vi "Demo.vi"() -> ()   [LabVIEW 2020]
uses:
  TypeDef/Plane.ctl
panel:
  out "string":string
  in  "current lon":string="-79.541260"
  in  "current lat":string="40.286792"
  in  "Current Map":refnum<k7>(container)
  out "Airplanes":T1[](array[typedef])
  out "Raw data":string[][](array[string])
  in  "Airplane":T1
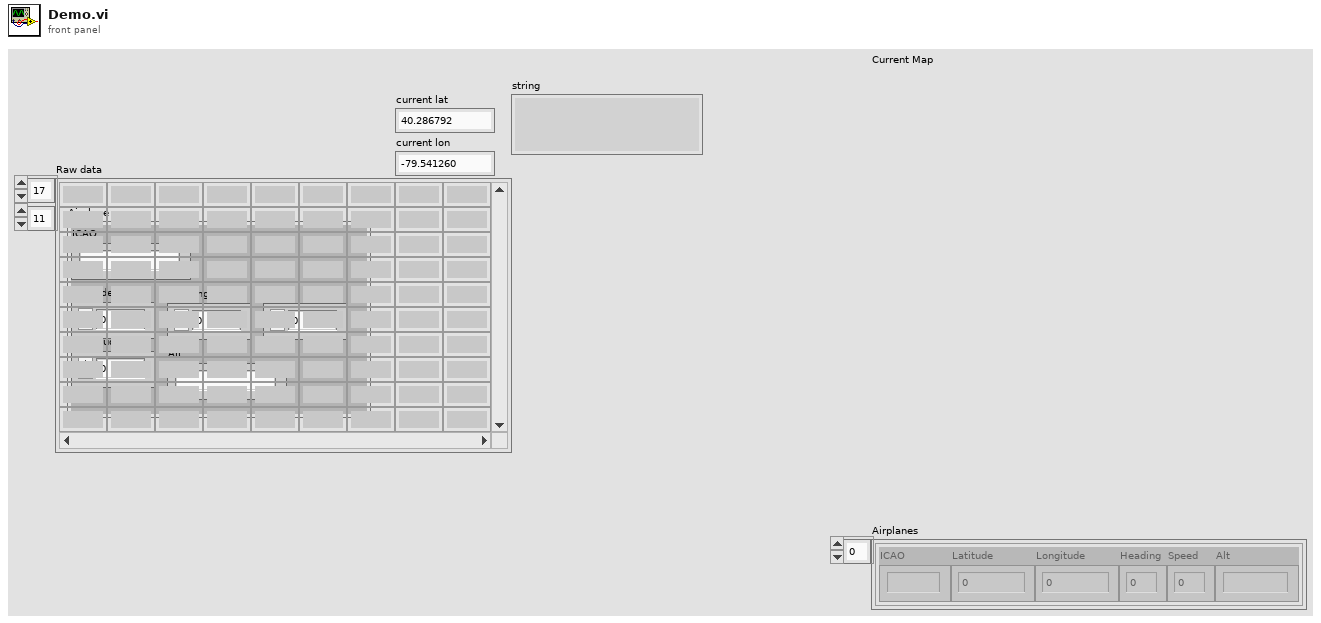
[diagram p1: front panel]
types:
  T1 = typedef "Plane.ctl" = cluster{"ICAO":string, "Latitude":dbl, "Longitude":dbl, "Heading":dbl, "Speed":dbl, "Alt":string}
  T2 = cluster{"ViewerLat":string, "ViewerLong":string, "ViewerAlt":string, "ViewerHDG":string, "Viewerpitch":string}
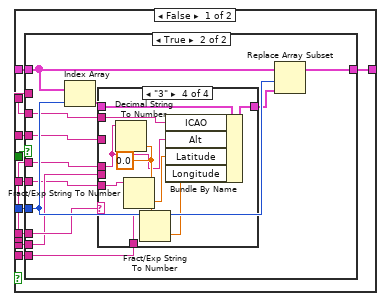
[diagram p6: hidden frame]
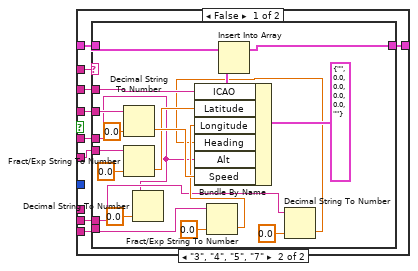
[diagram p7: hidden frame]
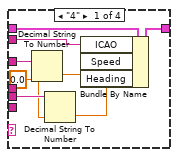
[diagram p9: hidden frame]
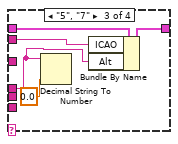
[diagram p11: hidden frame]
diagram:
  (unwired) ",{\"longitude\":0.000000,\"latitude\":0.000000,\"height\":,\"ICAO\":A05514},{\"longitude\":-79.645510,\"latitude\":39.757100,\"height\":39000,\"ICAO\":A4DD8F}" ("string")
  (unwired) "&markers=&markers=icon:https://icons.iconarchive.com/icons/unclebob/spanish-travel/24/plane-icon.png|40.366792,-80.261260" ("string")
  (unwired) "&markers=icon:https://icons.iconarchive.com/icons/unclebob/spanish-travel/24/plane-icon.png|" ("string")
  (unwired) "&markers=icon:https://icons.iconarchive.com/icons/ahmadhania/spherical/64/airplane-icon.png|" ("string")
  (unwired) "&markers=icon:https://icons.iconarchive.com/icons/graphicloads/folded/24/plane-folded-icon.png|" ("string")
  (unwired) "&markers=icon:https://icons.iconarchive.com/icons/papirus-team/papirus-status/24/airplane-mode-icon.png|" ("string")
  (unwired) "&markers=icon:\"file:///C:/Users/Kaitie/Downloads/aeroplane64.png\"%7C" ("string")
  (unwired) string[][] [["MSG", "7", "111", "11111", "ABAE62", "111111", "2021/06/30", "12:22:06.169", "2021/06/30", "12:22:06.150", "", "36000", "", "", "", "", "", "", "", "", "", "0"], ["MSG", "8", "111", "11111", "ABAE62", "111111", "2021/06/30", "12:22:06.346", "2021/06/30", "12:22:06.346", "", "", "", "", "", "", "", "", "", "", "", "0"], ["MSG", "8", "111", "11111", "ABAE62", "111111", "2021/06/30", "12:22:06.506", "2021/06/30", "12:22:06.478", "", "", "", "", "", "", "", "", "", "", "", "0"], ["MSG", "8", "111", "11111", "ABAE62", "111111", "2021/06/30", "12:22:06.515", "2021/06/30", "12:22:06.479", "", "", "", "", "", "", "", "", "", "", "", "0"], ["MSG", "7", "111", "11111", "ABAE62", "111111", "2021/06/30", "12:22:06.556", "2021/06/30", "12:22:06.543", "", "36000", "", "", "", "", "", "", "", "", "", "0"], ["MSG", "8", "111", "11111", "ABAE62", "111111", "2021/06/30", "12:22:07.101", "2021/06/30", "12:22:07.070", "", "", "", "", "", "", "", "", "", "", "", "0"], ["MSG", "7", "111", "11111", "ABAE62", "111111", "2021/06/30", "12:22:07.289", "2021/06/30", "12:22:07.264", "", "36000", "", "", "", "", "", "", "", "", "", "0"], ["MSG", "7", "111", "11111", "ABAE62", "111111", "2021/06/30", "12:22:07.451", "2021/06/30", "12:22:07.395", "", "36000", "", "", "", "", "", "", "", "", "", "0"], ["MSG", "8", "111", "11111", "ABAE62", "111111", "2021/06/30", "12:22:07.568", "2021/06/30", "12:22:07.527", "", "", "", "", "", "", "", "", "", "", "", "0"], ["MSG", "8", "111", "11111", "ABAE62", "111111", "2021/06/30", "12:22:07.578", "2021/06/30", "12:22:07.528", "", "", "", "", "", "", "", "", "", "", "", "0"], ["MSG", "8", "111", "11111", "ABAE62", "111111", "2021/06/30", "12:22:07.830", "2021/06/30", "12:22:07.789", "", "", "", "", "", "", "", "", "", "", "", "0"], ["MSG", "3", "111", "11111", "ABAE62", "111111", "2021/06/30", "12:22:07.997", "2021/06/30", "12:22:07.985", "", "36000", "", "", "40.36748", "-80.25311", "", "", "", "", "", "0"], ["MSG", "8", "111", "11111", "ABAE62", "111111", "2021/06/30", "12:22:08.045", "2021/06/30", "12:22:07.987", "", "", "", "", "", "", "", "", "", "", "", "0"], ["MSG", "8", "111", "11111", "ABAE62", "111111", "2021/06/30", "12:22:08.188", "2021/06/30", "12:22:08.181", "", "", "", "", "", "", "", "", "", "", "", "0"], ["MSG", "8", "111", "11111", "ABAE62", "111111", "2021/06/30", "12:22:08.197", "2021/06/30", "12:22:08.181", "", "", "", "", "", "", "", "", "", "", "", "0"], ["MSG", "7", "111", "11111", "ABAE62", "111111", "2021/06/30", "12:22:08.339", "2021/06/30", "12:22:08.315", "", "36000", "", "", "", "", "", "", "", "", "", "0"], ["MSG", "8", "111", "11111", "ABAE62", "111111", "2021/06/30", "12:22:09.700", "2021/06/30", "12:22:09.689", "", "", "", "", "", "", "", "", "", "", "", "0"], ["MSG", "8", "111", "11111", "ABAE62", "111111", "2021/06/30", "12:22:09.709", "2021/06/30", "12:22:09.689", "", "", "", "", "", "", "", "", "", "", "", "0"], ["MSG", "8", "111", "11111", "ABAE62", "111111", "2021/06/30", "12:22:10.016", "2021/06/30", "12:22:10.016", "", "", "", "", "", "", "", "", "", "", "", "0"], ["MSG", "3", "111", "11111", "ABAE62", "111111", "2021/06/30", "12:22:10.242", "2021/06/30", "12:22:10.214", "", "36000", "", "", "40.36833", "-80.25893", "", "", "", "", "", "0"], ["MSG", "8", "111", "11111", "ABAE62", "111111", "2021/06/30", "12:22:10.368", "2021/06/30", "12:22:10.345", "", "", "", "", "", "", "", "", "", "", "", "0"], ["MSG", "8", "111", "11111", "ABAE62", "111111", "2021/06/30", "12:22:10.602", "2021/06/30", "12:22:10.542", "", "", "", "", "", "", "", "", "", "", "", "0"], ["MSG", "4", "111", "11111", "ABAE62", "111111", "2021/06/30", "12:22:10.703", "2021/06/30", "12:22:10.672", "", "", "437", "281", "", "", "64", "", "", "", "", "0"], ["MSG", "8", "111", "11111", "ABAE62", "111111", "2021/06/30", "12:22:10.942", "2021/06/30", "12:22:10.934", "", "", "", "", "", "", "", "", "", "", "", "0"], ["MSG", "4", "111", "11111", "ABAE62", "111111", "2021/06/30", "12:22:11.735", "2021/06/30", "12:22:11.720", "", "", "437", "281", "", "", "64", "", "", "", "", "0"], ["MSG", "8", "111", "11111", "ABAE62", "111111", "2021/06/30", "12:22:11.902", "2021/06/30", "12:22:11.853", "", "", "", "", "", "", "", "", "", "", "", "0"], ["MSG", "7", "111", "11111", "ABAE62", "111111", "2021/06/30", "12:22:12.170", "2021/06/30", "12:22:12.114", "", "36000", "", "", "", "", "", "", "", "", "", "0"], ["MSG", "8", "111", "11111", "AE0144", "111111", "2021/06/30", "12:22:12.729", "2021/06/30", "12:22:12.704", "", "", "", "", "", "", "", "", "", "", "", "0"], ["MSG", "7", "111", "11111", "AE0144", "111111", "2021/06/30", "12:22:12.797", "2021/06/30", "12:22:12.769", "", "20000", "", "", "", "", "", "", "", "", "", "0"], ["MSG", "7", "111", "11111", "AE0144", "111111", "2021/06/30", "12:22:12.993", "2021/06/30", "12:22:12.966", "", "20000", "", "", "", "", "", "", "", "", "", "0"], ["MSG", "5", "111", "11111", "AE0144", "111111", "2021/06/30", "12:22:13.264", "2021/06/30", "12:22:13.229", "", "20000", "", "", "", "", "", "", "0", "", "0", "0"], ["MSG", "3", "111", "11111", "ABAE62", "111111", "2021/06/30", "12:22:14.038", "2021/06/30", "12:22:14.014", "", "36000", "", "", "40.36977", "-80.26880", "", "", "", "", "", "0"], ["MSG", "5", "111", "11111", "ABAE62", "111111", "2021/06/30", "12:22:14.427", "2021/06/30", "12:22:14.408", "", "36000", "", "", "", "", "", "", "0", "", "0", "0"], ["MSG", "7", "111", "11111", "ABAE62", "111111", "2021/06/30", "12:22:14.859", "2021/06/30", "12:22:14.801", "", "36000", "", "", "", "", "", "", "", "", "", "0"], ["MSG", "8", "111", "11111", "ABAE62", "111111", "2021/06/30", "12:22:14.994", "2021/06/30", "12:22:14.933", "", "", "", "", "", "", "", "", "", "", "", "0"], ["MSG", "8", "111", "11111", "ABAE62", "111111", "2021/06/30", "12:22:15.009", "2021/06/30", "12:22:15.000", "", "", "", "", "", "", "", "", "", "", "", "0"], ["MSG", "8", "111", "11111", "AE0144", "111111", "2021/06/30", "12:22:15.116", "2021/06/30", "12:22:15.064", "", "", "", "", "", "", "", "", "", "", "", "0"], ["MSG", "7", "111", "11111", "ABAE62", "111111", "2021/06/30", "12:22:15.147", "2021/06/30", "12:22:15.128", "", "36000", "", "", "", "", "", "", "", "", "", "0"], ["MSG", "7", "111", "11111", "ABAE62", "111111", "2021/06/30", "12:22:15.405", "2021/06/30", "12:22:15.391", "", "36000", "", "", "", "", "", "", "", "", "", "0"], ["MSG", "8", "111", "11111", "ABAE62", "111111", "2021/06/30", "12:22:15.533", "2021/06/30", "12:22:15.522", "", "", "", "", "", "", "", "", "", "", "", "0"], ["MSG", "8", "111", "11111", "ABAE62", "111111", "2021/06/30", "12:22:15.553", "2021/06/30", "12:22:15.523", "", "", "", "", "", "", "", "", "", "", "", "0"], ["MSG", "7", "111", "11111", "ABAE62", "111111", "2021/06/30", "12:22:15.718", "2021/06/30", "12:22:15.717", "", "36000", "", "", "", "", "", "", "", "", "", "0"]] ("Raw data 2")
  (unwired) "&markers=size:tiny" ("string")
  (unwired) "&markers=color:blue%7Clabel:S%7C" ("string")
  (unwired) "&markers=icon:https://goo.gl/5y3S82|" ("string")
  (unwired) string[][] [["MSG", "4", "111", "11111", "A99703", "111111", "2021/06/30", "01:33:22.831", "2021/06/30", "01:33:22.770", "", "", "213", "266", "", "", "-896", "", "", "", "", "0"], ["MSG", "8", "111", "11111", "A99703", "111111", "2021/06/30", "01:33:23.619", "2021/06/30", "01:33:23.558", "", "", "", "", "", "", "", "", "", "", "", "0"], ["MSG", "3", "111", "11111", "A99703", "111111", "2021/06/30", "01:33:23.658", "2021/06/30", "01:33:23.621", "", "3475", "", "", "40.35814", "-79.71923", "", "", "", "", "", "0"], ["MSG", "4", "111", "11111", "A99703", "111111", "2021/06/30", "01:33:23.760", "2021/06/30", "01:33:23.752", "", "", "213", "266", "", "", "-832", "", "", "", "", "0"], ["MSG", "3", "111", "11111", "A99703", "111111", "2021/06/30", "01:33:24.622", "2021/06/30", "01:33:24.605", "", "3475", "", "", "40.35805", "-79.72052", "", "", "", "", "", "0"], ["MSG", "4", "111", "11111", "A99703", "111111", "2021/06/30", "01:33:24.693", "2021/06/30", "01:33:24.672", "", "", "213", "266", "", "", "-832", "", "", "", "", "0"], ["MSG", "4", "111", "11111", "A99703", "111111", "2021/06/30", "01:33:25.696", "2021/06/30", "01:33:25.654", "", "", "213", "266", "", "", "-768", "", "", "", "", "0"], ["MSG", "1", "111", "11111", "A99703", "111111", "2021/06/30", "01:33:25.766", "2021/06/30", "01:33:25.720", "N717KV  ", "", "", "", "", "", "", "", "", "", "", "0"], ["MSG", "8", "111", "11111", "A99703", "111111", "2021/06/30", "01:33:25.849", "2021/06/30", "01:33:25.850", "", "", "", "", "", "", "", "", "", "", "", "0"], ["MSG", "5", "111", "11111", "A99703", "111111", "2021/06/30", "01:33:26.437", "2021/06/30", "01:33:26.375", "", "345", "", "", "", "", "", "", "", "", "", ""]] ("array")
  w27 = "," ("string")
  (unwired) "https://maps.googleapis.com/maps/api/staticmap?center=Brooklyn+Bridge,New+York,NY&zoom=13&size=600x300&maptype=roadmap\n&markers=color:blue%7Clabel:S%7C40.702147,-74.015794&markers=color:green%7Clabel:G%7C40.711614,-74.012318\n&markers=color:red%7Clabel:C%7C40.718217,-73.998284\n&key=AIzaSyBLVIRyOFRoOpmuxChHO5QT5_7M34SwGWA" ("URL")
  (unwired) string[][] [["MSG", "4", "111", "11111", "A05514", "111111", "2021/06/30", "01:06:18.351", "2021/06/30", "01:06:18.304", "", "", "272", "127", "", "", "0", "", "", "", "", "0"], ["MSG", "8", "111", "11111", "A4DD8F", "111111", "2021/06/30", "01:06:18.874", "2021/06/30", "01:06:18.827", "", "", "", "", "", "", "", "", "", "", "", "0"], ["MSG", "5", "111", "11111", "A4DD8F", "111111", "2021/06/30", "01:06:18.962", "2021/06/30", "01:06:18.957", "", "5000", "", "", "", "", "", "", "0", "", "0", "0"], ["MSG", "5", "111", "11111", "A4DD8F", "111111", "2021/06/30", "01:06:19.109", "2021/06/30", "01:06:19.088", "", "5000", "", "", "", "", "", "", "0", "", "0", "0"], ["MSG", "3", "111", "11111", "A4DD8F", "111111", "2021/06/30", "01:06:19.169", "2021/06/30", "01:06:19.153", "", "5000", "", "", "39.75710", "-79.64551", "", "", "", "", "", "0"], ["MSG", "4", "111", "11111", "A4DD8F", "111111", "2021/06/30", "01:06:19.218", "2021/06/30", "01:06:19.155", "", "", "450", "104", "", "", "0", "", "", "", "", "0"], ["MSG", "8", "111", "11111", "A4DD8F", "111111", "2021/06/30", "01:06:19.628", "2021/06/30", "01:06:19.612", "", "", "", "", "", "", "", "", "", "", "", "0"], ["MSG", "8", "111", "11111", "A4DD8F", "111111", "2021/06/30", "01:06:19.638", "2021/06/30", "01:06:19.613", "", "", "", "", "", "", "", "", "", "", "", "0"], ["MSG", "8", "111", "11111", "A4DD8F", "111111", "2021/06/30", "01:06:19.656", "2021/06/30", "01:06:19.614", "", "", "", "", "", "", "", "", "", "", "", "0"], ["MSG", "8", "111", "11111", "A4DD8F", "111111", "2021/06/30", "01:06:19.669", "2021/06/30", "01:06:19.614", "", "", "", "", "", "", "", "", "", "", "", "0"], ["MSG", "5", "111", "11111", "A4DD8F", "111111", "", "", "", "", "", "", "", "", "", "", "", "", "", "", "", ""]] ("array")
  # "Microsoft Windows [Version 10.0.19042.1052]\n(c) Microsoft Corporation. All rights reserved.\n\nC:\\Data\\dump1090-win.1.10.3010.14>dump1090.exe --interactive --net --net-beast --net-http-port 8081\n-----------------------------------------------------------------------------\n|                        dump1090 ModeS Receiver         Ver : 1.10.3010.14 |\n-----------------------------------------------------------------------------\n\n Copyright (C) 2012 by Salvatore Sanfilippo <antirez@gmail.com>\n Copyright (C) 2014 by Malcolm Robb <support@attavionics.com>\n\n All rights reserved.\n\n THIS SOFTWARE IS PROVIDED BY THE COPYRIGHT HOLDERS AND CONTRIBUTORS\n AS IS AND ANY EXPRESS OR IMPLIED WARRANTIES, INCLUDING, BUT NOT\n LIMITED TO, THE IMPLIED WARRANTIES OF MERCHANTABILITY AND FITNESS FOR\n A PARTICULAR PURPOSE ARE DISCLAIMED. IN NO EVENT SHALL THE COPYRIGHT\n HOLDER OR CONTRIBUTORS BE LIABLE FOR ANY DIRECT, INDIRECT, INCIDENTAL,\n SPECIAL, EXEMPLARY, OR CONSEQUENTIAL DAMAGES (INCLUDING, BUT NOT\n LIMITED TO, PROCUREMENT OF SUBSTITUTE GOODS OR SERVICES; LOSS OF USE,\n DATA, OR PROFITS; OR BUSINESS INTERRUPTION) HOWEVER CAUSED AND ON ANY\n THEORY OF LIABILITY, WHETHER IN CONTRACT, STRICT LIABILITY, OR TORT\n (INCLUDING NEGLIGENCE OR OTHERWISE) ARISING IN ANY WAY OUT OF THE USE\n OF THIS SOFTWARE, EVEN IF ADVISED OF THE POSSIBILITY OF SUCH DAMAGE.\n\n For further details refer to <https://github.com/MalcolmRobb/dump1090>\n\nHex     Mode  Sqwk  Flight   Alt    Spd  Hdg    Lat      Long   Sig  Msgs   Ti/\n-------------------------------------------------------------------------------\nHex     Mode  Sqwk  Flight   Alt    Spd  Hdg    Lat      Long   Sig  Msgs   Ti-\n-------------------------------------------------------------------------------\nHex     Mode  Sqwk  Flight   Alt    Spd  Hdg    Lat      Long   Sig  Msgs   Ti-\n-------------------------------------------------------------------------------\nHex     Mode  Sqwk  Flight   Alt    Spd  Hdg    Lat      Long   Sig  Msgs   Ti-\n-------------------------------------------------------------------------------\nHex     Mode  Sqwk  Flight   Alt    Spd  Hdg    Lat      Long   Sig  Msgs   Ti-\n-------------------------------------------------------------------------------\nHex     Mode  Sqwk  Flight   Alt    Spd  Hdg    Lat      Long   Sig  Msgs   Ti\\\n-------------------------------------------------------------------------------\nHex     Mode  Sqwk  Flight   Alt    Spd  Hdg    Lat      Long   Sig  Msgs   Ti\\\n-------------------------------------------------------------------------------\nHex     Mode  Sqwk  Flight   Alt    Spd  Hdg    Lat      Long   Sig  Msgs   Ti\\\n-------------------------------------------------------------------------------\nHex     Mode  Sqwk  Flight   Alt    Spd  Hdg    Lat      Long   Sig  Msgs   Ti\\\n-------------------------------------------------------------------------------\nHex     Mode  Sqwk  Flight   Alt    Spd  Hdg    Lat      Long   Sig  Msgs   Ti|\n-------------------------------------------------------------------------------\nHex     Mode  Sqwk  Flight   Alt    Spd  Hdg    Lat      Long   Sig  Msgs   Ti|\n-------------------------------------------------------------------------------\nHex     Mode  Sqwk  Flight   Alt    Spd  Hdg    Lat      Long   Sig  Msgs   Ti|\n-------------------------------------------------------------------------------\nHex     Mode  Sqwk  Flight   Alt    Spd  Hdg    Lat      Long   Sig  Msgs   Ti|\n-------------------------------------------------------------------------------\nHex     Mode  Sqwk  Flight   Alt    Spd  Hdg    Lat      Long   Sig  Msgs   Ti/\n-------------------------------------------------------------------------------\nHex     Mode  Sqwk  Flight   Alt    Spd  Hdg    Lat      Long   Sig  Msgs   Ti/\n-------------------------------------------------------------------------------\nHex     Mode  Sqwk  Flight   Alt    Spd  Hdg    Lat      Long   Sig  Msgs   Ti/\n-------------------------------------------------------------------------------\nHex     Mode  Sqwk  Flight   Alt    Spd  Hdg    Lat      Long   Sig  Msgs   Ti/\n-------------------------------------------------------------------------------\nHex     Mode  Sqwk  Flight   Alt    Spd  Hdg    Lat      Long   Sig  Msgs   Ti-\n-------------------------------------------------------------------------------\nHex     Mode  Sqwk  Flight   Alt    Spd  Hdg    Lat      Long   Sig  Msgs   Ti-\n-------------------------------------------------------------------------------\nHex     Mode  Sqwk  Flight   Alt    Spd  Hdg    Lat      Long   Sig  Msgs   Ti-\n-------------------------------------------------------------------------------\nHex     Mode  Sqwk  Flight   Alt    Spd  Hdg    Lat      Long   Sig  Msgs   Ti\\\n-------------------------------------------------------------------------------\nHex     Mode  Sqwk  Flight   Alt    Spd  Hdg    Lat      Long   Sig  Msgs   Ti\\\n-------------------------------------------------------------------------------\nHex     Mode  Sqwk  Flight   Alt    Spd  Hdg    Lat      Long   Sig  Msgs   Ti\\\n-------------------------------------------------------------------------------\nHex     Mode  Sqwk  Flight   Alt    Spd  Hdg    Lat      Long   Sig  Msgs   Ti\\\n-------------------------------------------------------------------------------\nHex     Mode  Sqwk  Flight   Alt    Spd  Hdg    Lat      Long   Sig  Msgs   Ti|\n-------------------------------------------------------------------------------\nHex     Mode  Sqwk  Flight   Alt    Spd  Hdg    Lat      Long   Sig  Msgs   Ti|\n-------------------------------------------------------------------------------\nHex     Mode  Sqwk  Flight   Alt    Spd  Hdg    Lat      Long   Sig  Msgs   Ti|\n-------------------------------------------------------------------------------\nHex     Mode  Sqwk  Flight   Alt    Spd  Hdg    Lat      Long   Sig  Msgs   Ti|\n-------------------------------------------------------------------------------\nHex     Mode  Sqwk  Flight   Alt    Spd  Hdg    Lat      Long   Sig  Msgs   Ti/\n-------------------------------------------------------------------------------\nHex     Mode  Sqwk  Flight   Alt    Spd  Hdg    Lat      Long   Sig  Msgs   Ti/\n-------------------------------------------------------------------------------\nHex     Mode  Sqwk  Flight   Alt    Spd  Hdg    Lat      Long   Sig  Msgs   Ti/\n-------------------------------------------------------------------------------\nHex     Mode  Sqwk  Flight   Alt    Spd  Hdg    Lat      Long   Sig  Msgs   Ti/\n-------------------------------------------------------------------------------\nHex     Mode  Sqwk  Flight   Alt    Spd  Hdg    Lat      Long   Sig  Msgs   Ti-\n-------------------------------------------------------------------------------\nHex     Mode  Sqwk  Flight   Alt    Spd  Hdg    Lat      Long   Sig  Msgs   Ti-\n-------------------------------------------------------------------------------\nHex     Mode  Sqwk  Flight   Alt    Spd  Hdg    Lat      Long   Sig  Msgs   Ti-\n-------------------------------------------------------------------------------\nHex     Mode  Sqwk  Flight   Alt    Spd  Hdg    Lat      Long   Sig  Msgs   Ti-\n-------------------------------------------------------------------------------\nHex     Mode  Sqwk  Flight   Alt    Spd  Hdg    Lat      Long   Sig  Msgs   Ti\\\n-------------------------------------------------------------------------------\nHex     Mode  Sqwk  Flight   Alt    Spd  Hdg    Lat      Long   Sig  Msgs   Ti\\\n-------------------------------------------------------------------------------\nHex     Mode  Sqwk  Flight   Alt    Spd  Hdg    Lat      Long   Sig  Msgs   Ti\\\n-------------------------------------------------------------------------------\nHex     Mode  Sqwk  Flight   Alt    Spd  Hdg    Lat      Long   Sig  Msgs   Ti\\\n-------------------------------------------------------------------------------\nHex     Mode  Sqwk  Flight   Alt    Spd  Hdg    Lat      Long   Sig  Msgs   Ti|\n-------------------------------------------------------------------------------\nHex     Mode  Sqwk  Flight   Alt    Spd  Hdg    Lat      Long   Sig  Msgs   Ti|\n-------------------------------------------------------------------------------\nHex     Mode  Sqwk  Flight   Alt    Spd  Hdg    Lat      Long   Sig  Msgs   Ti|\n-------------------------------------------------------------------------------\nHex     Mode  Sqwk  Flight   Alt    Spd  Hdg    Lat      Long   Sig  Msgs   Ti/\n-------------------------------------------------------------------------------\nHex     Mode  Sqwk  Flight   Alt    Spd  Hdg    Lat      Long   Sig  Msgs   Ti/\n-------------------------------------------------------------------------------\nHex     Mode  Sqwk  Flight   Alt    Spd  Hdg    Lat      Long   Sig  Msgs   Ti/\n-------------------------------------------------------------------------------\nHex     Mode  Sqwk  Flight   Alt    Spd  Hdg    Lat      Long   Sig  Msgs   Ti/\n-------------------------------------------------------------------------------\nHex     Mode  Sqwk  Flight   Alt    Spd  Hdg    Lat      Long   Sig  Msgs   Ti-\n-------------------------------------------------------------------------------\nHex     Mode  Sqwk  Flight   Alt    Spd  Hdg    Lat      Long   Sig  Msgs   Ti-\n-------------------------------------------------------------------------------\nHex     Mode  Sqwk  Flight   Alt    Spd  Hdg    Lat      Long   Sig  Msgs   Ti-\n-------------------------------------------------------------------------------\nHex     Mode  Sqwk  Flight   Alt    Spd  Hdg    Lat      Long   Sig  Msgs   Ti-\n-------------------------------------------------------------------------------\nHex     Mode  Sqwk  Flight   Alt    Spd  Hdg    Lat      Long   Sig  Msgs   Ti\\\n-------------------------------------------------------------------------------\nHex     Mode  Sqwk  Flight   Alt    Spd  Hdg    Lat      Long   Sig  Msgs   Ti\\\n-------------------------------------------------------------------------------\nHex     Mode  Sqwk  Flight   Alt    Spd  Hdg    Lat      Long   Sig  Msgs   Ti\\\n-------------------------------------------------------------------------------\nHex     Mode  Sqwk  Flight   Alt    Spd  Hdg    Lat      Long   Sig  Msgs   Ti\\\n-------------------------------------------------------------------------------\nHex     Mode  Sqwk  Flight   Alt    Spd  Hdg    Lat      Long   Sig  Msgs   Ti|\n-------------------------------------------------------------------------------\nHex     Mode  Sqwk  Flight   Alt    Spd  Hdg    Lat      Long   Sig  Msgs   Ti|\n-------------------------------------------------------------------------------\nHex     Mode  Sqwk  Flight   Alt    Spd  Hdg    Lat      Long   Sig  Msgs   Ti|\n-------------------------------------------------------------------------------\nHex     Mode  Sqwk  Flight   Alt    Spd  Hdg    Lat      Long   Sig  Msgs   Ti|\n-------------------------------------------------------------------------------\nHex     Mode  Sqwk  Flight   Alt    Spd  Hdg    Lat      Long   Sig  Msgs   Ti/\n-------------------------------------------------------------------------------\nHex     Mode  Sqwk  Flight   Alt    Spd  Hdg    Lat      Long   Sig  Msgs   Ti/\n-------------------------------------------------------------------------------\nHex     Mode  Sqwk  Flight   Alt    Spd  Hdg    Lat      Long   Sig  Msgs   Ti/\n-------------------------------------------------------------------------------\nHex     Mode  Sqwk  Flight   Alt    Spd  Hdg    Lat      Long   Sig  Msgs   Ti-\n-------------------------------------------------------------------------------\nHex     Mode  Sqwk  Flight   Alt    Spd  Hdg    Lat      Long   Sig  Msgs   Ti-\n-------------------------------------------------------------------------------\nHex     Mode  Sqwk  Flight   Alt    Spd  Hdg    Lat      Long   Sig  Msgs   Ti-\n-------------------------------------------------------------------------------\nHex     Mode  Sqwk  Flight   Alt    Spd  Hdg    Lat      Long   Sig  Msgs   Ti-\n-------------------------------------------------------------------------------\nHex     Mode  Sqwk  Flight   Alt    Spd  Hdg    Lat      Long   Sig  Msgs   Ti\\\n-------------------------------------------------------------------------------\nHex     Mode  Sqwk  Flight   Alt    Spd  Hdg    Lat      Long   Sig  Msgs   Ti\\\n-------------------------------------------------------------------------------\nHex     Mode  Sqwk  Flight   Alt    Spd  Hdg    Lat      Long   Sig  Msgs   Ti\\\n-------------------------------------------------------------------------------\nHex     Mode  Sqwk  Flight   Alt    Spd  Hdg    Lat      Long   Sig  Msgs   Ti\\\n-------------------------------------------------------------------------------\nHex     Mode  Sqwk  Flight   Alt    Spd  Hdg    Lat      Long   Sig  Msgs   Ti|\n-------------------------------------------------------------------------------\nHex     Mode  Sqwk  Flight   Alt    Spd  Hdg    Lat      Long   Sig  Msgs   Ti|\n-------------------------------------------------------------------------------\nHex     Mode  Sqwk  Flight   Alt    Spd  Hdg    Lat      Long   Sig  Msgs   Ti|\n-------------------------------------------------------------------------------\nHex     Mode  Sqwk  Flight   Alt    Spd  Hdg    Lat      Long   Sig  Msgs   Ti|\n-------------------------------------------------------------------------------\nHex     Mode  Sqwk  Flight   Alt    Spd  Hdg    Lat      Long   Sig  Msgs   Ti/\n-------------------------------------------------------------------------------\nHex     Mode  Sqwk  Flight   Alt    Spd  Hdg    Lat      Long   Sig  Msgs   Ti/\n-------------------------------------------------------------------------------\nHex     Mode  Sqwk  Flight   Alt    Spd  Hdg    Lat      Long   Sig  Msgs   Ti/\n-------------------------------------------------------------------------------\nHex     Mode  Sqwk  Flight   Alt    Spd  Hdg    Lat      Long   Sig  Msgs   Ti/\n-------------------------------------------------------------------------------\nHex     Mode  Sqwk  Flight   Alt    Spd  Hdg    Lat      Long   Sig  Msgs   Ti-\n-------------------------------------------------------------------------------\nHex     Mode  Sqwk  Flight   Alt    Spd  Hdg    Lat      Long   Sig  Msgs   Ti-\n-------------------------------------------------------------------------------\nHex     Mode  Sqwk  Flight   Alt    Spd  Hdg    Lat      Long   Sig  Msgs   Ti-\n-------------------------------------------------------------------------------\nHex     Mode  Sqwk  Flight   Alt    Spd  Hdg    Lat      Long   Sig  Msgs   Ti-\n-------------------------------------------------------------------------------\nHex     Mode  Sqwk  Flight   Alt    Spd  Hdg    Lat      Long   Sig  Msgs   Ti\\\n-------------------------------------------------------------------------------\nHex     Mode  Sqwk  Flight   Alt    Spd  Hdg    Lat      Long   Sig  Msgs   Ti\\\n-------------------------------------------------------------------------------\nHex     Mode  Sqwk  Flight   Alt    Spd  Hdg    Lat      Long   Sig  Msgs   Ti\\\n-------------------------------------------------------------------------------\nHex     Mode  Sqwk  Flight   Alt    Spd  Hdg    Lat      Long   Sig  Msgs   Ti|\n-------------------------------------------------------------------------------\nHex     Mode  Sqwk  Flight   Alt    Spd  Hdg    Lat      Long   Sig  Msgs   Ti|\n-------------------------------------------------------------------------------\nHex     Mode  Sqwk  Flight   Alt    Spd  Hdg    Lat      Long   Sig  Msgs   Ti|\n-------------------------------------------------------------------------------\nHex     Mode  Sqwk  Flight   Alt    Spd  Hdg    Lat      Long   Sig  Msgs   Ti|\n-------------------------------------------------------------------------------\nHex     Mode  Sqwk  Flight   Alt    Spd  Hdg    Lat      Long   Sig  Msgs   Ti/\n-------------------------------------------------------------------------------\nHex     Mode  Sqwk  Flight   Alt    Spd  Hdg    Lat      Long   Sig  Msgs   Ti/\n-------------------------------------------------------------------------------\nHex     Mode  Sqwk  Flight   Alt    Spd  Hdg    Lat      Long   Sig  Msgs   Ti/\n-------------------------------------------------------------------------------\nHex     Mode  Sqwk  Flight   Alt    Spd  Hdg    Lat      Long   Sig  Msgs   Ti/\n-------------------------------------------------------------------------------\nHex     Mode  Sqwk  Flight   Alt    Spd  Hdg    Lat      Long   Sig  Msgs   Ti-\n-------------------------------------------------------------------------------\nHex     Mode  Sqwk  Flight   Alt    Spd  Hdg    Lat      Long   Sig  Msgs   Ti-\n-------------------------------------------------------------------------------\nHex     Mode  Sqwk  Flight   Alt    Spd  Hdg    Lat      Long   Sig  Msgs   Ti-\n-------------------------------------------------------------------------------\nHex     Mode  Sqwk  Flight   Alt    Spd  Hdg    Lat      Long   Sig  Msgs   Ti-\n-------------------------------------------------------------------------------\nHex     Mode  Sqwk  Flight   Alt    Spd  Hdg    Lat      Long   Sig  Msgs   Ti\\\n-------------------------------------------------------------------------------\nHex     Mode  Sqwk  Flight   Alt    Spd  Hdg    Lat      Long   Sig  Msgs   Ti\\\n-------------------------------------------------------------------------------\nHex     Mode  Sqwk  Flight   Alt    Spd  Hdg    Lat      Long   Sig  Msgs   Ti\\\n-------------------------------------------------------------------------------\nHex     Mode  Sqwk  Flight   Alt    Spd  Hdg    Lat      Long   Sig  Msgs   Ti\\\n-------------------------------------------------------------------------------\nHex     Mode  Sqwk  Flight   Alt    Spd  Hdg    Lat      Long   Sig  Msgs   Ti|\n-------------------------------------------------------------------------------\nHex     Mode  Sqwk  Flight   Alt    Spd  Hdg    Lat      Long   Sig  Msgs   Ti|\n-------------------------------------------------------------------------------\nHex     Mode  Sqwk  Flight   Alt    Spd  Hdg    Lat      Long   Sig  Msgs   Ti|\n-------------------------------------------------------------------------------\nHex     Mode  Sqwk  Flight   Alt    Spd  Hdg    Lat      Long   Sig  Msgs   Ti/\n-------------------------------------------------------------------------------\nHex     Mode  Sqwk  Flight   Alt    Spd  Hdg    Lat      Long   Sig  Msgs   Ti/\n-------------------------------------------------------------------------------\nHex     Mode  Sqwk  Flight   Alt    Spd  Hdg    Lat      Long   Sig  Msgs   Ti/\n-------------------------------------------------------------------------------\nHex     Mode  Sqwk  Flight   Alt    Spd  Hdg    Lat      Long   Sig  Msgs   Ti/\n-------------------------------------------------------------------------------\nHex     Mode  Sqwk  Flight   Alt    Spd  Hdg    Lat      Long   Sig  Msgs   Ti-\n-------------------------------------------------------------------------------\nHex     Mode  Sqwk  Flight   Alt    Spd  Hdg    Lat      Long   Sig  Msgs   Ti-\n-------------------------------------------------------------------------------\nHex     Mode  Sqwk  Flight   Alt    Spd  Hdg    Lat      Long   Sig  Msgs   Ti-\n-------------------------------------------------------------------------------\nHex     Mode  Sqwk  Flight   Alt    Spd  Hdg    Lat      Long   Sig  Msgs   Ti-\n-------------------------------------------------------------------------------\nHex     Mode  Sqwk  Flight   Alt    Spd  Hdg    Lat      Long   Sig  Msgs   Ti\\\n-------------------------------------------------------------------------------\nHex     Mode  Sqwk  Flight   Alt    Spd  Hdg    Lat      Long   Sig  Msgs   Ti\\\n-------------------------------------------------------------------------------\nHex     Mode  Sqwk  Flight   Alt    Spd  Hdg    Lat      Long   Sig  Msgs   Ti\\\n-------------------------------------------------------------------------------\nHex     Mode  Sqwk  Flight   Alt    Spd  Hdg    Lat      Long   Sig  Msgs   Ti\\\n-------------------------------------------------------------------------------\nHex     Mode  Sqwk  Flight   Alt    Spd  Hdg    Lat      Long   Sig  Msgs   Ti|\n-------------------------------------------------------------------------------\nHex     Mode  Sqwk  Flight   Alt    Spd  Hdg    Lat      Long   Sig  Msgs   Ti|\n-------------------------------------------------------------------------------\nHex     Mode  Sqwk  Flight   Alt    Spd  Hdg    Lat      Long   Sig  Msgs   Ti|\n-------------------------------------------------------------------------------\nHex     Mode  Sqwk  Flight   Alt    Spd  Hdg    Lat      Long   Sig  Msgs   Ti|\n-------------------------------------------------------------------------------\nHex     Mode  Sqwk  Flight   Alt    Spd  Hdg    Lat      Long   Sig  Msgs   Ti/\n-------------------------------------------------------------------------------\nHex     Mode  Sqwk  Flight   Alt    Spd  Hdg    Lat      Long   Sig  Msgs   Ti/\n-------------------------------------------------------------------------------\nHex     Mode  Sqwk  Flight   Alt    Spd  Hdg    Lat      Long   Sig  Msgs   Ti/\n-------------------------------------------------------------------------------\nHex     Mode  Sqwk  Flight   Alt    Spd  Hdg    Lat      Long   Sig  Msgs   Ti-\n-------------------------------------------------------------------------------\nHex     Mode  Sqwk  Flight   Alt    Spd  Hdg    Lat      Long   Sig  Msgs   Ti-\n-------------------------------------------------------------------------------\nHex     Mode  Sqwk  Flight   Alt    Spd  Hdg    Lat      Long   Sig  Msgs   Ti-\n-------------------------------------------------------------------------------\nHex     Mode  Sqwk  Flight   Alt    Spd  Hdg    Lat      Long   Sig  Msgs   Ti-\n-------------------------------------------------------------------------------\nHex     Mode  Sqwk  Flight   Alt    Spd  Hdg    Lat      Long   Sig  Msgs   Ti\\\n-------------------------------------------------------------------------------\nHex     Mode  Sqwk  Flight   Alt    Spd  Hdg    Lat      Long   Sig  Msgs   Ti\\\n-------------------------------------------------------------------------------\nHex     Mode  Sqwk  Flight   Alt    Spd  Hdg    Lat      Long   Sig  Msgs   Ti\\\n-------------------------------------------------------------------------------\nHex     Mode  Sqwk  Flight   Alt    Spd  Hdg    Lat      Long   Sig  Msgs   Ti\\\n-------------------------------------------------------------------------------\nHex     Mode  Sqwk  Flight   Alt    Spd  Hdg    Lat      Long   Sig  Msgs   Ti|\n-------------------------------------------------------------------------------\nHex     Mode  Sqwk  Flight   Alt    Spd  Hdg    Lat      Long   Sig  Msgs   Ti|\n-------------------------------------------------------------------------------\nHex     Mode  Sqwk  Flight   Alt    Spd  Hdg    Lat      Long   Sig  Msgs   Ti|\n-------------------------------------------------------------------------------\nHex     Mode  Sqwk  Flight   Alt    Spd  Hdg    Lat      Long   Sig  Msgs   Ti|\n-------------------------------------------------------------------------------\nHex     Mode  Sqwk  Flight   Alt    Spd  Hdg    Lat      Long   Sig  Msgs   Ti/\n-------------------------------------------------------------------------------\nHex     Mode  Sqwk  Flight   Alt    Spd  Hdg    Lat      Long   Sig  Msgs   Ti/\n-------------------------------------------------------------------------------\nHex     Mode  Sqwk  Flight   Alt    Spd  Hdg    Lat      Long   Sig  Msgs   Ti/\n-------------------------------------------------------------------------------\nHex     Mode  Sqwk  Flight   Alt    Spd  Hdg    Lat      Long   Sig  Msgs   Ti/\n-------------------------------------------------------------------------------\nHex     Mode  Sqwk  Flight   Alt    Spd  Hdg    Lat      Long   Sig  Msgs   Ti-\n-------------------------------------------------------------------------------\nHex     Mode  Sqwk  Flight   Alt    Spd  Hdg    Lat      Long   Sig  Msgs   Ti-\n-------------------------------------------------------------------------------\nHex     Mode  Sqwk  Flight   Alt    Spd  Hdg    Lat      Long   Sig  Msgs   Ti-\n-------------------------------------------------------------------------------\nHex     Mode  Sqwk  Flight   Alt    Spd  Hdg    Lat      Long   Sig  Msgs   Ti-\n-------------------------------------------------------------------------------\nHex     Mode  Sqwk  Flight   Alt    Spd  Hdg    Lat      Long   Sig  Msgs   Ti\\\n-------------------------------------------------------------------------------\nHex     Mode  Sqwk  Flight   Alt    Spd  Hdg    Lat      Long   Sig  Msgs   Ti\\\n-------------------------------------------------------------------------------\nHex     Mode  Sqwk  Flight   Alt    Spd  Hdg    Lat      Long   Sig  Msgs   Ti\\\n-------------------------------------------------------------------------------\nHex     Mode  Sqwk  Flight   Alt    Spd  Hdg    Lat      Long   Sig  Msgs   Ti|\n-------------------------------------------------------------------------------\nHex     Mode  Sqwk  Flight   Alt    Spd  Hdg    Lat      Long   Sig  Msgs   Ti|\n-------------------------------------------------------------------------------\nHex     Mode  Sqwk  Flight   Alt    Spd  Hdg    Lat      Long   Sig  Msgs   Ti|\n-------------------------------------------------------------------------------\nHex     Mode  Sqwk  Flight   Alt    Spd  Hdg    Lat      Long   Sig  Msgs   Ti|\n-------------------------------------------------------------------------------\nHex     Mode  Sqwk  Flight   Alt    Spd  Hdg    Lat      Long   Sig  Msgs   Ti/\n-------------------------------------------------------------------------------\nHex     Mode  Sqwk  Flight   Alt    Spd  Hdg    Lat      Long   Sig  Msgs   Ti/\n-------------------------------------------------------------------------------\nHex     Mode  Sqwk  Flight   Alt    Spd  Hdg    Lat      Long   Sig  Msgs   Ti/\n-------------------------------------------------------------------------------\nHex     Mode  Sqwk  Flight   Alt    Spd  Hdg    Lat      Long   Sig  Msgs   Ti/\n-------------------------------------------------------------------------------\nHex     Mode  Sqwk  Flight   Alt    Spd  Hdg    Lat      Long   Sig  Msgs   Ti-\n-------------------------------------------------------------------------------\nHex     Mode  Sqwk  Flight   Alt    Spd  Hdg    Lat      Long   Sig  Msgs   Ti-\n-------------------------------------------------------------------------------\nHex     Mode  Sqwk  Flight   Alt    Spd  Hdg    Lat      Long   Sig  Msgs   Ti-\n-------------------------------------------------------------------------------\nHex     Mode  Sqwk  Flight   Alt    Spd  Hdg    Lat      Long   Sig  Msgs   Ti-\n-------------------------------------------------------------------------------\nHex     Mode  Sqwk  Flight   Alt    Spd  Hdg    Lat      Long   Sig  Msgs   Ti\\\n-------------------------------------------------------------------------------\nHex     Mode  Sqwk  Flight   Alt    Spd  Hdg    Lat      Long   Sig  Msgs   Ti\\\n-------------------------------------------------------------------------------\nHex     Mode  Sqwk  Flight   Alt    Spd  Hdg    Lat      Long   Sig  Msgs   Ti\\\n-------------------------------------------------------------------------------\nHex     Mode  Sqwk  Flight   Alt    Spd  Hdg    Lat      Long   Sig  Msgs   Ti\\\n-------------------------------------------------------------------------------\nHex     Mode  Sqwk  Flight   Alt    Spd  Hdg    Lat      Long   Sig  Msgs   Ti|\n-------------------------------------------------------------------------------\nHex     Mode  Sqwk  Flight   Alt    Spd  Hdg    Lat      Long   Sig  Msgs   Ti|\n-------------------------------------------------------------------------------\nHex     Mode  Sqwk  Flight   Alt    Spd  Hdg    Lat      Long   Sig  Msgs   Ti|\n-------------------------------------------------------------------------------\nHex     Mode  Sqwk  Flight   Alt    Spd  Hdg    Lat      Long   Sig  Msgs   Ti/\n-------------------------------------------------------------------------------\nHex     Mode  Sqwk  Flight   Alt    Spd  Hdg    Lat      Long   Sig  Msgs   Ti/\n-------------------------------------------------------------------------------\nHex     Mode  Sqwk  Flight   Alt    Spd  Hdg    Lat      Long   Sig  Msgs   Ti/\n-------------------------------------------------------------------------------\nHex     Mode  Sqwk  Flight   Alt    Spd  Hdg    Lat      Long   Sig  Msgs   Ti/\n-------------------------------------------------------------------------------\nHex     Mode  Sqwk  Flight   Alt    Spd  Hdg    Lat      Long   Sig  Msgs   Ti-\n-------------------------------------------------------------------------------\nHex     Mode  Sqwk  Flight   Alt    Spd  Hdg    Lat      Long   Sig  Msgs   Ti-\n-------------------------------------------------------------------------------\nHex     Mode  Sqwk  Flight   Alt    Spd  Hdg    Lat      Long   Sig  Msgs   Ti-\n-------------------------------------------------------------------------------\nHex     Mode  Sqwk  Flight   Alt    Spd  Hdg    Lat      Long   Sig  Msgs   Ti-\n-------------------------------------------------------------------------------\nHex     Mode  Sqwk  Flight   Alt    Spd  Hdg    Lat      Long   Sig  Msgs   Ti\\\n-------------------------------------------------------------------------------\nHex     Mode  Sqwk  Flight   Alt    Spd  Hdg    Lat      Long   Sig  Msgs   Ti\\\n-------------------------------------------------------------------------------\nHex     Mode  Sqwk  Flight   Alt    Spd  Hdg    Lat      Long   Sig  Msgs   Ti\\\n-------------------------------------------------------------------------------\nHex     Mode  Sqwk  Flight   Alt    Spd  Hdg    Lat      Long   Sig  Msgs   Ti\\\n-------------------------------------------------------------------------------\nHex     Mode  Sqwk  Flight   Alt    Spd  Hdg    Lat      Long   Sig  Msgs   Ti|\n-------------------------------------------------------------------------------\nHex     Mode  Sqwk  Flight   Alt    Spd  Hdg    Lat      Long   Sig  Msgs   Ti|\n-------------------------------------------------------------------------------\nHex     Mode  Sqwk  Flight   Alt    Spd  Hdg    Lat      Long   Sig  Msgs   Ti|\n-------------------------------------------------------------------------------\nHex     Mode  Sqwk  Flight   Alt    Spd  Hdg    Lat      Long   Sig  Msgs   Ti|\n-------------------------------------------------------------------------------\nHex     Mode  Sqwk  Flight   Alt    Spd  Hdg    Lat      Long   Sig  Msgs   Ti/\n-------------------------------------------------------------------------------\nHex     Mode  Sqwk  Flight   Alt    Spd  Hdg    Lat      Long   Sig  Msgs   Ti/\n-------------------------------------------------------------------------------\nHex     Mode  Sqwk  Flight   Alt    Spd  Hdg    Lat      Long   Sig  Msgs   Ti/\n-------------------------------------------------------------------------------\nHex     Mode  Sqwk  Flight   Alt    Spd  Hdg    Lat      Long   Sig  Msgs   Ti/\n-------------------------------------------------------------------------------\nHex     Mode  Sqwk  Flight   Alt    Spd  Hdg    Lat      Long   Sig  Msgs   Ti-\n-------------------------------------------------------------------------------\nHex     Mode  Sqwk  Flight   Alt    Spd  Hdg    Lat      Long   Sig  Msgs   Ti-\n-------------------------------------------------------------------------------\nHex     Mode  Sqwk  Flight   Alt    Spd  Hdg    Lat      Long   Sig  Msgs   Ti-\n-------------------------------------------------------------------------------\nHex     Mode  Sqwk  Flight   Alt    Spd  Hdg    Lat      Long   Sig  Msgs   Ti\\\n-------------------------------------------------------------------------------\nHex     Mode  Sqwk  Flight   Alt    Spd  Hdg    Lat      Long   Sig  Msgs   Ti\\\n-------------------------------------------------------------------------------\nHex     Mode  Sqwk  Flight   Alt    Spd  Hdg    Lat      Long   Sig  Msgs   Ti\\\n-------------------------------------------------------------------------------\nHex     Mode  Sqwk  Flight   Alt    Spd  Hdg    Lat      Long   Sig  Msgs   Ti\\\n-------------------------------------------------------------------------------\nHex     Mode  Sqwk  Flight   Alt    Spd  Hdg    Lat      Long   Sig  Msgs   Ti|\n-------------------------------------------------------------------------------\nHex     Mode  Sqwk  Flight   Alt    Spd  Hdg    Lat      Long   Sig  Msgs   Ti|\n-------------------------------------------------------------------------------\nHex     Mode  Sqwk  Flight   Alt    Spd  Hdg    Lat      Long   Sig  Msgs   Ti|\n-------------------------------------------------------------------------------\nHex     Mode  Sqwk  Flight   Alt    Spd  Hdg    Lat      Long   Sig  Msgs   Ti|\n-------------------------------------------------------------------------------\nHex     Mode  Sqwk  Flight   Alt    Spd  Hdg    Lat      Long   Sig  Msgs   Ti/\n-------------------------------------------------------------------------------\nHex     Mode  Sqwk  Flight   Alt    Spd  Hdg    Lat      Long   Sig  Msgs   Ti/\n-------------------------------------------------------------------------------\nHex     Mode  Sqwk  Flight   Alt    Spd  Hdg    Lat      Long   Sig  Msgs   Ti/\n-------------------------------------------------------------------------------\nHex     Mode  Sqwk  Flight   Alt    Spd  Hdg    Lat      Long   Sig  Msgs   Ti/\n-------------------------------------------------------------------------------\nHex     Mode  Sqwk  Flight   Alt    Spd  Hdg    Lat      Long   Sig  Msgs   Ti-\n-------------------------------------------------------------------------------\nHex     Mode  Sqwk  Flight   Alt    Spd  Hdg    Lat      Long   Sig  Msgs   Ti-\n-------------------------------------------------------------------------------\nHex     Mode  Sqwk  Flight   Alt    Spd  Hdg    Lat      Long   Sig  Msgs   Ti-\n-------------------------------------------------------------------------------\nHex     Mode  Sqwk  Flight   Alt    Spd  Hdg    Lat      Long   Sig  Msgs   Ti\\\n-------------------------------------------------------------------------------\nHex     Mode  Sqwk  Flight   Alt    Spd  Hdg    Lat      Long   Sig  Msgs   Ti\\\n-------------------------------------------------------------------------------\nHex     Mode  Sqwk  Flight   Alt    Spd  Hdg    Lat      Long   Sig  Msgs   Ti\\\n-------------------------------------------------------------------------------\nHex     Mode  Sqwk  Flight   Alt    Spd  Hdg    Lat      Long   Sig  Msgs   Ti\\\n-------------------------------------------------------------------------------\nHex     Mode  Sqwk  Flight   Alt    Spd  Hdg    Lat      Long   Sig  Msgs   Ti|\n-------------------------------------------------------------------------------\nHex     Mode  Sqwk  Flight   Alt    Spd  Hdg    Lat      Long   Sig  Msgs   Ti|\n-------------------------------------------------------------------------------\nHex     Mode  Sqwk  Flight   Alt    Spd  Hdg    Lat      Long   Sig  Msgs   Ti|\n-------------------------------------------------------------------------------\nHex     Mode  Sqwk  Flight   Alt    Spd  Hdg    Lat      Long   Sig  Msgs   Ti|\n-------------------------------------------------------------------------------\nHex     Mode  Sqwk  Flight   Alt    Spd  Hdg    Lat      Long   Sig  Msgs   Ti/\n-------------------------------------------------------------------------------\nHex     Mode  Sqwk  Flight   Alt    Spd  Hdg    Lat      Long   Sig  Msgs   Ti/\n-------------------------------------------------------------------------------\nHex     Mode  Sqwk  Flight   Alt    Spd  Hdg    Lat      Long   Sig  Msgs   Ti/\n-------------------------------------------------------------------------------\nHex     Mode  Sqwk  Flight   Alt    Spd  Hdg    Lat      Long   Sig  Msgs   Ti/\n-------------------------------------------------------------------------------\nHex     Mode  Sqwk  Flight   Alt    Spd  Hdg    Lat      Long   Sig  Msgs   Ti-\n-------------------------------------------------------------------------------\nHex     Mode  Sqwk  Flight   Alt    Spd  Hdg    Lat      Long   Sig  Msgs   Ti-\n-------------------------------------------------------------------------------\nHex     Mode  Sqwk  Flight   Alt    Spd  Hdg    Lat      Long   Sig  Msgs   Ti-\n-------------------------------------------------------------------------------\nHex     Mode  Sqwk  Flight   Alt    Spd  Hdg    Lat      Long   Sig  Msgs   Ti-\n-------------------------------------------------------------------------------\nHex     Mode  Sqwk  Flight   Alt    Spd  Hdg    Lat      Long   Sig  Msgs   Ti\\\n-------------------------------------------------------------------------------\nHex     Mode  Sqwk  Flight   Alt    Spd  Hdg    Lat      Long   Sig  Msgs   Ti\\\n-------------------------------------------------------------------------------\nHex     Mode  Sqwk  Flight   Alt    Spd  Hdg    Lat      Long   Sig  Msgs   Ti\\\n-------------------------------------------------------------------------------\nHex     Mode  Sqwk  Flight   Alt    Spd  Hdg    Lat      Long   Sig  Msgs   Ti|\n-------------------------------------------------------------------------------\nHex     Mode  Sqwk  Flight   Alt    Spd  Hdg    Lat      Long   Sig  Msgs   Ti|\n-------------------------------------------------------------------------------\nHex     Mode  Sqwk  Flight   Alt    Spd  Hdg    Lat      Long   Sig  Msgs   Ti|\n-------------------------------------------------------------------------------\nHex     Mode  Sqwk  Flight   Alt    Spd  Hdg    Lat      Long   Sig  Msgs   Ti|\n-------------------------------------------------------------------------------\nHex     Mode  Sqwk  Flight   Alt    Spd  Hdg    Lat      Long   Sig  Msgs   Ti/\n-------------------------------------------------------------------------------\nHex     Mode  Sqwk  Flight   Alt    Spd  Hdg    Lat      Long   Sig  Msgs   Ti/\n-------------------------------------------------------------------------------\nHex     Mode  Sqwk  Flight   Alt    Spd  Hdg    Lat      Long   Sig  Msgs   Ti/\n-------------------------------------------------------------------------------\nHex     Mode  Sqwk  Flight   Alt    Spd  Hdg    Lat      Long   Sig  Msgs   Ti/\n-------------------------------------------------------------------------------\nHex     Mode  Sqwk  Flight   Alt    Spd  Hdg    Lat      Long   Sig  Msgs   Ti-\n-------------------------------------------------------------------------------\nHex     Mode  Sqwk  Flight   Alt    Spd  Hdg    Lat      Long   Sig  Msgs   Ti-\n-------------------------------------------------------------------------------\nHex     Mode  Sqwk  Flight   Alt    Spd  Hdg    Lat      Long   Sig  Msgs   Ti-\n-------------------------------------------------------------------------------\nHex     Mode  Sqwk  Flight   Alt    Spd  Hdg    Lat      Long   Sig  Msgs   Ti-\n-------------------------------------------------------------------------------\nHex     Mode  Sqwk  Flight   Alt    Spd  Hdg    Lat      Long   Sig  Msgs   Ti\\\n-------------------------------------------------------------------------------\nHex     Mode  Sqwk  Flight   Alt    Spd  Hdg    Lat      Long   Sig  Msgs   Ti\\\n-------------------------------------------------------------------------------\nHex     Mode  Sqwk  Flight   Alt    Spd  Hdg    Lat      Long   Sig  Msgs   Ti\\\n-------------------------------------------------------------------------------\nHex     Mode  Sqwk  Flight   Alt    Spd  Hdg    Lat      Long   Sig  Msgs   Ti\\\n-------------------------------------------------------------------------------\nHex     Mode  Sqwk  Flight   Alt    Spd  Hdg    Lat      Long   Sig  Msgs   Ti|\n-------------------------------------------------------------------------------\nHex     Mode  Sqwk  Flight   Alt    Spd  Hdg    Lat      Long   Sig  Msgs   Ti|\n-------------------------------------------------------------------------------\nHex     Mode  Sqwk  Flight   Alt    Spd  Hdg    Lat      Long   Sig  Msgs   Ti|\n-------------------------------------------------------------------------------\nHex     Mode  Sqwk  Flight   Alt    Spd  Hdg    Lat      Long   Sig  Msgs   Ti/\n-------------------------------------------------------------------------------\nHex     Mode  Sqwk  Flight   Alt    Spd  Hdg    Lat      Long   Sig  Msgs   Ti/\n-------------------------------------------------------------------------------\nHex     Mode  Sqwk  Flight   Alt    Spd  Hdg    Lat      Long   Sig  Msgs   Ti/\n-------------------------------------------------------------------------------\nHex     Mode  Sqwk  Flight   Alt    Spd  Hdg    Lat      Long   Sig  Msgs   Ti/\n-------------------------------------------------------------------------------\nHex     Mode  Sqwk  Flight   Alt    Spd  Hdg    Lat      Long   Sig  Msgs   Ti-\n-------------------------------------------------------------------------------\nHex     Mode  Sqwk  Flight   Alt    Spd  Hdg    Lat      Long   Sig  Msgs   Ti-\n-------------------------------------------------------------------------------\nHex     Mode  Sqwk  Flight   Alt    Spd  Hdg    Lat      Long   Sig  Msgs   Ti-\n-------------------------------------------------------------------------------\nHex     Mode  Sqwk  Flight   Alt    Spd  Hdg    Lat      Long   Sig  Msgs   Ti-\n-------------------------------------------------------------------------------\nHex     Mode  Sqwk  Flight   Alt    Spd  Hdg    Lat      Long   Sig  Msgs   Ti\\\n-------------------------------------------------------------------------------\nHex     Mode  Sqwk  Flight   Alt    Spd  Hdg    Lat      Long   Sig  Msgs   Ti\\\n-------------------------------------------------------------------------------\nHex     Mode  Sqwk  Flight   Alt    Spd  Hdg    Lat      Long   Sig  Msgs   Ti\\\n-------------------------------------------------------------------------------\nHex     Mode  Sqwk  Flight   Alt    Spd  Hdg    Lat      Long   Sig  Msgs   Ti\\\n-------------------------------------------------------------------------------\nHex     Mode  Sqwk  Flight   Alt    Spd  Hdg    Lat      Long   Sig  Msgs   Ti|\n-------------------------------------------------------------------------------\nHex     Mode  Sqwk  Flight   Alt    Spd  Hdg    Lat      Long   Sig  Msgs   Ti|\n-------------------------------------------------------------------------------\nHex     Mode  Sqwk  Flight   Alt    Spd  Hdg    Lat      Long   Sig  Msgs   Ti|\n-------------------------------------------------------------------------------\nHex     Mode  Sqwk  Flight   Alt    Spd  Hdg    Lat      Long   Sig  Msgs   Ti|\n-------------------------------------------------------------------------------\nHex     Mode  Sqwk  Flight   Alt    Spd  Hdg    Lat      Long   Sig  Msgs   Ti/\n-------------------------------------------------------------------------------\nHex     Mode  Sqwk  Flight   Alt    Spd  Hdg    Lat      Long   Sig  Msgs   Ti/\n-------------------------------------------------------------------------------\nHex     Mode  Sqwk  Flight   Alt    Spd  Hdg    Lat      Long   Sig  Msgs   Ti/\n-------------------------------------------------------------------------------\nHex     Mode  Sqwk  Flight   Alt    Spd  Hdg    Lat      Long   Sig  Msgs   Ti/\n-------------------------------------------------------------------------------\nHex     Mode  Sqwk  Flight   Alt    Spd  Hdg    Lat      Long   Sig  Msgs   Ti-\n-------------------------------------------------------------------------------\nHex     Mode  Sqwk  Flight   Alt    Spd  Hdg    Lat      Long   Sig  Msgs   Ti-\n-------------------------------------------------------------------------------\nHex     Mode  Sqwk  Flight   Alt    Spd  Hdg    Lat      Long   Sig  Msgs   Ti-\n-------------------------------------------------------------------------------\nHex     Mode  Sqwk  Flight   Alt    Spd  Hdg    Lat      Long   Sig  Msgs   Ti\\\n-------------------------------------------------------------------------------\nHex     Mode  Sqwk  Flight   Alt    Spd  Hdg    Lat      Long   Sig  Msgs   Ti\\\n-------------------------------------------------------------------------------\nHex     Mode  Sqwk  Flight   Alt    Spd  Hdg    Lat      Long   Sig  Msgs   Ti\\\n-------------------------------------------------------------------------------\nHex     Mode  Sqwk  Flight   Alt    Spd  Hdg    Lat      Long   Sig  Msgs   Ti\\\n-------------------------------------------------------------------------------\nHex     Mode  Sqwk  Flight   Alt    Spd  Hdg    Lat      Long   Sig  Msgs   Ti|\n-------------------------------------------------------------------------------\nHex     Mode  Sqwk  Flight   Alt    Spd  Hdg    Lat      Long   Sig  Msgs   Ti|\n-------------------------------------------------------------------------------\nHex     Mode  Sqwk  Flight   Alt    Spd  Hdg    Lat      Long   Sig  Msgs   Ti|\n-------------------------------------------------------------------------------\nHex     Mode  Sqwk  Flight   Alt    Spd  Hdg    Lat      Long   Sig  Msgs   Ti|\n-------------------------------------------------------------------------------\nHex     Mode  Sqwk  Flight   Alt    Spd  Hdg    Lat      Long   Sig  Msgs   Ti/\n-------------------------------------------------------------------------------\nHex     Mode  Sqwk  Flight   Alt    Spd  Hdg    Lat      Long   Sig  Msgs   Ti/\n-------------------------------------------------------------------------------\nHex     Mode  Sqwk  Flight   Alt    Spd  Hdg    Lat      Long   Sig  Msgs   Ti/\n-------------------------------------------------------------------------------\nHex     Mode  Sqwk  Flight   Alt    Spd  Hdg    Lat      Long   Sig  Msgs   Ti/\n-------------------------------------------------------------------------------\nHex     Mode  Sqwk  Flight   Alt    Spd  Hdg    Lat      Long   Sig  Msgs   Ti-\n-------------------------------------------------------------------------------\nHex     Mode  Sqwk  Flight   Alt    Spd  Hdg    Lat      Long   Sig  Msgs   Ti-\n-------------------------------------------------------------------------------\nHex     Mode  Sqwk  Flight   Alt    Spd  Hdg    Lat      Long   Sig  Msgs   Ti-\n-------------------------------------------------------------------------------\nHex     Mode  Sqwk  Flight   Alt    Spd  Hdg    Lat      Long   Sig  Msgs   Ti-\n-------------------------------------------------------------------------------\nHex     Mode  Sqwk  Flight   Alt    Spd  Hdg    Lat      Long   Sig  Msgs   Ti\\\n-------------------------------------------------------------------------------\nHex     Mode  Sqwk  Flight   Alt    Spd  Hdg    Lat      Long   Sig  Msgs   Ti\\\n-------------------------------------------------------------------------------\nHex     Mode  Sqwk  Flight   Alt    Spd  Hdg    Lat      Long   Sig  Msgs   Ti\\\n-------------------------------------------------------------------------------\nHex     Mode  Sqwk  Flight   Alt    Spd  Hdg    Lat      Long   Sig  Msgs   Ti|\n-------------------------------------------------------------------------------\nHex     Mode  Sqwk  Flight   Alt    Spd  Hdg    Lat      Long   Sig  Msgs   Ti|\n-------------------------------------------------------------------------------\nHex     Mode  Sqwk  Flight   Alt    Spd  Hdg    Lat      Long   Sig  Msgs   Ti|\n-------------------------------------------------------------------------------\nHex     Mode  Sqwk  Flight   Alt    Spd  Hdg    Lat      Long   Sig  Msgs   Ti|\n-------------------------------------------------------------------------------\nHex     Mode  Sqwk  Flight   Alt    Spd  Hdg    Lat      Long   Sig  Msgs   Ti/\n-------------------------------------------------------------------------------\nHex     Mode  Sqwk  Flight   Alt    Spd  Hdg    Lat      Long   Sig  Msgs   Ti/\n-------------------------------------------------------------------------------\nHex     Mode  Sqwk  Flight   Alt    Spd  Hdg    Lat      Long   Sig  Msgs   Ti/\n-------------------------------------------------------------------------------\nHex     Mode  Sqwk  Flight   Alt    Spd  Hdg    Lat      Long   Sig  Msgs   Ti/\n-------------------------------------------------------------------------------\nHex     Mode  Sqwk  Flight   Alt    Spd  Hdg    Lat      Long   Sig  Msgs   Ti-\n-------------------------------------------------------------------------------\nHex     Mode  Sqwk  Flight   Alt    Spd  Hdg    Lat      Long   Sig  Msgs   Ti-\n-------------------------------------------------------------------------------\nHex     Mode  Sqwk  Flight   Alt    Spd  Hdg    Lat      Long   Sig  Msgs   Ti-\n-------------------------------------------------------------------------------\nHex     Mode  Sqwk  Flight   Alt    Spd  Hdg    Lat      Long   Sig  Msgs   Ti-\n-------------------------------------------------------------------------------\nHex     Mode  Sqwk  Flight   Alt    Spd  Hdg    Lat      Long   Sig  Msgs   Ti\\\n-------------------------------------------------------------------------------\nHex     Mode  Sqwk  Flight   Alt    Spd  Hdg    Lat      Long   Sig  Msgs   Ti\\\n-------------------------------------------------------------------------------\nHex     Mode  Sqwk  Flight   Alt    Spd  Hdg    Lat      Long   Sig  Msgs   Ti\\\n-------------------------------------------------------------------------------\nHex     Mode  Sqwk  Flight   Alt    Spd  Hdg    Lat      Long   Sig  Msgs   Ti\\\n-------------------------------------------------------------------------------\nHex     Mode  Sqwk  Flight   Alt    Spd  Hdg    Lat      Long   Sig  Msgs   Ti|\n-------------------------------------------------------------------------------\nHex     Mode  Sqwk  Flight   Alt    Spd  Hdg    Lat      Long   Sig  Msgs   Ti|\n-------------------------------------------------------------------------------\nHex     Mode  Sqwk  Flight   Alt    Spd  Hdg    Lat      Long   Sig  Msgs   Ti|\n-------------------------------------------------------------------------------\nHex     Mode  Sqwk  Flight   Alt    Spd  Hdg    Lat      Long   Sig  Msgs   Ti|\n-------------------------------------------------------------------------------\nHex     Mode  Sqwk  Flight   Alt    Spd  Hdg    Lat      Long   Sig  Msgs   Ti/\n-------------------------------------------------------------------------------\nHex     Mode  Sqwk  Flight   Alt    Spd  Hdg    Lat      Long   Sig  Msgs   Ti/\n-------------------------------------------------------------------------------\nHex     Mode  Sqwk  Flight   Alt    Spd  Hdg    Lat      Long   Sig  Msgs   Ti/\n-------------------------------------------------------------------------------\nHex     Mode  Sqwk  Flight   Alt    Spd  Hdg    Lat      Long   Sig  Msgs   Ti-\n-------------------------------------------------------------------------------\nHex     Mode  Sqwk  Flight   Alt    Spd  Hdg    Lat      Long   Sig  Msgs   Ti-\n-------------------------------------------------------------------------------\nHex     Mode  Sqwk  Flight   Alt    Spd  Hdg    Lat      Long   Sig  Msgs   Ti-\n-------------------------------------------------------------------------------\nHex     Mode  Sqwk  Flight   Alt    Spd  Hdg    Lat      Long   Sig  Msgs   Ti-\n-------------------------------------------------------------------------------\nHex     Mode  Sqwk  Flight   Alt    Spd  Hdg    Lat      Long   Sig  Msgs   Ti\\\n-------------------------------------------------------------------------------\nHex     Mode  Sqwk  Flight   Alt    Spd  Hdg    Lat      Long   Sig  Msgs   Ti\\\n-------------------------------------------------------------------------------\nHex     Mode  Sqwk  Flight   Alt    Spd  Hdg    Lat      Long   Sig  Msgs   Ti\\\n-------------------------------------------------------------------------------\nHex     Mode  Sqwk  Flight   Alt    Spd  Hdg    Lat      Long   Sig  Msgs   Ti\\\n-------------------------------------------------------------------------------\nHex     Mode  Sqwk  Flight   Alt    Spd  Hdg    Lat      Long   Sig  Msgs   Ti|\n-------------------------------------------------------------------------------\nHex     Mode  Sqwk  Flight   Alt    Spd  Hdg    Lat      Long   Sig  Msgs   Ti|\n-------------------------------------------------------------------------------\nHex     Mode  Sqwk  Flight   Alt    Spd  Hdg    Lat      Long   Sig  Msgs   Ti|\n-------------------------------------------------------------------------------\nHex     Mode  Sqwk  Flight   Alt    Spd  Hdg    Lat      Long   Sig  Msgs   Ti|\n-------------------------------------------------------------------------------\nHex     Mode  Sqwk  Flight   Alt    Spd  Hdg    Lat      Long   Sig  Msgs   Ti/\n-------------------------------------------------------------------------------\nHex     Mode  Sqwk  Flight   Alt    Spd  Hdg    Lat      Long   Sig  Msgs   Ti/\n-------------------------------------------------------------------------------\nHex     Mode  Sqwk  Flight   Alt    Spd  Hdg    Lat      Long   Sig  Msgs   Ti/\n-------------------------------------------------------------------------------\nHex     Mode  Sqwk  Flight   Alt    Spd  Hdg    Lat      Long   Sig  Msgs   Ti/\n-------------------------------------------------------------------------------\nHex     Mode  Sqwk  Flight   Alt    Spd  Hdg    Lat      Long   Sig  Msgs   Ti-\n-------------------------------------------------------------------------------\nHex     Mode  Sqwk  Flight   Alt    Spd  Hdg    Lat      Long   Sig  Msgs   Ti-\n-------------------------------------------------------------------------------\nHex     Mode  Sqwk  Flight   Alt    Spd  Hdg    Lat      Long   Sig  Msgs   Ti-\n-------------------------------------------------------------------------------\nHex     Mode  Sqwk  Flight   Alt    Spd  Hdg    Lat      Long   Sig  Msgs   Ti\\\n-------------------------------------------------------------------------------\nHex     Mode  Sqwk  Flight   Alt    Spd  Hdg    Lat      Long   Sig  Msgs   Ti\\\n-------------------------------------------------------------------------------\nHex     Mode  Sqwk  Flight   Alt    Spd  Hdg    Lat      Long   Sig  Msgs   Ti\\\n-------------------------------------------------------------------------------\nHex     Mode  Sqwk  Flight   Alt    Spd  Hdg    Lat      Long   Sig  Msgs   Ti\\\n-------------------------------------------------------------------------------\nHex     Mode  Sqwk  Flight   Alt    Spd  Hdg    Lat      Long   Sig  Msgs   Ti|\n-------------------------------------------------------------------------------\nHex     Mode  Sqwk  Flight   Alt    Spd  Hdg    Lat      Long   Sig  Msgs   Ti|\n-------------------------------------------------------------------------------\nHex     Mode  Sqwk  Flight   Alt    Spd  Hdg    Lat      Long   Sig  Msgs   Ti|\n-------------------------------------------------------------------------------\nHex     Mode  Sqwk  Flight   Alt    Spd  Hdg    Lat      Long   Sig  Msgs   Ti|\n-------------------------------------------------------------------------------\nHex     Mode  Sqwk  Flight   Alt    Spd  Hdg    Lat      Long   Sig  Msgs   Ti/\n-------------------------------------------------------------------------------\nHex     Mode  Sqwk  Flight   Alt    Spd  Hdg    Lat      Long   Sig  Msgs   Ti/\n-------------------------------------------------------------------------------\nHex     Mode  Sqwk  Flight   Alt    Spd  Hdg    Lat      Long   Sig  Msgs   Ti/\n-------------------------------------------------------------------------------\nHex     Mode  Sqwk  Flight   Alt    Spd  Hdg    Lat      Long   Sig  Msgs   Ti/\n-------------------------------------------------------------------------------\nHex     Mode  Sqwk  Flight   Alt    Spd  Hdg    Lat      Long   Sig  Msgs   Ti-\n-------------------------------------------------------------------------------\nHex     Mode  Sqwk  Flight   Alt    Spd  Hdg    Lat      Long   Sig  Msgs   Ti-\n-------------------------------------------------------------------------------\nHex     Mode  Sqwk  Flight   Alt    Spd  Hdg    Lat      Long   Sig  Msgs   Ti-\n-------------------------------------------------------------------------------\nHex     Mode  Sqwk  Flight   Alt    Spd  Hdg    Lat      Long   Sig  Msgs   Ti-\n-------------------------------------------------------------------------------\nHex     Mode  Sqwk  Flight   Alt    Spd  Hdg    Lat      Long   Sig  Msgs   Ti\\\n-------------------------------------------------------------------------------\nHex     Mode  Sqwk  Flight   Alt    Spd  Hdg    Lat      Long   Sig  Msgs   Ti\\\n-------------------------------------------------------------------------------\nHex     Mode  Sqwk  Flight   Alt    Spd  Hdg    Lat      Long   Sig  Msgs   Ti\\\n-------------------------------------------------------------------------------\nHex     Mode  Sqwk  Flight   Alt    Spd  Hdg    Lat      Long   Sig  Msgs   Ti|\n-------------------------------------------------------------------------------\nHex     Mode  Sqwk  Flight   Alt    Spd  Hdg    Lat      Long   Sig  Msgs   Ti|\n-------------------------------------------------------------------------------\nHex     Mode  Sqwk  Flight   Alt    Spd  Hdg    Lat      Long   Sig  Msgs   Ti|\n-------------------------------------------------------------------------------\nHex     Mode  Sqwk  Flight   Alt    Spd  Hdg    Lat      Long   Sig  Msgs   Ti|\n-------------------------------------------------------------------------------\nHex     Mode  Sqwk  Flight   Alt    Spd  Hdg    Lat      Long   Sig  Msgs   Ti/\n-------------------------------------------------------------------------------\nHex     Mode  Sqwk  Flight   Alt    Spd  Hdg    Lat      Long   Sig  Msgs   Ti/\n-------------------------------------------------------------------------------\nHex     Mode  Sqwk  Flight   Alt    Spd  Hdg    Lat      Long   Sig  Msgs   Ti/\n-------------------------------------------------------------------------------\nHex     Mode  Sqwk  Flight   Alt    Spd  Hdg    Lat      Long   Sig  Msgs   Ti/\n-------------------------------------------------------------------------------\nHex     Mode  Sqwk  Flight   Alt    Spd  Hdg    Lat      Long   Sig  Msgs   Ti-\n-------------------------------------------------------------------------------\nHex     Mode  Sqwk  Flight   Alt    Spd  Hdg    Lat      Long   Sig  Msgs   Ti-\n-------------------------------------------------------------------------------\nHex     Mode  Sqwk  Flight   Alt    Spd  Hdg    Lat      Long   Sig  Msgs   Ti-\n-------------------------------------------------------------------------------\nHex     Mode  Sqwk  Flight   Alt    Spd  Hdg    Lat      Long   Sig  Msgs   Ti-\n-------------------------------------------------------------------------------\nHex     Mode  Sqwk  Flight   Alt    Spd  Hdg    Lat      Long   Sig  Msgs   Ti\\\n-------------------------------------------------------------------------------\nHex     Mode  Sqwk  Flight   Alt    Spd  Hdg    Lat      Long   Sig  Msgs   Ti\\\n-------------------------------------------------------------------------------\nHex     Mode  Sqwk  Flight   Alt    Spd  Hdg    Lat      Long   Sig  Msgs   Ti\\\n-------------------------------------------------------------------------------\nHex     Mode  Sqwk  Flight   Alt    Spd  Hdg    Lat      Long   Sig  Msgs   Ti\\\n-------------------------------------------------------------------------------\nHex     Mode  Sqwk  Flight   Alt    Spd  Hdg    Lat      Long   Sig  Msgs   Ti|\n-------------------------------------------------------------------------------\nHex     Mode  Sqwk  Flight   Alt    Spd  Hdg    Lat      Long   Sig  Msgs   Ti|\n-------------------------------------------------------------------------------\nHex     Mode  Sqwk  Flight   Alt    Spd  Hdg    Lat      Long   Sig  Msgs   Ti|\n-------------------------------------------------------------------------------\nHex     Mode  Sqwk  Flight   Alt    Spd  Hdg    Lat      Long   Sig  Msgs   Ti|\n-------------------------------------------------------------------------------\nHex     Mode  Sqwk  Flight   Alt    Spd  Hdg    Lat      Long   Sig  Msgs   Ti/\n-------------------------------------------------------------------------------\nHex     Mode  Sqwk  Flight   Alt    Spd  Hdg    Lat      Long   Sig  Msgs   Ti/\n-------------------------------------------------------------------------------\nHex     Mode  Sqwk  Flight   Alt    Spd  Hdg    Lat      Long   Sig  Msgs   Ti/\n-------------------------------------------------------------------------------\nHex     Mode  Sqwk  Flight   Alt    Spd  Hdg    Lat      Long   Sig  Msgs   Ti-\n-------------------------------------------------------------------------------\nHex     Mode  Sqwk  Flight   Alt    Spd  Hdg    Lat      Long   Sig  Msgs   Ti-\n-------------------------------------------------------------------------------\nHex     Mode  Sqwk  Flight   Alt    Spd  Hdg    Lat      Long   Sig  Msgs   Ti-\n-------------------------------------------------------------------------------\nHex     Mode  Sqwk  Flight   Alt    Spd  Hdg    Lat      Long   Sig  Msgs   Ti-\n-------------------------------------------------------------------------------\nHex     Mode  Sqwk  Flight   Alt    Spd  Hdg    Lat      Long   Sig  Msgs   Ti\\\n-------------------------------------------------------------------------------\nHex     Mode  Sqwk  Flight   Alt    Spd  Hdg    Lat      Long   Sig  Msgs   Ti\\\n-------------------------------------------------------------------------------\nHex     Mode  Sqwk  Flight   Alt    Spd  Hdg    Lat      Long   Sig  Msgs   Ti\\\n-------------------------------------------------------------------------------\nHex     Mode  Sqwk  Flight   Alt    Spd  Hdg    Lat      Long   Sig  Msgs   Ti\\\n-------------------------------------------------------------------------------\nHex     Mode  Sqwk  Flight   Alt    Spd  Hdg    Lat      Long   Sig  Msgs   Ti|\n-------------------------------------------------------------------------------\nHex     Mode  Sqwk  Flight   Alt    Spd  Hdg    Lat      Long   Sig  Msgs   Ti|\n-------------------------------------------------------------------------------\nHex     Mode  Sqwk  Flight   Alt    Spd  Hdg    Lat      Long   Sig  Msgs   Ti|\n-------------------------------------------------------------------------------\nHex     Mode  Sqwk  Flight   Alt    Spd  Hdg    Lat      Long   Sig  Msgs   Ti|\n-------------------------------------------------------------------------------\nHex     Mode  Sqwk  Flight   Alt    Spd  Hdg    Lat      Long   Sig  Msgs   Ti/\n-------------------------------------------------------------------------------\nHex     Mode  Sqwk  Flight   Alt    Spd  Hdg    Lat      Long   Sig  Msgs   Ti/\n-------------------------------------------------------------------------------\nHex     Mode  Sqwk  Flight   Alt    Spd  Hdg    Lat      Long   Sig  Msgs   Ti/\n-------------------------------------------------------------------------------\nHex     Mode  Sqwk  Flight   Alt    Spd  Hdg    Lat      Long   Sig  Msgs   Ti/\n-------------------------------------------------------------------------------\nHex     Mode  Sqwk  Flight   Alt    Spd  Hdg    Lat      Long   Sig  Msgs   Ti-\n-------------------------------------------------------------------------------\nHex     Mode  Sqwk  Flight   Alt    Spd  Hdg    Lat      Long   Sig  Msgs   Ti-\n-------------------------------------------------------------------------------\nHex     Mode  Sqwk  Flight   Alt    Spd  Hdg    Lat      Long   Sig  Msgs   Ti-\n-------------------------------------------------------------------------------\nHex     Mode  Sqwk  Flight   Alt    Spd  Hdg    Lat      Long   Sig  Msgs   Ti\\\n-------------------------------------------------------------------------------\nHex     Mode  Sqwk  Flight   Alt    Spd  Hdg    Lat      Long   Sig  Msgs   Ti\\\n-------------------------------------------------------------------------------\nHex     Mode  Sqwk  Flight   Alt    Spd  Hdg    Lat      Long   Sig  Msgs   Ti\\\n-------------------------------------------------------------------------------\nHex     Mode  Sqwk  Flight   Alt    Spd  Hdg    Lat      Long   Sig  Msgs   Ti\\\n-------------------------------------------------------------------------------\nHex     Mode  Sqwk  Flight   Alt    Spd  Hdg    Lat      Long   Sig  Msgs   Ti|\n-------------------------------------------------------------------------------\nHex     Mode  Sqwk  Flight   Alt    Spd  Hdg    Lat      Long   Sig  Msgs   Ti|\n-------------------------------------------------------------------------------\nHex     Mode  Sqwk  Flight   Alt    Spd  Hdg    Lat      Long   Sig  Msgs   Ti|\n-------------------------------------------------------------------------------\nHex     Mode  Sqwk  Flight   Alt    Spd  Hdg    Lat      Long   Sig  Msgs   Ti|\n-------------------------------------------------------------------------------\nHex     Mode  Sqwk  Flight   Alt    Spd  Hdg    Lat      Long   Sig  Msgs   Ti/\n-------------------------------------------------------------------------------\nHex     Mode  Sqwk  Flight   Alt    Spd  Hdg    Lat      Long   Sig  Msgs   Ti/\n-------------------------------------------------------------------------------\nHex     Mode  Sqwk  Flight   Alt    Spd  Hdg    Lat      Long   Sig  Msgs   Ti/\n-------------------------------------------------------------------------------\nHex     Mode  Sqwk  Flight   Alt    Spd  Hdg    Lat      Long   Sig  Msgs   Ti/\n-------------------------------------------------------------------------------\nHex     Mode  Sqwk  Flight   Alt    Spd  Hdg    Lat      Long   Sig  Msgs   Ti-\n-------------------------------------------------------------------------------\nHex     Mode  Sqwk  Flight   Alt    Spd  Hdg    Lat      Long   Sig  Msgs   Ti-\n-------------------------------------------------------------------------------\nHex     Mode  Sqwk  Flight   Alt    Spd  Hdg    Lat      Long   Sig  Msgs   Ti-\n-------------------------------------------------------------------------------\nHex     Mode  Sqwk  Flight   Alt    Spd  Hdg    Lat      Long   Sig  Msgs   Ti-\n-------------------------------------------------------------------------------\nHex     Mode  Sqwk  Flight   Alt    Spd  Hdg    Lat      Long   Sig  Msgs   Ti\\\n-------------------------------------------------------------------------------\nHex     Mode  Sqwk  Flight   Alt    Spd  Hdg    Lat      Long   Sig  Msgs   Ti\\\n-------------------------------------------------------------------------------\nHex     Mode  Sqwk  Flight   Alt    Spd  Hdg    Lat      Long   Sig  Msgs   Ti\\\n-------------------------------------------------------------------------------\nHex     Mode  Sqwk  Flight   Alt    Spd  Hdg    Lat      Long   Sig  Msgs   Ti\\\n-------------------------------------------------------------------------------\nHex     Mode  Sqwk  Flight   Alt    Spd  Hdg    Lat      Long   Sig  Msgs   Ti|\n-------------------------------------------------------------------------------\nHex     Mode  Sqwk  Flight   Alt    Spd  Hdg    Lat      Long   Sig  Msgs   Ti|\n-------------------------------------------------------------------------------\nHex     Mode  Sqwk  Flight   Alt    Spd  Hdg    Lat      Long   Sig  Msgs   Ti|\n-------------------------------------------------------------------------------\nHex     Mode  Sqwk  Flight   Alt    Spd  Hdg    Lat      Long   Sig  Msgs   Ti/\n-------------------------------------------------------------------------------\nHex     Mode  Sqwk  Flight   Alt    Spd  Hdg    Lat      Long   Sig  Msgs   Ti/\n-------------------------------------------------------------------------------\nHex     Mode  Sqwk  Flight   Alt    Spd  Hdg    Lat      Long   Sig  Msgs   Ti/\n-------------------------------------------------------------------------------\nHex     Mode  Sqwk  Flight   Alt    Spd  Hdg    Lat      Long   Sig  Msgs   Ti/\n-------------------------------------------------------------------------------\nHex     Mode  Sqwk  Flight   Alt    Spd  Hdg    Lat      Long   Sig  Msgs   Ti-\n-------------------------------------------------------------------------------\nHex     Mode  Sqwk  Flight   Alt    Spd  Hdg    Lat      Long   Sig  Msgs   Ti-\n-------------------------------------------------------------------------------\nHex     Mode  Sqwk  Flight   Alt    Spd  Hdg    Lat      Long   Sig  Msgs   Ti-\n-------------------------------------------------------------------------------\nHex     Mode  Sqwk  Flight   Alt    Spd  Hdg    Lat      Long   Sig  Msgs   Ti-\n-------------------------------------------------------------------------------\nHex     Mode  Sqwk  Flight   Alt    Spd  Hdg    Lat      Long   Sig  Msgs   Ti\\\n-------------------------------------------------------------------------------\nHex     Mode  Sqwk  Flight   Alt    Spd  Hdg    Lat      Long   Sig  Msgs   Ti\\\n-------------------------------------------------------------------------------\nHex     Mode  Sqwk  Flight   Alt    Spd  Hdg    Lat      Long   Sig  Msgs   Ti\\\n-------------------------------------------------------------------------------\nHex     Mode  Sqwk  Flight   Alt    Spd  Hdg    Lat      Long   Sig  Msgs   Ti\\\n-------------------------------------------------------------------------------\nHex     Mode  Sqwk  Flight   Alt    Spd  Hdg    Lat      Long   Sig  Msgs   Ti|\n-------------------------------------------------------------------------------\nHex     Mode  Sqwk  Flight   Alt    Spd  Hdg    Lat      Long   Sig  Msgs   Ti|\n-------------------------------------------------------------------------------\nHex     Mode  Sqwk  Flight   Alt    Spd  Hdg    Lat      Long   Sig  Msgs   Ti|\n-------------------------------------------------------------------------------\nHex     Mode  Sqwk  Flight   Alt    Spd  Hdg    Lat      Long   Sig  Msgs   Ti|\n-------------------------------------------------------------------------------\nHex     Mode  Sqwk  Flight   Alt    Spd  Hdg    Lat      Long   Sig  Msgs   Ti/\n-------------------------------------------------------------------------------\nHex     Mode  Sqwk  Flight   Alt    Spd  Hdg    Lat      Long   Sig  Msgs   Ti/\n-------------------------------------------------------------------------------\nHex     Mode  Sqwk  Flight   Alt    Spd  Hdg    Lat      Long   Sig  Msgs   Ti/\n-------------------------------------------------------------------------------\nHex     Mode  Sqwk  Flight   Alt    Spd  Hdg    Lat      Long   Sig  Msgs   Ti-\n-------------------------------------------------------------------------------\nHex     Mode  Sqwk  Flight   Alt    Spd  Hdg    Lat      Long   Sig  Msgs   Ti-\n-------------------------------------------------------------------------------\nHex     Mode  Sqwk  Flight   Alt    Spd  Hdg    Lat      Long   Sig  Msgs   Ti-\n-------------------------------------------------------------------------------\nHex     Mode  Sqwk  Flight   Alt    Spd  Hdg    Lat      Long   Sig  Msgs   Ti-\n-------------------------------------------------------------------------------\nHex     Mode  Sqwk  Flight   Alt    Spd  Hdg    Lat      Long   Sig  Msgs   Ti\\\n-------------------------------------------------------------------------------\nHex     Mode  Sqwk  Flight   Alt    Spd  Hdg    Lat      Long   Sig  Msgs   Ti\\\n-------------------------------------------------------------------------------\nHex     Mode  Sqwk  Flight   Alt    Spd  Hdg    Lat      Long   Sig  Msgs   Ti\\\n-------------------------------------------------------------------------------\nHex     Mode  Sqwk  Flight   Alt    Spd  Hdg    Lat      Long   Sig  Msgs   Ti\\\n-------------------------------------------------------------------------------\nHex     Mode  Sqwk  Flight   Alt    Spd  Hdg    Lat      Long   Sig  Msgs   Ti|\n-------------------------------------------------------------------------------\nHex     Mode  Sqwk  Flight   Alt    Spd  Hdg    Lat      Long   Sig  Msgs   Ti|\n-------------------------------------------------------------------------------\nHex     Mode  Sqwk  Flight   Alt    Spd  Hdg    Lat      Long   Sig  Msgs   Ti|\n-------------------------------------------------------------------------------\nHex     Mode  Sqwk  Flight   Alt    Spd  Hdg    Lat      Long   Sig  Msgs   Ti|\n-------------------------------------------------------------------------------\nHex     Mode  Sqwk  Flight   Alt    Spd  Hdg    Lat      Long   Sig  Msgs   Ti/\n-------------------------------------------------------------------------------\nHex     Mode  Sqwk  Flight   Alt    Spd  Hdg    Lat      Long   Sig  Msgs   Ti/\n-------------------------------------------------------------------------------\nHex     Mode  Sqwk  Flight   Alt    Spd  Hdg    Lat      Long   Sig  Msgs   Ti/\n-------------------------------------------------------------------------------\nHex     Mode  Sqwk  Flight   Alt    Spd  Hdg    Lat      Long   Sig  Msgs   Ti/\n-------------------------------------------------------------------------------\nHex     Mode  Sqwk  Flight   Alt    Spd  Hdg    Lat      Long   Sig  Msgs   Ti-\n-------------------------------------------------------------------------------\nHex     Mode  Sqwk  Flight   Alt    Spd  Hdg    Lat      Long   Sig  Msgs   Ti-\n-------------------------------------------------------------------------------\nHex     Mode  Sqwk  Flight   Alt    Spd  Hdg    Lat      Long   Sig  Msgs   Ti-\n-------------------------------------------------------------------------------\nHex     Mode  Sqwk  Flight   Alt    Spd  Hdg    Lat      Long   Sig  Msgs   Ti\\\n-------------------------------------------------------------------------------\nHex     Mode  Sqwk  Flight   Alt    Spd  Hdg    Lat      Long   Sig  Msgs   Ti\\\n-------------------------------------------------------------------------------\nHex     Mode  Sqwk  Flight   Alt    Spd  Hdg    Lat      Long   Sig  Msgs   Ti\\\n-------------------------------------------------------------------------------\nHex     Mode  Sqwk  Flight   Alt    Spd  Hdg    Lat      Long   Sig  Msgs   Ti\\\n-------------------------------------------------------------------------------\nHex     Mode  Sqwk  Flight   Alt    Spd  Hdg    Lat      Long   Sig  Msgs   Ti|\n-------------------------------------------------------------------------------\nHex     Mode  Sqwk  Flight   Alt    Spd  Hdg    Lat      Long   Sig  Msgs   Ti|\n-------------------------------------------------------------------------------\nHex     Mode  Sqwk  Flight   Alt    Spd  Hdg    Lat      Long   Sig  Msgs   Ti|\n-------------------------------------------------------------------------------\nHex     Mode  Sqwk  Flight   Alt    Spd  Hdg    Lat      Long   Sig  Msgs   Ti|\n-------------------------------------------------------------------------------\nHex     Mode  Sqwk  Flight   Alt    Spd  Hdg    Lat      Long   Sig  Msgs   Ti/\n-------------------------------------------------------------------------------\nHex     Mode  Sqwk  Flight   Alt    Spd  Hdg    Lat      Long   Sig  Msgs   Ti/\n-------------------------------------------------------------------------------\nHex     Mode  Sqwk  Flight   Alt    Spd  Hdg    Lat      Long   Sig  Msgs   Ti/\n-------------------------------------------------------------------------------\nHex     Mode  Sqwk  Flight   Alt    Spd  Hdg    Lat      Long   Sig  Msgs   Ti/\n-------------------------------------------------------------------------------\nHex     Mode  Sqwk  Flight   Alt    Spd  Hdg    Lat      Long   Sig  Msgs   Ti-\n-------------------------------------------------------------------------------\nHex     Mode  Sqwk  Flight   Alt    Spd  Hdg    Lat      Long   Sig  Msgs   Ti-\n-------------------------------------------------------------------------------\nHex     Mode  Sqwk  Flight   Alt    Spd  Hdg    Lat      Long   Sig  Msgs   Ti-\n-------------------------------------------------------------------------------\nHex     Mode  Sqwk  Flight   Alt    Spd  Hdg    Lat      Long   Sig  Msgs   Ti-\n-------------------------------------------------------------------------------\nHex     Mode  Sqwk  Flight   Alt    Spd  Hdg    Lat      Long   Sig  Msgs   Ti\\\n-------------------------------------------------------------------------------\nHex     Mode  Sqwk  Flight   Alt    Spd  Hdg    Lat      Long   Sig  Msgs   Ti\\\n-------------------------------------------------------------------------------\nHex     Mode  Sqwk  Flight   Alt    Spd  Hdg    Lat      Long   Sig  Msgs   Ti\\\n-------------------------------------------------------------------------------\nHex     Mode  Sqwk  Flight   Alt    Spd  Hdg    Lat      Long   Sig  Msgs   Ti\\\n-------------------------------------------------------------------------------\nHex     Mode  Sqwk  Flight   Alt    Spd  Hdg    Lat      Long   Sig  Msgs   Ti|\n-------------------------------------------------------------------------------\nHex     Mode  Sqwk  Flight   Alt    Spd  Hdg    Lat      Long   Sig  Msgs   Ti|\n-------------------------------------------------------------------------------\nHex     Mode  Sqwk  Flight   Alt    Spd  Hdg    Lat      Long   Sig  Msgs   Ti|\n-------------------------------------------------------------------------------\nHex     Mode  Sqwk  Flight   Alt    Spd  Hdg    Lat      Long   Sig  Msgs   Ti/\n-------------------------------------------------------------------------------\nHex     Mode  Sqwk  Flight   Alt    Spd  Hdg    Lat      Long   Sig  Msgs   Ti/\n-------------------------------------------------------------------------------\nHex     Mode  Sqwk  Flight   Alt    Spd  Hdg    Lat      Long   Sig  Msgs   Ti/\n-------------------------------------------------------------------------------\nHex     Mode  Sqwk  Flight   Alt    Spd  Hdg    Lat      Long   Sig  Msgs   Ti/\n-------------------------------------------------------------------------------\nHex     Mode  Sqwk  Flight   Alt    Spd  Hdg    Lat      Long   Sig  Msgs   Ti-\n-------------------------------------------------------------------------------\nHex     Mode  Sqwk  Flight   Alt    Spd  Hdg    Lat      Long   Sig  Msgs   Ti-\n-------------------------------------------------------------------------------\nHex     Mode  Sqwk  Flight   Alt    Spd  Hdg    Lat      Long   Sig  Msgs   Ti-\n-------------------------------------------------------------------------------\nHex     Mode  Sqwk  Flight   Alt    Spd  Hdg    Lat      Long   Sig  Msgs   Ti-\n-------------------------------------------------------------------------------\nHex     Mode  Sqwk  Flight   Alt    Spd  Hdg    Lat      Long   Sig  Msgs   Ti\\\n-------------------------------------------------------------------------------\nHex     Mode  Sqwk  Flight   Alt    Spd  Hdg    Lat      Long   Sig  Msgs   Ti\\\n-------------------------------------------------------------------------------\nHex     Mode  Sqwk  Flight   Alt    Spd  Hdg    Lat      Long   Sig  Msgs   Ti\\\n-------------------------------------------------------------------------------\nHex     Mode  Sqwk  Flight   Alt    Spd  Hdg    Lat      Long   Sig  Msgs   Ti\\\n-------------------------------------------------------------------------------\nHex     Mode  Sqwk  Flight   Alt    Spd  Hdg    Lat      Long   Sig  Msgs   Ti|\n-------------------------------------------------------------------------------\nHex     Mode  Sqwk  Flight   Alt    Spd  Hdg    Lat      Long   Sig  Msgs   Ti|\n-------------------------------------------------------------------------------\nHex     Mode  Sqwk  Flight   Alt    Spd  Hdg    Lat      Long   Sig  Msgs   Ti|\n-------------------------------------------------------------------------------\nHex     Mode  Sqwk  Flight   Alt    Spd  Hdg    Lat      Long   Sig  Msgs   Ti|\n-------------------------------------------------------------------------------\nHex     Mode  Sqwk  Flight   Alt    Spd  Hdg    Lat      Long   Sig  Msgs   Ti/\n-------------------------------------------------------------------------------\nHex     Mode  Sqwk  Flight   Alt    Spd  Hdg    Lat      Long   Sig  Msgs   Ti/\n-------------------------------------------------------------------------------\nHex     Mode  Sqwk  Flight   Alt    Spd  Hdg    Lat      Long   Sig  Msgs   Ti/\n-------------------------------------------------------------------------------\nHex     Mode  Sqwk  Flight   Alt    Spd  Hdg    Lat      Long   Sig  Msgs   Ti-\n-------------------------------------------------------------------------------\nHex     Mode  Sqwk  Flight   Alt    Spd  Hdg    Lat      Long   Sig  Msgs   Ti-\n-------------------------------------------------------------------------------\nHex     Mode  Sqwk  Flight   Alt    Spd  Hdg    Lat      Long   Sig  Msgs   Ti-\n-------------------------------------------------------------------------------\nHex     Mode  Sqwk  Flight   Alt    Spd  Hdg    Lat      Long   Sig  Msgs   Ti-\n-------------------------------------------------------------------------------\nHex     Mode  Sqwk  Flight   Alt    Spd  Hdg    Lat      Long   Sig  Msgs   Ti\\\n-------------------------------------------------------------------------------\nHex     Mode  Sqwk  Flight   Alt    Spd  Hdg    Lat      Long   Sig  Msgs   Ti\\\n-------------------------------------------------------------------------------\nHex     Mode  Sqwk  Flight   Alt    Spd  Hdg    Lat      Long   Sig  Msgs   Ti\\\n-------------------------------------------------------------------------------\nHex     Mode  Sqwk  Flight   Alt    Spd  Hdg    Lat      Long   Sig  Msgs   Ti\\\n-------------------------------------------------------------------------------\nHex     Mode  Sqwk  Flight   Alt    Spd  Hdg    Lat      Long   Sig  Msgs   Ti|\n-------------------------------------------------------------------------------\nHex     Mode  Sqwk  Flight   Alt    Spd  Hdg    Lat      Long   Sig  Msgs   Ti|\n-------------------------------------------------------------------------------\nHex     Mode  Sqwk  Flight   Alt    Spd  Hdg    Lat      Long   Sig  Msgs   Ti|\n-------------------------------------------------------------------------------\nHex     Mode  Sqwk  Flight   Alt    Spd  Hdg    Lat      Long   Sig  Msgs   Ti|\n-------------------------------------------------------------------------------\nHex     Mode  Sqwk  Flight   Alt    Spd  Hdg    Lat      Long   Sig  Msgs   Ti/\n-------------------------------------------------------------------------------\nHex     Mode  Sqwk  Flight   Alt    Spd  Hdg    Lat      Long   Sig  Msgs   Ti/\n-------------------------------------------------------------------------------\nHex     Mode  Sqwk  Flight   Alt    Spd  Hdg    Lat      Long   Sig  Msgs   Ti/\n-------------------------------------------------------------------------------\nHex     Mode  Sqwk  Flight   Alt    Spd  Hdg    Lat      Long   Sig  Msgs   Ti/\n-------------------------------------------------------------------------------\nHex     Mode  Sqwk  Flight   Alt    Spd  Hdg    Lat      Long   Sig  Msgs   Ti-\n-------------------------------------------------------------------------------\nHex     Mode  Sqwk  Flight   Alt    Spd  Hdg    Lat      Long   Sig  Msgs   Ti-\n-------------------------------------------------------------------------------\nHex     Mode  Sqwk  Flight   Alt    Spd  Hdg    Lat      Long   Sig  Msgs   Ti-\n-------------------------------------------------------------------------------\nHex     Mode  Sqwk  Flight   Alt    Spd  Hdg    Lat      Long   Sig  Msgs   Ti-\n-------------------------------------------------------------------------------\nHex     Mode  Sqwk  Flight   Alt    Spd  Hdg    Lat      Long   Sig  Msgs   Ti\\\n-------------------------------------------------------------------------------\nHex     Mode  Sqwk  Flight   Alt    Spd  Hdg    Lat      Long   Sig  Msgs   Ti\\\n-------------------------------------------------------------------------------\nHex     Mode  Sqwk  Flight   Alt    Spd  Hdg    Lat      Long   Sig  Msgs   Ti\\\n-------------------------------------------------------------------------------\nHex     Mode  Sqwk  Flight   Alt    Spd  Hdg    Lat      Long   Sig  Msgs   Ti|\n-------------------------------------------------------------------------------\nHex     Mode  Sqwk  Flight   Alt    Spd  Hdg    Lat      Long   Sig  Msgs   Ti|\n-------------------------------------------------------------------------------\nHex     Mode  Sqwk  Flight   Alt    Spd  Hdg    Lat      Long   Sig  Msgs   Ti|\n-------------------------------------------------------------------------------\nHex     Mode  Sqwk  Flight   Alt    Spd  Hdg    Lat      Long   Sig  Msgs   Ti|\n-------------------------------------------------------------------------------\nHex     Mode  Sqwk  Flight   Alt    Spd  Hdg    Lat      Long   Sig  Msgs   Ti/\n-------------------------------------------------------------------------------\nHex     Mode  Sqwk  Flight   Alt    Spd  Hdg    Lat      Long   Sig  Msgs   Ti/\n-------------------------------------------------------------------------------\nHex     Mode  Sqwk  Flight   Alt    Spd  Hdg    Lat      Long   Sig  Msgs   Ti/\n-------------------------------------------------------------------------------\nHex     Mode  Sqwk  Flight   Alt    Spd  Hdg    Lat      Long   Sig  Msgs   Ti/\n-------------------------------------------------------------------------------\nHex     Mode  Sqwk  Flight   Alt    Spd  Hdg    Lat      Long   Sig  Msgs   Ti-\n-------------------------------------------------------------------------------\nHex     Mode  Sqwk  Flight   Alt    Spd  Hdg    Lat      Long   Sig  Msgs   Ti-\n-------------------------------------------------------------------------------\nHex     Mode  Sqwk  Flight   Alt    Spd  Hdg    Lat      Long   Sig  Msgs   Ti-\n-------------------------------------------------------------------------------\nHex     Mode  Sqwk  Flight   Alt    Spd  Hdg    Lat      Long   Sig  Msgs   Ti-\n-------------------------------------------------------------------------------\nHex     Mode  Sqwk  Flight   Alt    Spd  Hdg    Lat      Long   Sig  Msgs   Ti\\\n-------------------------------------------------------------------------------\nHex     Mode  Sqwk  Flight   Alt    Spd  Hdg    Lat      Long   Sig  Msgs   Ti\\\n-------------------------------------------------------------------------------\nHex     Mode  Sqwk  Flight   Alt    Spd  Hdg    Lat      Long   Sig  Msgs   Ti\\\n-------------------------------------------------------------------------------\nHex     Mode  Sqwk  Flight   Alt    Spd  Hdg    Lat      Long   Sig  Msgs   Ti\\\n-------------------------------------------------------------------------------\nHex     Mode  Sqwk  Flight   Alt    Spd  Hdg    Lat      Long   Sig  Msgs   Ti|\n-------------------------------------------------------------------------------\nHex     Mode  Sqwk  Flight   Alt    Spd  Hdg    Lat      Long   Sig  Msgs   Ti|\n-------------------------------------------------------------------------------\nHex     Mode  Sqwk  Flight   Alt    Spd  Hdg    Lat      Long   Sig  Msgs   Ti|\n-------------------------------------------------------------------------------\nHex     Mode  Sqwk  Flight   Alt    Spd  Hdg    Lat      Long   Sig  Msgs   Ti/\n-------------------------------------------------------------------------------\nHex     Mode  Sqwk  Flight   Alt    Spd  Hdg    Lat      Long   Sig  Msgs   Ti/\n-------------------------------------------------------------------------------\nHex     Mode  Sqwk  Flight   Alt    Spd  Hdg    Lat      Long   Sig  Msgs   Ti/\n-------------------------------------------------------------------------------\nHex     Mode  Sqwk  Flight   Alt    Spd  Hdg    Lat      Long   Sig  Msgs   Ti/\n-------------------------------------------------------------------------------\nHex     Mode  Sqwk  Flight   Alt    Spd  Hdg    Lat      Long   Sig  Msgs   Ti-\n-------------------------------------------------------------------------------\nHex     Mode  Sqwk  Flight   Alt    Spd  Hdg    Lat      Long   Sig  Msgs   Ti-\n-------------------------------------------------------------------------------\nHex     Mode  Sqwk  Flight   Alt    Spd  Hdg    Lat      Long   Sig  Msgs   Ti-\n-------------------------------------------------------------------------------\nHex     Mode  Sqwk  Flight   Alt    Spd  Hdg    Lat      Long   Sig  Msgs   Ti-\n-------------------------------------------------------------------------------\nHex     Mode  Sqwk  Flight   Alt    Spd  Hdg    Lat      Long   Sig  Msgs   Ti\\\n-------------------------------------------------------------------------------\nHex     Mode  Sqwk  Flight   Alt    Spd  Hdg    Lat      Long   Sig  Msgs   Ti\\\n-------------------------------------------------------------------------------\nHex     Mode  Sqwk  Flight   Alt    Spd  Hdg    Lat      Long   Sig  Msgs   Ti\\\n-------------------------------------------------------------------------------\nHex     Mode  Sqwk  Flight   Alt    Spd  Hdg    Lat      Long   Sig  Msgs   Ti\\\n-------------------------------------------------------------------------------\nHex     Mode  Sqwk  Flight   Alt    Spd  Hdg    Lat      Long   Sig  Msgs   Ti|\n-------------------------------------------------------------------------------\nHex     Mode  Sqwk  Flight   Alt    Spd  Hdg    Lat      Long   Sig  Msgs   Ti|\n-------------------------------------------------------------------------------\nHex     Mode  Sqwk  Flight   Alt    Spd  Hdg    Lat      Long   Sig  Msgs   Ti|\n-------------------------------------------------------------------------------\nHex     Mode  Sqwk  Flight   Alt    Spd  Hdg    Lat      Long   Sig  Msgs   Ti|\n-------------------------------------------------------------------------------\nHex     Mode  Sqwk  Flight   Alt    Spd  Hdg    Lat      Long   Sig  Msgs   Ti/\n-------------------------------------------------------------------------------\nHex     Mode  Sqwk  Flight   Alt    Spd  Hdg    Lat      Long   Sig  Msgs   Ti/\n-------------------------------------------------------------------------------\nHex     Mode  Sqwk  Flight   Alt    Spd  Hdg    Lat      Long   Sig  Msgs   Ti/\n-------------------------------------------------------------------------------\nHex     Mode  Sqwk  Flight   Alt    Spd  Hdg    Lat      Long   Sig  Msgs   Ti-\n-------------------------------------------------------------------------------\nHex     Mode  Sqwk  Flight   Alt    Spd  Hdg    Lat      Long   Sig  Msgs   Ti-\n-------------------------------------------------------------------------------\nHex     Mode  Sqwk  Flight   Alt    Spd  Hdg    Lat      Long   Sig  Msgs   Ti-\n-------------------------------------------------------------------------------\nHex     Mode  Sqwk  Flight   Alt    Spd  Hdg    Lat      Long   Sig  Msgs   Ti-\n-------------------------------------------------------------------------------\nHex     Mode  Sqwk  Flight   Alt    Spd  Hdg    Lat      Long   Sig  Msgs   Ti\\\n-------------------------------------------------------------------------------\nHex     Mode  Sqwk  Flight   Alt    Spd  Hdg    Lat      Long   Sig  Msgs   Ti\\\n-------------------------------------------------------------------------------\nHex     Mode  Sqwk  Flight   Alt    Spd  Hdg    Lat      Long   Sig  Msgs   Ti\\\n-------------------------------------------------------------------------------\nHex     Mode  Sqwk  Flight   Alt    Spd  Hdg    Lat      Long   Sig  Msgs   Ti\\\n-------------------------------------------------------------------------------\nHex     Mode  Sqwk  Flight   Alt    Spd  Hdg    Lat      Long   Sig  Msgs   Ti|\n-------------------------------------------------------------------------------\nHex     Mode  Sqwk  Flight   Alt    Spd  Hdg    Lat      Long   Sig  Msgs   Ti|\n-------------------------------------------------------------------------------\nHex     Mode  Sqwk  Flight   Alt    Spd  Hdg    Lat      Long   Sig  Msgs   Ti|\n-------------------------------------------------------------------------------\nHex     Mode  Sqwk  Flight   Alt    Spd  Hdg    Lat      Long   Sig  Msgs   Ti|\n-------------------------------------------------------------------------------\nHex     Mode  Sqwk  Flight   Alt    Spd  Hdg    Lat      Long   Sig  Msgs   Ti/\n-------------------------------------------------------------------------------\nHex     Mode  Sqwk  Flight   Alt    Spd  Hdg    Lat      Long   Sig  Msgs   Ti/\n-------------------------------------------------------------------------------\nHex     Mode  Sqwk  Flight   Alt    Spd  Hdg    Lat      Long   Sig  Msgs   Ti/\n-------------------------------------------------------------------------------\nHex     Mode  Sqwk  Flight   Alt    Spd  Hdg    Lat      Long   Sig  Msgs   Ti/\n-------------------------------------------------------------------------------\nHex     Mode  Sqwk  Flight   Alt    Spd  Hdg    Lat      Long   Sig  Msgs   Ti-\n-------------------------------------------------------------------------------\nHex     Mode  Sqwk  Flight   Alt    Spd  Hdg    Lat      Long   Sig  Msgs   Ti-\n-------------------------------------------------------------------------------\nHex     Mode  Sqwk  Flight   Alt    Spd  Hdg    Lat      Long   Sig  Msgs   Ti-\n-------------------------------------------------------------------------------\nHex     Mode  Sqwk  Flight   Alt    Spd  Hdg    Lat      Long   Sig  Msgs   Ti-\n-------------------------------------------------------------------------------\nHex     Mode  Sqwk  Flight   Alt    Spd  Hdg    Lat      Long   Sig  Msgs   Ti\\\n-------------------------------------------------------------------------------\nHex     Mode  Sqwk  Flight   Alt    Spd  Hdg    Lat      Long   Sig  Msgs   Ti\\\n-------------------------------------------------------------------------------\nHex     Mode  Sqwk  Flight   Alt    Spd  Hdg    Lat      Long   Sig  Msgs   Ti\\\n-------------------------------------------------------------------------------\nHex     Mode  Sqwk  Flight   Alt    Spd  Hdg    Lat      Long   Sig  Msgs   Ti|\n-------------------------------------------------------------------------------\nHex     Mode  Sqwk  Flight   Alt    Spd  Hdg    Lat      Long   Sig  Msgs   Ti|\n-------------------------------------------------------------------------------\nHex     Mode  Sqwk  Flight   Alt    Spd  Hdg    Lat      Long   Sig  Msgs   Ti|\n-------------------------------------------------------------------------------\nHex     Mode  Sqwk  Flight   Alt    Spd  Hdg    Lat      Long   Sig  Msgs   Ti|\n-------------------------------------------------------------------------------\nHex     Mode  Sqwk  Flight   Alt    Spd  Hdg    Lat      Long   Sig  Msgs   Ti/\n-------------------------------------------------------------------------------\nHex     Mode  Sqwk  Flight   Alt    Spd  Hdg    Lat      Long   Sig  Msgs   Ti/\n-------------------------------------------------------------------------------\nHex     Mode  Sqwk  Flight   Alt    Spd  Hdg    Lat      Long   Sig  Msgs   Ti/\n-------------------------------------------------------------------------------\nHex     Mode  Sqwk  Flight   Alt    Spd  Hdg    Lat      Long   Sig  Msgs   Ti/\n-------------------------------------------------------------------------------\nHex     Mode  Sqwk  Flight   Alt    Spd  Hdg    Lat      Long   Sig  Msgs   Ti-\n-------------------------------------------------------------------------------\nHex     Mode  Sqwk  Flight   Alt    Spd  Hdg    Lat      Long   Sig  Msgs   Ti-\n-------------------------------------------------------------------------------\nHex     Mode  Sqwk  Flight   Alt    Spd  Hdg    Lat      Long   Sig  Msgs   Ti-\n-------------------------------------------------------------------------------\nHex     Mode  Sqwk  Flight   Alt    Spd  Hdg    Lat      Long   Sig  Msgs   Ti-\n-------------------------------------------------------------------------------\nHex     Mode  Sqwk  Flight   Alt    Spd  Hdg    Lat      Long   Sig  Msgs   Ti\\\n-------------------------------------------------------------------------------\nHex     Mode  Sqwk  Flight   Alt    Spd  Hdg    Lat      Long   Sig  Msgs   Ti\\\n-------------------------------------------------------------------------------\nHex     Mode  Sqwk  Flight   Alt    Spd  Hdg    Lat      Long   Sig  Msgs   Ti\\\n-------------------------------------------------------------------------------\nHex     Mode  Sqwk  Flight   Alt    Spd  Hdg    Lat      Long   Sig  Msgs   Ti\\\n-------------------------------------------------------------------------------\nHex     Mode  Sqwk  Flight   Alt    Spd  Hdg    Lat      Long   Sig  Msgs   Ti|\n-------------------------------------------------------------------------------\nHex     Mode  Sqwk  Flight   Alt    Spd  Hdg    Lat      Long   Sig  Msgs   Ti|\n-------------------------------------------------------------------------------\nHex     Mode  Sqwk  Flight   Alt    Spd  Hdg    Lat      Long   Sig  Msgs   Ti|\n-------------------------------------------------------------------------------\nHex     Mode  Sqwk  Flight   Alt    Spd  Hdg    Lat      Long   Sig  Msgs   Ti/\n-------------------------------------------------------------------------------\nHex     Mode  Sqwk  Flight   Alt    Spd  Hdg    Lat      Long   Sig  Msgs   Ti/\n-------------------------------------------------------------------------------\nHex     Mode  Sqwk  Flight   Alt    Spd  Hdg    Lat      Long   Sig  Msgs   Ti/\n-------------------------------------------------------------------------------\nHex     Mode  Sqwk  Flight   Alt    Spd  Hdg    Lat      Long   Sig  Msgs   Ti/\n-------------------------------------------------------------------------------\nHex     Mode  Sqwk  Flight   Alt    Spd  Hdg    Lat      Long   Sig  Msgs   Ti-\n-------------------------------------------------------------------------------\nHex     Mode  Sqwk  Flight   Alt    Spd  Hdg    Lat      Long   Sig  Msgs   Ti-\n-------------------------------------------------------------------------------\nHex     Mode  Sqwk  Flight   Alt    Spd  Hdg    Lat      Long   Sig  Msgs   Ti-\n-------------------------------------------------------------------------------\nHex     Mode  Sqwk  Flight   Alt    Spd  Hdg    Lat      Long   Sig  Msgs   Ti-\n-------------------------------------------------------------------------------\nHex     Mode  Sqwk  Flight   Alt    Spd  Hdg    Lat      Long   Sig  Msgs   Ti\\\n-------------------------------------------------------------------------------\nHex     Mode  Sqwk  Flight   Alt    Spd  Hdg    Lat      Long   Sig  Msgs   Ti\\\n-------------------------------------------------------------------------------\nHex     Mode  Sqwk  Flight   Alt    Spd  Hdg    Lat      Long   Sig  Msgs   Ti\\\n-------------------------------------------------------------------------------\nHex     Mode  Sqwk  Flight   Alt    Spd  Hdg    Lat      Long   Sig  Msgs   Ti\\\n-------------------------------------------------------------------------------\nHex     Mode  Sqwk  Flight   Alt    Spd  Hdg    Lat      Long   Sig  Msgs   Ti|\n-------------------------------------------------------------------------------\nHex     Mode  Sqwk  Flight   Alt    Spd  Hdg    Lat      Long   Sig  Msgs   Ti|\n-------------------------------------------------------------------------------\nHex     Mode  Sqwk  Flight   Alt    Spd  Hdg    Lat      Long   Sig  Msgs   Ti|\n-------------------------------------------------------------------------------\nHex     Mode  Sqwk  Flight   Alt    Spd  Hdg    Lat      Long   Sig  Msgs   Ti|\n-------------------------------------------------------------------------------\nHex     Mode  Sqwk  Flight   Alt    Spd  Hdg    Lat      Long   Sig  Msgs   Ti/\n-------------------------------------------------------------------------------\nHex     Mode  Sqwk  Flight   Alt    Spd  Hdg    Lat      Long   Sig  Msgs   Ti/\n-------------------------------------------------------------------------------\nHex     Mode  Sqwk  Flight   Alt    Spd  Hdg    Lat      Long   Sig  Msgs   Ti/\n-------------------------------------------------------------------------------\nHex     Mode  Sqwk  Flight   Alt    Spd  Hdg    Lat      Long   Sig  Msgs   Ti-\n-------------------------------------------------------------------------------\nHex     Mode  Sqwk  Flight   Alt    Spd  Hdg    Lat      Long   Sig  Msgs   Ti-\n-------------------------------------------------------------------------------\nHex     Mode  Sqwk  Flight   Alt    Spd  Hdg    Lat      Long   Sig  Msgs   Ti-\n-------------------------------------------------------------------------------\nHex     Mode  Sqwk  Flight   Alt    Spd  Hdg    Lat      Long   Sig  Msgs   Ti-\n-------------------------------------------------------------------------------\nHex     Mode  Sqwk  Flight   Alt    Spd  Hdg    Lat      Long   Sig  Msgs   Ti\\\n-------------------------------------------------------------------------------\nHex     Mode  Sqwk  Flight   Alt    Spd  Hdg    Lat      Long   Sig  Msgs   Ti\\\n-------------------------------------------------------------------------------\nHex     Mode  Sqwk  Flight   Alt    Spd  Hdg    Lat      Long   Sig  Msgs   Ti\\\n-------------------------------------------------------------------------------\nHex     Mode  Sqwk  Flight   Alt    Spd  Hdg    Lat      Long   Sig  Msgs   Ti\\\n-------------------------------------------------------------------------------\nHex     Mode  Sqwk  Flight   Alt    Spd  Hdg    Lat      Long   Sig  Msgs   Ti|\n-------------------------------------------------------------------------------\nHex     Mode  Sqwk  Flight   Alt    Spd  Hdg    Lat      Long   Sig  Msgs   Ti|\n-------------------------------------------------------------------------------\nHex     Mode  Sqwk  Flight   Alt    Spd  Hdg    Lat      Long   Sig  Msgs   Ti|\n-------------------------------------------------------------------------------\nHex     Mode  Sqwk  Flight   Alt    Spd  Hdg    Lat      Long   Sig  Msgs   Ti|\n-------------------------------------------------------------------------------\nHex     Mode  Sqwk  Flight   Alt    Spd  Hdg    Lat      Long   Sig  Msgs   Ti/\n-------------------------------------------------------------------------------\nHex     Mode  Sqwk  Flight   Alt    Spd  Hdg    Lat      Long   Sig  Msgs   Ti/\n-------------------------------------------------------------------------------\nHex     Mode  Sqwk  Flight   Alt    Spd  Hdg    Lat      Long   Sig  Msgs   Ti/\n-------------------------------------------------------------------------------\nHex     Mode  Sqwk  Flight   Alt    Spd  Hdg    Lat      Long   Sig  Msgs   Ti/\n-------------------------------------------------------------------------------\nHex     Mode  Sqwk  Flight   Alt    Spd  Hdg    Lat      Long   Sig  Msgs   Ti-\n-------------------------------------------------------------------------------\nHex     Mode  Sqwk  Flight   Alt    Spd  Hdg    Lat      Long   Sig  Msgs   Ti-\n-------------------------------------------------------------------------------\nHex     Mode  Sqwk  Flight   Alt    Spd  Hdg    Lat      Long   Sig  Msgs   Ti-\n-------------------------------------------------------------------------------\nHex     Mode  Sqwk  Flight   Alt    Spd  Hdg    Lat      Long   Sig  Msgs   Ti-\n-------------------------------------------------------------------------------\nHex     Mode  Sqwk  Flight   Alt    Spd  Hdg    Lat      Long   Sig  Msgs   Ti\\\n-------------------------------------------------------------------------------\nHex     Mode  Sqwk  Flight   Alt    Spd  Hdg    Lat      Long   Sig  Msgs   Ti\\\n-------------------------------------------------------------------------------\nHex     Mode  Sqwk  Flight   Alt    Spd  Hdg    Lat      Long   Sig  Msgs   Ti\\\n-------------------------------------------------------------------------------\nHex     Mode  Sqwk  Flight   Alt    Spd  Hdg    Lat      Long   Sig  Msgs   Ti|\n-------------------------------------------------------------------------------\nHex     Mode  Sqwk  Flight   Alt    Spd  Hdg    Lat      Long   Sig  Msgs   Ti|\n-------------------------------------------------------------------------------\nHex     Mode  Sqwk  Flight   Alt    Spd  Hdg    Lat      Long   Sig  Msgs   Ti|\n-------------------------------------------------------------------------------\nHex     Mode  Sqwk  Flight   Alt    Spd  Hdg    Lat      Long   Sig  Msgs   Ti|\n-------------------------------------------------------------------------------\nHex     Mode  Sqwk  Flight   Alt    Spd  Hdg    Lat      Long   Sig  Msgs   Ti/\n-------------------------------------------------------------------------------\nHex     Mode  Sqwk  Flight   Alt    Spd  Hdg    Lat      Long   Sig  Msgs   Ti/\n-------------------------------------------------------------------------------\nHex     Mode  Sqwk  Flight   Alt    Spd  Hdg    Lat      Long   Sig  Msgs   Ti/\n-------------------------------------------------------------------------------\nHex     Mode  Sqwk  Flight   Alt    Spd  Hdg    Lat      Long   Sig  Msgs   Ti/\n-------------------------------------------------------------------------------\nHex     Mode  Sqwk  Flight   Alt    Spd  Hdg    Lat      Long   Sig  Msgs   Ti-\n-------------------------------------------------------------------------------\nHex     Mode  Sqwk  Flight   Alt    Spd  Hdg    Lat      Long   Sig  Msgs   Ti-\n-------------------------------------------------------------------------------\nHex     Mode  Sqwk  Flight   Alt    Spd  Hdg    Lat      Long   Sig  Msgs   Ti-\n-------------------------------------------------------------------------------\nHex     Mode  Sqwk  Flight   Alt    Spd  Hdg    Lat      Long   Sig  Msgs   Ti-\n-------------------------------------------------------------------------------\nHex     Mode  Sqwk  Flight   Alt    Spd  Hdg    Lat      Long   Sig  Msgs   Ti\\\n-------------------------------------------------------------------------------\nHex     Mode  Sqwk  Flight   Alt    Spd  Hdg    Lat      Long   Sig  Msgs   Ti\\\n-------------------------------------------------------------------------------\nHex     Mode  Sqwk  Flight   Alt    Spd  Hdg    Lat      Long   Sig  Msgs   Ti\\\n-------------------------------------------------------------------------------\nHex     Mode  Sqwk  Flight   Alt    Spd  Hdg    Lat      Long   Sig  Msgs   Ti\\\n-------------------------------------------------------------------------------\nHex     Mode  Sqwk  Flight   Alt    Spd  Hdg    Lat      Long   Sig  Msgs   Ti|\n-------------------------------------------------------------------------------\nHex     Mode  Sqwk  Flight   Alt    Spd  Hdg    Lat      Long   Sig  Msgs   Ti|\n-------------------------------------------------------------------------------\nHex     Mode  Sqwk  Flight   Alt    Spd  Hdg    Lat      Long   Sig  Msgs   Ti|\n-------------------------------------------------------------------------------\nHex     Mode  Sqwk  Flight   Alt    Spd  Hdg    Lat      Long   Sig  Msgs   Ti/\n-------------------------------------------------------------------------------\nHex     Mode  Sqwk  Flight   Alt    Spd  Hdg    Lat      Long   Sig  Msgs   Ti/\n-------------------------------------------------------------------------------\nHex     Mode  Sqwk  Flight   Alt    Spd  Hdg    Lat      Long   Sig  Msgs   Ti/\n-------------------------------------------------------------------------------\nHex     Mode  Sqwk  Flight   Alt    Spd  Hdg    Lat      Long   Sig  Msgs   Ti/\n-------------------------------------------------------------------------------\nHex     Mode  Sqwk  Flight   Alt    Spd  Hdg    Lat      Long   Sig  Msgs   Ti-\n-------------------------------------------------------------------------------\nHex     Mode  Sqwk  Flight   Alt    Spd  Hdg    Lat      Long   Sig  Msgs   Ti-\n-------------------------------------------------------------------------------\nHex     Mode  Sqwk  Flight   Alt    Spd  Hdg    Lat      Long   Sig  Msgs   Ti-\n-------------------------------------------------------------------------------\nHex     Mode  Sqwk  Flight   Alt    Spd  Hdg    Lat      Long   Sig  Msgs   Ti-\n-------------------------------------------------------------------------------\nHex     Mode  Sqwk  Flight   Alt    Spd  Hdg    Lat      Long   Sig  Msgs   Ti\\\n-------------------------------------------------------------------------------\nHex     Mode  Sqwk  Flight   Alt    Spd  Hdg    Lat      Long   Sig  Msgs   Ti\\\n-------------------------------------------------------------------------------\nHex     Mode  Sqwk  Flight   Alt    Spd  Hdg    Lat      Long   Sig  Msgs   Ti\\\n-------------------------------------------------------------------------------\nHex     Mode  Sqwk  Flight   Alt    Spd  Hdg    Lat      Long   Sig  Msgs   Ti\\\n-------------------------------------------------------------------------------\nHex     Mode  Sqwk  Flight   Alt    Spd  Hdg    Lat      Long   Sig  Msgs   Ti|\n-------------------------------------------------------------------------------\nHex     Mode  Sqwk  Flight   Alt    Spd  Hdg    Lat      Long   Sig  Msgs   Ti|\n-------------------------------------------------------------------------------\nHex     Mode  Sqwk  Flight   Alt    Spd  Hdg    Lat      Long   Sig  Msgs   Ti|\n-------------------------------------------------------------------------------\nHex     Mode  Sqwk  Flight   Alt    Spd  Hdg    Lat      Long   Sig  Msgs   Ti|\n-------------------------------------------------------------------------------\nHex     Mode  Sqwk  Flight   Alt    Spd  Hdg    Lat      Long   Sig  Msgs   Ti/\n-------------------------------------------------------------------------------\nHex     Mode  Sqwk  Flight   Alt    Spd  Hdg    Lat      Long   Sig  Msgs   Ti/\n-------------------------------------------------------------------------------\nHex     Mode  Sqwk  Flight   Alt    Spd  Hdg    Lat      Long   Sig  Msgs   Ti/\n-------------------------------------------------------------------------------\nHex     Mode  Sqwk  Flight   Alt    Spd  Hdg    Lat      Long   Sig  Msgs   Ti/\n-------------------------------------------------------------------------------\nHex     Mode  Sqwk  Flight   Alt    Spd  Hdg    Lat      Long   Sig  Msgs   Ti-\n-------------------------------------------------------------------------------\nHex     Mode  Sqwk  Flight   Alt    Spd  Hdg    Lat      Long   Sig  Msgs   Ti-\n-------------------------------------------------------------------------------\nHex     Mode  Sqwk  Flight   Alt    Spd  Hdg    Lat      Long   Sig  Msgs   Ti-\n-------------------------------------------------------------------------------\nHex     Mode  Sqwk  Flight   Alt    Spd  Hdg    Lat      Long   Sig  Msgs   Ti\\\n-------------------------------------------------------------------------------\nHex     Mode  Sqwk  Flight   Alt    Spd  Hdg    Lat      Long   Sig  Msgs   Ti\\\n-------------------------------------------------------------------------------\nHex     Mode  Sqwk  Flight   Alt    Spd  Hdg    Lat      Long   Sig  Msgs   Ti\\\n-------------------------------------------------------------------------------\nHex     Mode  Sqwk  Flight   Alt    Spd  Hdg    Lat      Long   Sig  Msgs   Ti\\\n-------------------------------------------------------------------------------\nHex     Mode  Sqwk  Flight   Alt    Spd  Hdg    Lat      Long   Sig  Msgs   Ti|\n-------------------------------------------------------------------------------\nHex     Mode  Sqwk  Flight   Alt    Spd  Hdg    Lat      Long   Sig  Msgs   Ti|\n-------------------------------------------------------------------------------\nHex     Mode  Sqwk  Flight   Alt    Spd  Hdg    Lat      Long   Sig  Msgs   Ti|\n-------------------------------------------------------------------------------\nHex     Mode  Sqwk  Flight   Alt    Spd  Hdg    Lat      Long   Sig  Msgs   Ti|\n-------------------------------------------------------------------------------\nHex     Mode  Sqwk  Flight   Alt    Spd  Hdg    Lat      Long   Sig  Msgs   Ti/\n-------------------------------------------------------------------------------\nHex     Mode  Sqwk  Flight   Alt    Spd  Hdg    Lat      Long   Sig  Msgs   Ti/\n-------------------------------------------------------------------------------\nHex     Mode  Sqwk  Flight   Alt    Spd  Hdg    Lat      Long   Sig  Msgs   Ti/\n-------------------------------------------------------------------------------\nHex     Mode  Sqwk  Flight   Alt    Spd  Hdg    Lat      Long   Sig  Msgs   Ti/\n-------------------------------------------------------------------------------\nHex     Mode  Sqwk  Flight   Alt    Spd  Hdg    Lat      Long   Sig  Msgs   Ti-\n-------------------------------------------------------------------------------\nHex     Mode  Sqwk  Flight   Alt    Spd  Hdg    Lat      Long   Sig  Msgs   Ti-\n-------------------------------------------------------------------------------\nHex     Mode  Sqwk  Flight   Alt    Spd  Hdg    Lat      Long   Sig  Msgs   Ti-\n-------------------------------------------------------------------------------\nHex     Mode  Sqwk  Flight   Alt    Spd  Hdg    Lat      Long   Sig  Msgs   Ti-\n-------------------------------------------------------------------------------\nHex     Mode  Sqwk  Flight   Alt    Spd  Hdg    Lat      Long   Sig  Msgs   Ti\\\n-------------------------------------------------------------------------------\nHex     Mode  Sqwk  Flight   Alt    Spd  Hdg    Lat      Long   Sig  Msgs   Ti\\\n-------------------------------------------------------------------------------\nHex     Mode  Sqwk  Flight   Alt    Spd  Hdg    Lat      Long   Sig  Msgs   Ti\\\n-------------------------------------------------------------------------------\nHex     Mode  Sqwk  Flight   Alt    Spd  Hdg    Lat      Long   Sig  Msgs   Ti|\n-------------------------------------------------------------------------------\nHex     Mode  Sqwk  Flight   Alt    Spd  Hdg    Lat      Long   Sig  Msgs   Ti|\n-------------------------------------------------------------------------------\nHex     Mode  Sqwk  Flight   Alt    Spd  Hdg    Lat      Long   Sig  Msgs   Ti|\n-------------------------------------------------------------------------------\nHex     Mode  Sqwk  Flight   Alt    Spd  Hdg    Lat      Long   Sig  Msgs   Ti|\n-------------------------------------------------------------------------------\nHex     Mode  Sqwk  Flight   Alt    Spd  Hdg    Lat      Long   Sig  Msgs   Ti/\n-------------------------------------------------------------------------------\nHex     Mode  Sqwk  Flight   Alt    Spd  Hdg    Lat      Long   Sig  Msgs   Ti/\n-------------------------------------------------------------------------------\nHex     Mode  Sqwk  Flight   Alt    Spd  Hdg    Lat      Long   Sig  Msgs   Ti/\n-------------------------------------------------------------------------------\nHex     Mode  Sqwk  Flight   Alt    Spd  Hdg    Lat      Long   Sig  Msgs   Ti/\n-------------------------------------------------------------------------------\nHex     Mode  Sqwk  Flight   Alt    Spd  Hdg    Lat      Long   Sig  Msgs   Ti-\n-------------------------------------------------------------------------------\nHex     Mode  Sqwk  Flight   Alt    Spd  Hdg    Lat      Long   Sig  Msgs   Ti-\n-------------------------------------------------------------------------------\nHex     Mode  Sqwk  Flight   Alt    Spd  Hdg    Lat      Long   Sig  Msgs   Ti-\n-------------------------------------------------------------------------------\nHex     Mode  Sqwk  Flight   Alt    Spd  Hdg    Lat      Long   Sig  Msgs   Ti-\n-------------------------------------------------------------------------------\nHex     Mode  Sqwk  Flight   Alt    Spd  Hdg    Lat      Long   Sig  Msgs   Ti\\\n-------------------------------------------------------------------------------\nHex     Mode  Sqwk  Flight   Alt    Spd  Hdg    Lat      Long   Sig  Msgs   Ti\\\n-------------------------------------------------------------------------------\nHex     Mode  Sqwk  Flight   Alt    Spd  Hdg    Lat      Long   Sig  Msgs   Ti\\\n-------------------------------------------------------------------------------\nHex     Mode  Sqwk  Flight   Alt    Spd  Hdg    Lat      Long   Sig  Msgs   Ti\\\n-------------------------------------------------------------------------------\nHex     Mode  Sqwk  Flight   Alt    Spd  Hdg    Lat      Long   Sig  Msgs   Ti|\n-------------------------------------------------------------------------------\nHex     Mode  Sqwk  Flight   Alt    Spd  Hdg    Lat      Long   Sig  Msgs   Ti|\n-------------------------------------------------------------------------------\nHex     Mode  Sqwk  Flight   Alt    Spd  Hdg    Lat      Long   Sig  Msgs   Ti|\n-------------------------------------------------------------------------------\nHex     Mode  Sqwk  Flight   Alt    Spd  Hdg    Lat      Long   Sig  Msgs   Ti/\n-------------------------------------------------------------------------------\nHex     Mode  Sqwk  Flight   Alt    Spd  Hdg    Lat      Long   Sig  Msgs   Ti/\n-------------------------------------------------------------------------------\nHex     Mode  Sqwk  Flight   Alt    Spd  Hdg    Lat      Long   Sig  Msgs   Ti/\n-------------------------------------------------------------------------------\nHex     Mode  Sqwk  Flight   Alt    Spd  Hdg    Lat      Long   Sig  Msgs   Ti/\n-------------------------------------------------------------------------------\nHex     Mode  Sqwk  Flight   Alt    Spd  Hdg    Lat      Long   Sig  Msgs   Ti-\n-------------------------------------------------------------------------------\nHex     Mode  Sqwk  Flight   Alt    Spd  Hdg    Lat      Long   Sig  Msgs   Ti-\n-------------------------------------------------------------------------------\nHex     Mode  Sqwk  Flight   Alt    Spd  Hdg    Lat      Long   Sig  Msgs   Ti-\n-------------------------------------------------------------------------------\nHex     Mode  Sqwk  Flight   Alt    Spd  Hdg    Lat      Long   Sig  Msgs   Ti-\n-------------------------------------------------------------------------------\nHex     Mode  Sqwk  Flight   Alt    Spd  Hdg    Lat      Long   Sig  Msgs   Ti\\\n-------------------------------------------------------------------------------\nHex     Mode  Sqwk  Flight   Alt    Spd  Hdg    Lat      Long   Sig  Msgs   Ti\\\n-------------------------------------------------------------------------------\nHex     Mode  Sqwk  Flight   Alt    Spd  Hdg    Lat      Long   Sig  Msgs   Ti\\\n-------------------------------------------------------------------------------\nHex     Mode  Sqwk  Flight   Alt    Spd  Hdg    Lat      Long   Sig  Msgs   Ti\\\n-------------------------------------------------------------------------------\nHex     Mode  Sqwk  Flight   Alt    Spd  Hdg    Lat      Long   Sig  Msgs   Ti|\n-------------------------------------------------------------------------------\nHex     Mode  Sqwk  Flight   Alt    Spd  Hdg    Lat      Long   Sig  Msgs   Ti|\n-------------------------------------------------------------------------------\nHex     Mode  Sqwk  Flight   Alt    Spd  Hdg    Lat      Long   Sig  Msgs   Ti|\n-------------------------------------------------------------------------------\nHex     Mode  Sqwk  Flight   Alt    Spd  Hdg    Lat      Long   Sig  Msgs   Ti|\n-------------------------------------------------------------------------------\nHex     Mode  Sqwk  Flight   Alt    Spd  Hdg    Lat      Long   Sig  Msgs   Ti/\n-------------------------------------------------------------------------------\nHex     Mode  Sqwk  Flight   Alt    Spd  Hdg    Lat      Long   Sig  Msgs   Ti/\n-------------------------------------------------------------------------------\nHex     Mode  Sqwk  Flight   Alt    Spd  Hdg    Lat      Long   Sig  Msgs   Ti/\n-------------------------------------------------------------------------------\nHex     Mode  Sqwk  Flight   Alt    Spd  Hdg    Lat      Long   Sig  Msgs   Ti/\n-------------------------------------------------------------------------------\nHex     Mode  Sqwk  Flight   Alt    Spd  Hdg    Lat      Long   Sig  Msgs   Ti-\n-------------------------------------------------------------------------------\nHex     Mode  Sqwk  Flight   Alt    Spd  Hdg    Lat      Long   Sig  Msgs   Ti-\n-------------------------------------------------------------------------------\nHex     Mode  Sqwk  Flight   Alt    Spd  Hdg    Lat      Long   Sig  Msgs   Ti-\n-------------------------------------------------------------------------------\nHex     Mode  Sqwk  Flight   Alt    Spd  Hdg    Lat      Long   Sig  Msgs   Ti\\\n-------------------------------------------------------------------------------\nHex     Mode  Sqwk  Flight   Alt    Spd  Hdg    Lat      Long   Sig  Msgs   Ti\\\n-------------------------------------------------------------------------------\nHex     Mode  Sqwk  Flight   Alt    Spd  Hdg    Lat      Long   Sig  Msgs   Ti\\\n-------------------------------------------------------------------------------\nHex     Mode  Sqwk  Flight   Alt    Spd  Hdg    Lat      Long   Sig  Msgs   Ti\\\n-------------------------------------------------------------------------------\nHex     Mode  Sqwk  Flight   Alt    Spd  Hdg    Lat      Long   Sig  Msgs   Ti|\n-------------------------------------------------------------------------------\nHex     Mode  Sqwk  Flight   Alt    Spd  Hdg    Lat      Long   Sig  Msgs   Ti|\n-------------------------------------------------------------------------------\nHex     Mode  Sqwk  Flight   Alt    Spd  Hdg    Lat      Long   Sig  Msgs   Ti|\n-------------------------------------------------------------------------------\nHex     Mode  Sqwk  Flight   Alt    Spd  Hdg    Lat      Long   Sig  Msgs   Ti|\n-------------------------------------------------------------------------------\nHex     Mode  Sqwk  Flight   Alt    Spd  Hdg    Lat      Long   Sig  Msgs   Ti/\n-------------------------------------------------------------------------------\nHex     Mode  Sqwk  Flight   Alt    Spd  Hdg    Lat      Long   Sig  Msgs   Ti/\n-------------------------------------------------------------------------------\nHex     Mode  Sqwk  Flight   Alt    Spd  Hdg    Lat      Long   Sig  Msgs   Ti/\n-------------------------------------------------------------------------------\nHex     Mode  Sqwk  Flight   Alt    Spd  Hdg    Lat      Long   Sig  Msgs   Ti/\n-------------------------------------------------------------------------------\nHex     Mode  Sqwk  Flight   Alt    Spd  Hdg    Lat      Long   Sig  Msgs   Ti-\n-------------------------------------------------------------------------------\nHex     Mode  Sqwk  Flight   Alt    Spd  Hdg    Lat      Long   Sig  Msgs   Ti-\n-------------------------------------------------------------------------------\nHex     Mode  Sqwk  Flight   Alt    Spd  Hdg    Lat      Long   Sig  Msgs   Ti-\n-------------------------------------------------------------------------------\nHex     Mode  Sqwk  Flight   Alt    Spd  Hdg    Lat      Long   Sig  Msgs   Ti-\n-------------------------------------------------------------------------------\nHex     Mode  Sqwk  Flight   Alt    Spd  Hdg    Lat      Long   Sig  Msgs   Ti\\\n-------------------------------------------------------------------------------\nHex     Mode  Sqwk  Flight   Alt    Spd  Hdg    Lat      Long   Sig  Msgs   Ti\\\n-------------------------------------------------------------------------------\nHex     Mode  Sqwk  Flight   Alt    Spd  Hdg    Lat      Long   Sig  Msgs   Ti\\\n-------------------------------------------------------------------------------\nHex     Mode  Sqwk  Flight   Alt    Spd  Hdg    Lat      Long   Sig  Msgs   Ti|\n-------------------------------------------------------------------------------\nHex     Mode  Sqwk  Flight   Alt    Spd  Hdg    Lat      Long   Sig  Msgs   Ti|\n-------------------------------------------------------------------------------\nHex     Mode  Sqwk  Flight   Alt    Spd  Hdg    Lat      Long   Sig  Msgs   Ti|\n-------------------------------------------------------------------------------\nHex     Mode  Sqwk  Flight   Alt    Spd  Hdg    Lat      Long   Sig  Msgs   Ti|\n-------------------------------------------------------------------------------\nHex     Mode  Sqwk  Flight   Alt    Spd  Hdg    Lat     \nC:\\Data\\dump1090-win.1.10.3010.14>dump1090.exe --interactive --net --net-beast --net-http-port 8081\n-----------------------------------------------------------------------------\n|                        dump1090 ModeS Receiver         Ver : 1.10.3010.14 |\n-----------------------------------------------------------------------------\n\n Copyright (C) 2012 by Salvatore Sanfilippo <antirez@gmail.com>\n Copyright (C) 2014 by Malcolm Robb <support@attavionics.com>\n\n All rights reserved.\n\n THIS SOFTWARE IS PROVIDED BY THE COPYRIGHT HOLDERS AND CONTRIBUTORS\n AS IS AND ANY EXPRESS OR IMPLIED WARRANTIES, INCLUDING, BUT NOT\n LIMITED TO, THE IMPLIED WARRANTIES OF MERCHANTABILITY AND FITNESS FOR\n A PARTICULAR PURPOSE ARE DISCLAIMED. IN NO EVENT SHALL THE COPYRIGHT\n HOLDER OR CONTRIBUTORS BE LIABLE FOR ANY DIRECT, INDIRECT, INCIDENTAL,\n SPECIAL, EXEMPLARY, OR CONSEQUENTIAL DAMAGES (INCLUDING, BUT NOT\n LIMITED TO, PROCUREMENT OF SUBSTITUTE GOODS OR SERVICES; LOSS OF USE,\n DATA, OR PROFITS; OR BUSINESS INTERRUPTION) HOWEVER CAUSED AND ON ANY\n THEORY OF LIABILITY, WHETHER IN CONTRACT, STRICT LIABILITY, OR TORT\n (INCLUDING NEGLIGENCE OR OTHERWISE) ARISING IN ANY WAY OUT OF THE USE\n OF THIS SOFTWARE, EVEN IF ADVISED OF THE POSSIBILITY OF SUCH DAMAGE.\n\n For further details refer to <https://github.com/MalcolmRobb/dump1090>\n\nHex     Mode  Sqwk  Flight   Alt    Spd  Hdg    Lat      Long   Sig  Msgs   Ti|\n-------------------------------------------------------------------------------\nHex     Mode  Sqwk  Flight   Alt    Spd  Hdg    Lat      Long   Sig  Msgs   Ti/\n-------------------------------------------------------------------------------\nHex     Mode  Sqwk  Flight   Alt    Spd  Hdg    Lat      Long   Sig  Msgs   Ti/\n-------------------------------------------------------------------------------\nHex     Mode  Sqwk  Flight   Alt    Spd  Hdg    Lat      Long   Sig  Msgs   Ti/\n-------------------------------------------------------------------------------\nHex     Mode  Sqwk  Flight   Alt    Spd  Hdg    Lat      Long   Sig  Msgs   Ti/\n-------------------------------------------------------------------------------\nHex     Mode  Sqwk  Flight   Alt    Spd  Hdg    Lat      Long   Sig  Msgs   Ti-\n-------------------------------------------------------------------------------\nHex     Mode  Sqwk  Flight   Alt    Spd  Hdg    Lat      Long   Sig  Msgs   Ti-\n-------------------------------------------------------------------------------\nHex     Mode  Sqwk  Flight   Alt    Spd  Hdg    Lat      Long   Sig  Msgs   Ti-\n-------------------------------------------------------------------------------\nHex     Mode  Sqwk  Flight   Alt    Spd  Hdg    Lat      Long   Sig  Msgs   Ti-\n-------------------------------------------------------------------------------\nHex     Mode  Sqwk  Flight   Alt    Spd  Hdg    Lat      Long   Sig  Msgs   Ti\\\n-------------------------------------------------------------------------------\nA1DF3E  S                           303  264                     10     1    1\nHex     Mode  Sqwk  Flight   Alt    Spd  Hdg    Lat      Long   Sig  Msgs   Ti\\\n-------------------------------------------------------------------------------\nA1DF3E  S                           303  264                     10     1    1\nHex     Mode  Sqwk  Flight   Alt    Spd  Hdg    Lat      Long   Sig  Msgs   Ti\\\n-------------------------------------------------------------------------------\nA1DF3E  S                           303  264                     10     1    1\nHex     Mode  Sqwk  Flight   Alt    Spd  Hdg    Lat      Long   Sig  Msgs   Ti\\\n-------------------------------------------------------------------------------\nA1DF3E  S                           303  264                     10     1    1\nHex     Mode  Sqwk  Flight   Alt    Spd  Hdg    Lat      Long   Sig  Msgs   Ti|\n-------------------------------------------------------------------------------\nA1DF3E  S                           303  265                     10     2    1\nHex     Mode  Sqwk  Flight   Alt    Spd  Hdg    Lat      Long   Sig  Msgs   Ti|\n-------------------------------------------------------------------------------\nA1DF3E  S                           303  265                     11     3    0\nHex     Mode  Sqwk  Flight   Alt    Spd  Hdg    Lat      Long   Sig  Msgs   Ti|\n-------------------------------------------------------------------------------\nA1DF3E  S                           303  265                     11     3    0\nHex     Mode  Sqwk  Flight   Alt    Spd  Hdg    Lat      Long   Sig  Msgs   Ti|\n-------------------------------------------------------------------------------\nA1DF3E  S                     9875  303  265                     11     4    0\nHex     Mode  Sqwk  Flight   Alt    Spd  Hdg    Lat      Long   Sig  Msgs   Ti/\n-------------------------------------------------------------------------------\nA1DF3E  S                     9875  303  265                     11     4    1\nHex     Mode  Sqwk  Flight   Alt    Spd  Hdg    Lat      Long   Sig  Msgs   Ti/\n-------------------------------------------------------------------------------\nA1DF3E  S                     9875  303  265                     10     5    0\nHex     Mode  Sqwk  Flight   Alt    Spd  Hdg    Lat      Long   Sig  Msgs   Ti/\n-------------------------------------------------------------------------------\nA1DF3E  S                     9875  303  265                     11     6    0\nHex     Mode  Sqwk  Flight   Alt    Spd  Hdg    Lat      Long   Sig  Msgs   Ti/\n-------------------------------------------------------------------------------\nA1DF3E  S                     9875  303  266                     11     7    0\nHex     Mode  Sqwk  Flight   Alt    Spd  Hdg    Lat      Long   Sig  Msgs   Ti-\n-------------------------------------------------------------------------------\nA1DF3E  S                     9875  303  266                     11     9    0\nHex     Mode  Sqwk  Flight   Alt    Spd  Hdg    Lat      Long   Sig  Msgs   Ti-\n-------------------------------------------------------------------------------\nA1DF3E  S                     9875  303  266                     11     9    0\nHex     Mode  Sqwk  Flight   Alt    Spd  Hdg    Lat      Long   Sig  Msgs   Ti-\n-------------------------------------------------------------------------------\nA1DF3E  S                     9875  302  266                     11    10    0\nHex     Mode  Sqwk  Flight   Alt    Spd  Hdg    Lat      Long   Sig  Msgs   Ti\\\n-------------------------------------------------------------------------------\nA1DF3E  S                     9875  302  266                     11    10    1\nHex     Mode  Sqwk  Flight   Alt    Spd  Hdg    Lat      Long   Sig  Msgs   Ti\\\n-------------------------------------------------------------------------------\nA1DF3E  S                     9875  302  266                     11    10    1\nHex     Mode  Sqwk  Flight   Alt    Spd  Hdg    Lat      Long   Sig  Msgs   Ti\\\n-------------------------------------------------------------------------------\nA1DF3E  S                     9875  302  266                     11    10    1\nHex     Mode  Sqwk  Flight   Alt    Spd  Hdg    Lat      Long   Sig  Msgs   Ti\\\n-------------------------------------------------------------------------------\nA1DF3E  S                     9875  302  266                     11    10    1\nHex     Mode  Sqwk  Flight   Alt    Spd  Hdg    Lat      Long   Sig  Msgs   Ti|\n-------------------------------------------------------------------------------\nA1DF3E  S                     9875  302  266                     11    10    2\nHex     Mode  Sqwk  Flight   Alt    Spd  Hdg    Lat      Long   Sig  Msgs   Ti|\n-------------------------------------------------------------------------------\nA1DF3E  S                     9875  302  266                     10    11    0\nHex     Mode  Sqwk  Flight   Alt    Spd  Hdg    Lat      Long   Sig  Msgs   Ti|\n-------------------------------------------------------------------------------\nA1DF3E  S                     9875  302  266                     10    11    0\nHex     Mode  Sqwk  Flight   Alt    Spd  Hdg    Lat      Long   Sig  Msgs   Ti|\n-------------------------------------------------------------------------------\nA1DF3E  S                     9875  302  266                     10    11    0\nHex     Mode  Sqwk  Flight   Alt    Spd  Hdg    Lat      Long   Sig  Msgs   Ti/\n-------------------------------------------------------------------------------\nA1DF3E  S                     9875  302  266                     10    11    1\nHex     Mode  Sqwk  Flight   Alt    Spd  Hdg    Lat      Long   Sig  Msgs   Ti/\n-------------------------------------------------------------------------------\nA1DF3E  S                     9875  302  266                     10    11    1\nHex     Mode  Sqwk  Flight   Alt    Spd  Hdg    Lat      Long   Sig  Msgs   Ti/\n-------------------------------------------------------------------------------\nA1DF3E  S                     9875  302  266                     10    12    0\nHex     Mode  Sqwk  Flight   Alt    Spd  Hdg    Lat      Long   Sig  Msgs   Ti/\n-------------------------------------------------------------------------------\nA1DF3E  S                     9875  302  266                     10    12    0\nHex     Mode  Sqwk  Flight   Alt    Spd  Hdg    Lat      Long   Sig  Msgs   Ti-\n-------------------------------------------------------------------------------\nA1DF3E  S                     9875  302  268                     10    14    0\nHex     Mode  Sqwk  Flight   Alt    Spd  Hdg    Lat      Long   Sig  Msgs   Ti-\n-------------------------------------------------------------------------------\nA1DF3E  S                     9875  302  268                     10    15    0\nHex     Mode  Sqwk  Flight   Alt    Spd  Hdg    Lat      Long   Sig  Msgs   Ti-\n-------------------------------------------------------------------------------\nA1DF3E  S                     9875  302  268                     10    16    0\nHex     Mode  Sqwk  Flight   Alt    Spd  Hdg    Lat      Long   Sig  Msgs   Ti-\n-------------------------------------------------------------------------------\nA1DF3E  S                     9875  302  268   40.127  -79.492   11    17    0\nHex     Mode  Sqwk  Flight   Alt    Spd  Hdg    Lat      Long   Sig  Msgs   Ti\\\n-------------------------------------------------------------------------------\nA1DF3E  S                     9875  302  268   40.127  -79.492   11    18    0\nHex     Mode  Sqwk  Flight   Alt    Spd  Hdg    Lat      Long   Sig  Msgs   Ti\\\n-------------------------------------------------------------------------------\nA1DF3E  S                     9875  302  268   40.126  -79.493   11    19    0\nHex     Mode  Sqwk  Flight   Alt    Spd  Hdg    Lat      Long   Sig  Msgs   Ti\\\n-------------------------------------------------------------------------------\nA1DF3E  S                     9875  302  268   40.126  -79.493   11    20    0\nHex     Mode  Sqwk  Flight   Alt    Spd  Hdg    Lat      Long   Sig  Msgs   Ti|\n-------------------------------------------------------------------------------\nA1DF3E  S                     9875  302  268   40.126  -79.493   11    20    1\nHex     Mode  Sqwk  Flight   Alt    Spd  Hdg    Lat      Long   Sig  Msgs   Ti|\n-------------------------------------------------------------------------------\nA1DF3E  S                     9875  302  268   40.126  -79.493   11    21    0\nHex     Mode  Sqwk  Flight   Alt    Spd  Hdg    Lat      Long   Sig  Msgs   Ti|\n-------------------------------------------------------------------------------\nA1DF3E  S                     9875  302  269   40.126  -79.493   12    24    0\nHex     Mode  Sqwk  Flight   Alt    Spd  Hdg    Lat      Long   Sig  Msgs   Ti|\n-------------------------------------------------------------------------------\nA1DF3E  S                     9875  302  269   40.126  -79.493   12    24    0\nHex     Mode  Sqwk  Flight   Alt    Spd  Hdg    Lat      Long   Sig  Msgs   Ti/\n-------------------------------------------------------------------------------\nA1DF3E  S                     9875  302  269   40.126  -79.493   11    25    1\nHex     Mode  Sqwk  Flight   Alt    Spd  Hdg    Lat      Long   Sig  Msgs   Ti/\n-------------------------------------------------------------------------------\nA1DF3E  S                     9875  302  269   40.126  -79.493   11    25    1\nHex     Mode  Sqwk  Flight   Alt    Spd  Hdg    Lat      Long   Sig  Msgs   Ti/\n-------------------------------------------------------------------------------\nA1DF3E  S                     9875  302  269   40.126  -79.493   12    26    0\nHex     Mode  Sqwk  Flight   Alt    Spd  Hdg    Lat      Long   Sig  Msgs   Ti/\n-------------------------------------------------------------------------------\nA1DF3E  S                     9875  302  269   40.126  -79.498   12    27    0\nHex     Mode  Sqwk  Flight   Alt    Spd  Hdg    Lat      Long   Sig  Msgs   Ti-\n-------------------------------------------------------------------------------\nA1DF3E  S                     9875  302  269   40.126  -79.498   11    28    1\nHex     Mode  Sqwk  Flight   Alt    Spd  Hdg    Lat      Long   Sig  Msgs   Ti-\n-------------------------------------------------------------------------------\nA1DF3E  S                     9875  302  269   40.126  -79.498   11    28    1\nHex     Mode  Sqwk  Flight   Alt    Spd  Hdg    Lat      Long   Sig  Msgs   Ti-\n-------------------------------------------------------------------------------\nA1DF3E  S                     9875  302  269   40.126  -79.498   11    29    0\nHex     Mode  Sqwk  Flight   Alt    Spd  Hdg    Lat      Long   Sig  Msgs   Ti-\n-------------------------------------------------------------------------------\nA1DF3E  S                     9875  302  269   40.126  -79.500   11    30    0\nHex     Mode  Sqwk  Flight   Alt    Spd  Hdg    Lat      Long   Sig  Msgs   Ti\\\n-------------------------------------------------------------------------------\nA1DF3E  S                     9875  302  269   40.126  -79.500   11    30    1\nHex     Mode  Sqwk  Flight   Alt    Spd  Hdg    Lat      Long   Sig  Msgs   Ti\\\n-------------------------------------------------------------------------------\nA1DF3E  S                     9875  302  269   40.126  -79.500   11    30    1\nHex     Mode  Sqwk  Flight   Alt    Spd  Hdg    Lat      Long   Sig  Msgs   Ti\\\n-------------------------------------------------------------------------------\nA1DF3E  S                     9875  302  269   40.126  -79.500   11    30    1\nHex     Mode  Sqwk  Flight   Alt    Spd  Hdg    Lat      Long   Sig  Msgs   Ti\\\n-------------------------------------------------------------------------------\nA1DF3E  S                     9875  302  269   40.126  -79.500   11    30    1\nHex     Mode  Sqwk  Flight   Alt    Spd  Hdg    Lat      Long   Sig  Msgs   Ti|\n-------------------------------------------------------------------------------\nA1DF3E  S                     9875  302  269   40.126  -79.500   11    30    2\nHex     Mode  Sqwk  Flight   Alt    Spd  Hdg    Lat      Long   Sig  Msgs   Ti|\n-------------------------------------------------------------------------------\nA1DF3E  S                     9875  302  269   40.126  -79.500   11    30    2\nHex     Mode  Sqwk  Flight   Alt    Spd  Hdg    Lat      Long   Sig  Msgs   Ti|\n-------------------------------------------------------------------------------\nA1DF3E  S                     9875  302  269   40.126  -79.503   11    31    0\nHex     Mode  Sqwk  Flight   Alt    Spd  Hdg    Lat      Long   Sig  Msgs   Ti/\n-------------------------------------------------------------------------------\nA1DF3E  S                     9875  302  269   40.126  -79.503   11    31    1\nHex     Mode  Sqwk  Flight   Alt    Spd  Hdg    Lat      Long   Sig  Msgs   Ti/\n-------------------------------------------------------------------------------\nA1DF3E  S                     9875  302  269   40.126  -79.503   11    31    1\nHex     Mode  Sqwk  Flight   Alt    Spd  Hdg    Lat      Long   Sig  Msgs   Ti/\n-------------------------------------------------------------------------------\nA1DF3E  S                     9875  302  269   40.126  -79.503   11    31    1\nHex     Mode  Sqwk  Flight   Alt    Spd  Hdg    Lat      Long   Sig  Msgs   Ti/\n-------------------------------------------------------------------------------\nA1DF3E  S                     9875  302  269   40.126  -79.503   11    32    0\nHex     Mode  Sqwk  Flight   Alt    Spd  Hdg    Lat      Long   Sig  Msgs   Ti-\n-------------------------------------------------------------------------------\nA1DF3E  S                     9875  302  269   40.126  -79.503   11    32    1\nHex     Mode  Sqwk  Flight   Alt    Spd  Hdg    Lat      Long   Sig  Msgs   Ti-\n-------------------------------------------------------------------------------\nA1DF3E  S                     9875  301  271   40.126  -79.503   11    33    0\nHex     Mode  Sqwk  Flight   Alt    Spd  Hdg    Lat      Long   Sig  Msgs   Ti-\n-------------------------------------------------------------------------------\nA1DF3E  S                     9875  301  271   40.126  -79.506   11    34    0\nHex     Mode  Sqwk  Flight   Alt    Spd  Hdg    Lat      Long   Sig  Msgs   Ti-\n-------------------------------------------------------------------------------\nA1DF3E  S                     9875  301  271   40.126  -79.506   11    34    0\nHex     Mode  Sqwk  Flight   Alt    Spd  Hdg    Lat      Long   Sig  Msgs   Ti\\\n-------------------------------------------------------------------------------\nA1DF3E  S                     9875  301  271   40.126  -79.506   11    34    1\nHex     Mode  Sqwk  Flight   Alt    Spd  Hdg    Lat      Long   Sig  Msgs   Ti\\\n-------------------------------------------------------------------------------\nA1DF3E  S                     9875  301  271   40.126  -79.506   11    34    1\nHex     Mode  Sqwk  Flight   Alt    Spd  Hdg    Lat      Long   Sig  Msgs   Ti\\\n-------------------------------------------------------------------------------\nA1DF3E  S                     9875  301  271   40.126  -79.506   11    34    1\nHex     Mode  Sqwk  Flight   Alt    Spd  Hdg    Lat      Long   Sig  Msgs   Ti\\\n-------------------------------------------------------------------------------\nA1DF3E  S                     9875  301  271   40.126  -79.506   11    34    1\nHex     Mode  Sqwk  Flight   Alt    Spd  Hdg    Lat      Long   Sig  Msgs   Ti|\n-------------------------------------------------------------------------------\nA1DF3E  S                     9875  301  271   40.126  -79.506   11    35    0\nHex     Mode  Sqwk  Flight   Alt    Spd  Hdg    Lat      Long   Sig  Msgs   Ti|\n-------------------------------------------------------------------------------\nA1DF3E  S                     9875  301  271   40.126  -79.506   11    35    0\nHex     Mode  Sqwk  Flight   Alt    Spd  Hdg    Lat      Long   Sig  Msgs   Ti|\n-------------------------------------------------------------------------------\nA1DF3E  S                     9875  301  271   40.126  -79.510   11    36    0\nHex     Mode  Sqwk  Flight   Alt    Spd  Hdg    Lat      Long   Sig  Msgs   Ti|\n-------------------------------------------------------------------------------\nA1DF3E  S                     9875  301  271   40.126  -79.510   11    36    0\nHex     Mode  Sqwk  Flight   Alt    Spd  Hdg    Lat      Long   Sig  Msgs   Ti/\n-------------------------------------------------------------------------------\nA1DF3E  S                     9875  301  271   40.126  -79.510   11    36    1\nHex     Mode  Sqwk  Flight   Alt    Spd  Hdg    Lat      Long   Sig  Msgs   Ti/\n-------------------------------------------------------------------------------\nA1DF3E  S                     9875  301  271   40.126  -79.510   11    36    1\nHex     Mode  Sqwk  Flight   Alt    Spd  Hdg    Lat      Long   Sig  Msgs   Ti/\n-------------------------------------------------------------------------------\nA1DF3E  S                     9875  301  271   40.126  -79.510   11    36    1\nHex     Mode  Sqwk  Flight   Alt    Spd  Hdg    Lat      Long   Sig  Msgs   Ti/\n-------------------------------------------------------------------------------\nA1DF3E  S                     9875  301  271   40.126  -79.510   11    36    1\nHex     Mode  Sqwk  Flight   Alt    Spd  Hdg    Lat      Long   Sig  Msgs   Ti-\n-------------------------------------------------------------------------------\nA1DF3E  S                     9875  301  271   40.126  -79.510   11    36    2\nHex     Mode  Sqwk  Flight   Alt    Spd  Hdg    Lat      Long   Sig  Msgs   Ti-\n-------------------------------------------------------------------------------\nA1DF3E  S                     9875  301  271   40.126  -79.510   11    36    2\nHex     Mode  Sqwk  Flight   Alt    Spd  Hdg    Lat      Long   Sig  Msgs   Ti-\n-------------------------------------------------------------------------------\nA1DF3E  S                     9875  301  271   40.126  -79.510   11    36    2\nHex     Mode  Sqwk  Flight   Alt    Spd  Hdg    Lat      Long   Sig  Msgs   Ti\\\n-------------------------------------------------------------------------------\nA1DF3E  S                     9875  301  271   40.126  -79.510   11    36    3\nHex     Mode  Sqwk  Flight   Alt    Spd  Hdg    Lat      Long   Sig  Msgs   Ti\\\n-------------------------------------------------------------------------------\nA1DF3E  S                     9875  301  271   40.126  -79.510   11    36    3\nHex     Mode  Sqwk  Flight   Alt    Spd  Hdg    Lat      Long   Sig  Msgs   Ti\\\n-------------------------------------------------------------------------------\nA1DF3E  S                     9875  301  271   40.126  -79.510   11    36    3\nHex     Mode  Sqwk  Flight   Alt    Spd  Hdg    Lat      Long   Sig  Msgs   Ti\\\n-------------------------------------------------------------------------------\nA1DF3E  S                     9875  301  271   40.126  -79.510   11    36    3\nHex     Mode  Sqwk  Flight   Alt    Spd  Hdg    Lat      Long   Sig  Msgs   Ti|\n-------------------------------------------------------------------------------\nA1DF3E  S                     9875  301  271   40.126  -79.510   11    36    4\nHex     Mode  Sqwk  Flight   Alt    Spd  Hdg    Lat      Long   Sig  Msgs   Ti|\n-------------------------------------------------------------------------------\nA1DF3E  S                     9875  301  271   40.126  -79.510   11    36    4\nHex     Mode  Sqwk  Flight   Alt    Spd  Hdg    Lat      Long   Sig  Msgs   Ti|\n-------------------------------------------------------------------------------\nA1DF3E  S                     9875  301  271   40.126  -79.510   11    36    4\nHex     Mode  Sqwk  Flight   Alt    Spd  Hdg    Lat      Long   Sig  Msgs   Ti|\n-------------------------------------------------------------------------------\nA1DF3E  S                     9875  301  271   40.126  -79.510   11    37    0\nHex     Mode  Sqwk  Flight   Alt    Spd  Hdg    Lat      Long   Sig  Msgs   Ti/\n-------------------------------------------------------------------------------\nA1DF3E  S                     9875  301  271   40.126  -79.510   11    37    1\nHex     Mode  Sqwk  Flight   Alt    Spd  Hdg    Lat      Long   Sig  Msgs   Ti/\n-------------------------------------------------------------------------------\nA1DF3E  S                     9875  301  273   40.126  -79.510   12    38    0\nHex     Mode  Sqwk  Flight   Alt    Spd  Hdg    Lat      Long   Sig  Msgs   Ti/\n-------------------------------------------------------------------------------\nA1DF3E  S                     9875  301  273   40.127  -79.519   11    39    0\nHex     Mode  Sqwk  Flight   Alt    Spd  Hdg    Lat      Long   Sig  Msgs   Ti/\n-------------------------------------------------------------------------------\nA1DF3E  S                     9875  301  273   40.127  -79.519   11    39    0\nHex     Mode  Sqwk  Flight   Alt    Spd  Hdg    Lat      Long   Sig  Msgs   Ti-\n-------------------------------------------------------------------------------\nA1DF3E  S                     9875  301  273   40.127  -79.519   11    39    1\nHex     Mode  Sqwk  Flight   Alt    Spd  Hdg    Lat      Long   Sig  Msgs   Ti-\n-------------------------------------------------------------------------------\nA1DF3E  S                     9875  301  273   40.127  -79.519   11    39    1\nHex     Mode  Sqwk  Flight   Alt    Spd  Hdg    Lat      Long   Sig  Msgs   Ti-\n-------------------------------------------------------------------------------\nA1DF3E  S                     9875  301  273   40.127  -79.519   11    39    1\nHex     Mode  Sqwk  Flight   Alt    Spd  Hdg    Lat      Long   Sig  Msgs   Ti-\n-------------------------------------------------------------------------------\nA1DF3E  S                     9875  300  274   40.127  -79.519   11    41    0\nHex     Mode  Sqwk  Flight   Alt    Spd  Hdg    Lat      Long   Sig  Msgs   Ti\\\n-------------------------------------------------------------------------------\nA1DF3E  S                     9875  300  274   40.127  -79.519   11    41    1\nHex     Mode  Sqwk  Flight   Alt    Spd  Hdg    Lat      Long   Sig  Msgs   Ti\\\n-------------------------------------------------------------------------------\nA1DF3E  S                     9875  300  274   40.127  -79.519   11    41    1\nHex     Mode  Sqwk  Flight   Alt    Spd  Hdg    Lat      Long   Sig  Msgs   Ti\\\n-------------------------------------------------------------------------------\nA1DF3E  S                     9875  300  274   40.127  -79.523   12    43    0\nHex     Mode  Sqwk  Flight   Alt    Spd  Hdg    Lat      Long   Sig  Msgs   Ti|\n-------------------------------------------------------------------------------\nA1DF3E  S                     9875  300  274   40.127  -79.523   12    43    1\nHex     Mode  Sqwk  Flight   Alt    Spd  Hdg    Lat      Long   Sig  Msgs   Ti|\n-------------------------------------------------------------------------------\nA1DF3E  S                     9875  300  274   40.127  -79.523   12    43    1\nHex     Mode  Sqwk  Flight   Alt    Spd  Hdg    Lat      Long   Sig  Msgs   Ti|\n-------------------------------------------------------------------------------\nA1DF3E  S                     9875  300  274   40.127  -79.523   12    43    1\nHex     Mode  Sqwk  Flight   Alt    Spd  Hdg    Lat      Long   Sig  Msgs   Ti|\n-------------------------------------------------------------------------------\nA1DF3E  S                     9875  300  274   40.127  -79.525   13    45    0\nHex     Mode  Sqwk  Flight   Alt    Spd  Hdg    Lat      Long   Sig  Msgs   Ti/\n-------------------------------------------------------------------------------\nA1DF3E  S                     9875  300  274   40.127  -79.525   13    45    1\nHex     Mode  Sqwk  Flight   Alt    Spd  Hdg    Lat      Long   Sig  Msgs   Ti/\n-------------------------------------------------------------------------------\nA1DF3E  S                     9875  300  274   40.127  -79.525   13    45    1\nHex     Mode  Sqwk  Flight   Alt    Spd  Hdg    Lat      Long   Sig  Msgs   Ti/\n-------------------------------------------------------------------------------\nA1DF3E  S                     9875  300  274   40.127  -79.525   12    46    0\nHex     Mode  Sqwk  Flight   Alt    Spd  Hdg    Lat      Long   Sig  Msgs   Ti/\n-------------------------------------------------------------------------------\nA1DF3E  S                     9875  300  274   40.127  -79.527   12    47    0\nHex     Mode  Sqwk  Flight   Alt    Spd  Hdg    Lat      Long   Sig  Msgs   Ti-\n-------------------------------------------------------------------------------\nA1DF3E  S                     9875  300  274   40.127  -79.527   12    47    1\nHex     Mode  Sqwk  Flight   Alt    Spd  Hdg    Lat      Long   Sig  Msgs   Ti-\n-------------------------------------------------------------------------------\nA1DF3E  S                     9875  300  274   40.127  -79.527   12    47    1\nHex     Mode  Sqwk  Flight   Alt    Spd  Hdg    Lat      Long   Sig  Msgs   Ti-\n-------------------------------------------------------------------------------\nA1DF3E  S                     9875  300  274   40.127  -79.527   13    48    0\nHex     Mode  Sqwk  Flight   Alt    Spd  Hdg    Lat      Long   Sig  Msgs   Ti-\n-------------------------------------------------------------------------------\nA1DF3E  S                     9875  300  274   40.127  -79.527   12    49    0\nHex     Mode  Sqwk  Flight   Alt    Spd  Hdg    Lat      Long   Sig  Msgs   Ti\\\n-------------------------------------------------------------------------------\nA1DF3E  S                     9875  300  274   40.127  -79.527   12    49    1\nHex     Mode  Sqwk  Flight   Alt    Spd  Hdg    Lat      Long   Sig  Msgs   Ti\\\n-------------------------------------------------------------------------------\nA1DF3E  S                     9875  300  274   40.127  -79.527   12    49    1\nHex     Mode  Sqwk  Flight   Alt    Spd  Hdg    Lat      Long   Sig  Msgs   Ti\\\n-------------------------------------------------------------------------------\nA1DF3E  S                     9875  300  274   40.127  -79.527   12    49    1\nHex     Mode  Sqwk  Flight   Alt    Spd  Hdg    Lat      Long   Sig  Msgs   Ti\\\n-------------------------------------------------------------------------------\nA1DF3E  S                     9875  300  274   40.127  -79.527   12    49    1\nHex     Mode  Sqwk  Flight   Alt    Spd  Hdg    Lat      Long   Sig  Msgs   Ti|\n-------------------------------------------------------------------------------\nA1DF3E  S                     9875  300  274   40.127  -79.527   12    49    2\nHex     Mode  Sqwk  Flight   Alt    Spd  Hdg    Lat      Long   Sig  Msgs   Ti|\n-------------------------------------------------------------------------------\nA1DF3E  S                     9875  300  274   40.127  -79.527   12    49    2\nHex     Mode  Sqwk  Flight   Alt    Spd  Hdg    Lat      Long   Sig  Msgs   Ti|\n-------------------------------------------------------------------------------\nA1DF3E  S                     9875  300  274   40.127  -79.527   11    50    0\nHex     Mode  Sqwk  Flight   Alt    Spd  Hdg    Lat      Long   Sig  Msgs   Ti/\n-------------------------------------------------------------------------------\nA1DF3E  S                     9875  300  274   40.127  -79.527   11    50    1\nHex     Mode  Sqwk  Flight   Alt    Spd  Hdg    Lat      Long   Sig  Msgs   Ti/\n-------------------------------------------------------------------------------\nA1DF3E  S                     9875  300  274   40.127  -79.527   11    50    1\nHex     Mode  Sqwk  Flight   Alt    Spd  Hdg    Lat      Long   Sig  Msgs   Ti/\n-------------------------------------------------------------------------------\nA1DF3E  S                     9875  300  274   40.127  -79.527   11    50    1\nHex     Mode  Sqwk  Flight   Alt    Spd  Hdg    Lat      Long   Sig  Msgs   Ti/\n-------------------------------------------------------------------------------\nA1DF3E  S                     9875  300  274   40.127  -79.527   11    50    1\nHex     Mode  Sqwk  Flight   Alt    Spd  Hdg    Lat      Long   Sig  Msgs   Ti-\n-------------------------------------------------------------------------------\nA1DF3E  S                     9875  300  274   40.127  -79.527   11    50    2\nHex     Mode  Sqwk  Flight   Alt    Spd  Hdg    Lat      Long   Sig  Msgs   Ti-\n-------------------------------------------------------------------------------\nA1DF3E  S                     9875  300  274   40.127  -79.527   11    50    2\nHex     Mode  Sqwk  Flight   Alt    Spd  Hdg    Lat      Long   Sig  Msgs   Ti-\n-------------------------------------------------------------------------------\nA1DF3E  S                     9875  300  274   40.127  -79.527   11    50    2\nHex     Mode  Sqwk  Flight   Alt    Spd  Hdg    Lat      Long   Sig  Msgs   Ti-\n-------------------------------------------------------------------------------\nA1DF3E  S                     9875  300  274   40.127  -79.527   11    50    2\nHex     Mode  Sqwk  Flight   Alt    Spd  Hdg    Lat      Long   Sig  Msgs   Ti\\\n-------------------------------------------------------------------------------\nA1DF3E  S                     9875  300  274   40.127  -79.527   11    50    3\nHex     Mode  Sqwk  Flight   Alt    Spd  Hdg    Lat      Long   Sig  Msgs   Ti\\\n-------------------------------------------------------------------------------\nA1DF3E  S                     9875  300  274   40.127  -79.527   11    50    3\nHex     Mode  Sqwk  Flight   Alt    Spd  Hdg    Lat      Long   Sig  Msgs   Ti\\\n-------------------------------------------------------------------------------\nA1DF3E  S                     9875  300  274   40.127  -79.527   11    50    3\nHex     Mode  Sqwk  Flight   Alt    Spd  Hdg    Lat      Long   Sig  Msgs   Ti\\\n-------------------------------------------------------------------------------\nA1DF3E  S                     9875  300  274   40.127  -79.527   11    50    3\nHex     Mode  Sqwk  Flight   Alt    Spd  Hdg    Lat      Long   Sig  Msgs   Ti|\n-------------------------------------------------------------------------------\nA1DF3E  S                     9875  300  274   40.127  -79.527   11    50    4\nHex     Mode  Sqwk  Flight   Alt    Spd  Hdg    Lat      Long   Sig  Msgs   Ti|\n-------------------------------------------------------------------------------\nA1DF3E  S                     9875  300  274   40.127  -79.527   11    50    4\nHex     Mode  Sqwk  Flight   Alt    Spd  Hdg    Lat      Long   Sig  Msgs   Ti|\n-------------------------------------------------------------------------------\nA1DF3E  S                     9875  300  274   40.127  -79.527   11    50    4\nHex     Mode  Sqwk  Flight   Alt    Spd  Hdg    Lat      Long   Sig  Msgs   Ti|\n-------------------------------------------------------------------------------\nA1DF3E  S                     9875  300  274   40.127  -79.527   11    50    4\nHex     Mode  Sqwk  Flight   Alt    Spd  Hdg    Lat      Long   Sig  Msgs   Ti/\n-------------------------------------------------------------------------------\nA1DF3E  S                     9875  300  274   40.127  -79.527   11    50    5\nHex     Mode  Sqwk  Flight   Alt    Spd  Hdg    Lat      Long   Sig  Msgs   Ti/\n-------------------------------------------------------------------------------\nA1DF3E  S                     9875  300  274   40.127  -79.527   11    50    5\nHex     Mode  Sqwk  Flight   Alt    Spd  Hdg    Lat      Long   Sig  Msgs   Ti/\n-------------------------------------------------------------------------------\nA1DF3E  S                     9875  300  274   40.127  -79.527   11    50    5\nHex     Mode  Sqwk  Flight   Alt    Spd  Hdg    Lat      Long   Sig  Msgs   Ti/\n-------------------------------------------------------------------------------\nA1DF3E  S                     9875  300  274   40.127  -79.527   11    50    5\nHex     Mode  Sqwk  Flight   Alt    Spd  Hdg    Lat      Long   Sig  Msgs   Ti-\n-------------------------------------------------------------------------------\nA1DF3E  S           N22G      9875  300  274   40.127  -79.527   11    51    0\nHex     Mode  Sqwk  Flight   Alt    Spd  Hdg    Lat      Long   Sig  Msgs   Ti-\n-------------------------------------------------------------------------------\nA1DF3E  S           N22G      9875  300  274   40.127  -79.527   11    51    0\nHex     Mode  Sqwk  Flight   Alt    Spd  Hdg    Lat      Long   Sig  Msgs   Ti-\n-------------------------------------------------------------------------------\nA1DF3E  S           N22G      9875  300  274   40.128  -79.543   11    52    0\nHex     Mode  Sqwk  Flight   Alt    Spd  Hdg    Lat      Long   Sig  Msgs   Ti\\\n-------------------------------------------------------------------------------\nA1DF3E  S           N22G      9875  299  274   40.128  -79.543   11    53    1\nHex     Mode  Sqwk  Flight   Alt    Spd  Hdg    Lat      Long   Sig  Msgs   Ti\\\n-------------------------------------------------------------------------------\nA1DF3E  S           N22G      9875  299  274   40.128  -79.543   11    53    1\nHex     Mode  Sqwk  Flight   Alt    Spd  Hdg    Lat      Long   Sig  Msgs   Ti\\\n-------------------------------------------------------------------------------\nA1DF3E  S           N22G      9875  299  274   40.128  -79.543   11    54    0\nHex     Mode  Sqwk  Flight   Alt    Spd  Hdg    Lat      Long   Sig  Msgs   Ti\\\n-------------------------------------------------------------------------------\nA1DF3E  S           N22G      9875  299  274   40.128  -79.543   11    54    0\nHex     Mode  Sqwk  Flight   Alt    Spd  Hdg    Lat      Long   Sig  Msgs   Ti|\n-------------------------------------------------------------------------------\nA1DF3E  S           N22G      9875  299  274   40.128  -79.543   11    54    1\nHex     Mode  Sqwk  Flight   Alt    Spd  Hdg    Lat      Long   Sig  Msgs   Ti|\n-------------------------------------------------------------------------------\nA1DF3E  S           N22G      9875  299  274   40.128  -79.543   11    55    0\nHex     Mode  Sqwk  Flight   Alt    Spd  Hdg    Lat      Long   Sig  Msgs   Ti|\n-------------------------------------------------------------------------------\nA1DF3E  S           N22G      9875  299  274   40.128  -79.546   11    56    0\nHex     Mode  Sqwk  Flight   Alt    Spd  Hdg    Lat      Long   Sig  Msgs   Ti|\n-------------------------------------------------------------------------------\nA1DF3E  S           N22G      9875  299  274   40.128  -79.546   11    57    0\nHex     Mode  Sqwk  Flight   Alt    Spd  Hdg    Lat      Long   Sig  Msgs   Ti/\n-------------------------------------------------------------------------------\nA1DF3E  S           N22G      9875  299  274   40.128  -79.546   11    57    1\nHex     Mode  Sqwk  Flight   Alt    Spd  Hdg    Lat      Long   Sig  Msgs   Ti/\n-------------------------------------------------------------------------------\nA1DF3E  S           N22G      9875  299  274   40.128  -79.546   11    57    1\nHex     Mode  Sqwk  Flight   Alt    Spd  Hdg    Lat      Long   Sig  Msgs   Ti/\n-------------------------------------------------------------------------------\nA1DF3E  S           N22G      9875  299  274   40.128  -79.548   11    59    0\nHex     Mode  Sqwk  Flight   Alt    Spd  Hdg    Lat      Long   Sig  Msgs   Ti/\n-------------------------------------------------------------------------------\nA1DF3E  S           N22G      9875  299  274   40.128  -79.548   11    59    0\nHex     Mode  Sqwk  Flight   Alt    Spd  Hdg    Lat      Long   Sig  Msgs   Ti-\n-------------------------------------------------------------------------------\nA1DF3E  S           N22G      9875  299  274   40.128  -79.548   11    59    1\nHex     Mode  Sqwk  Flight   Alt    Spd  Hdg    Lat      Long   Sig  Msgs   Ti-\n-------------------------------------------------------------------------------\nA1DF3E  S           N22G      9875  299  274   40.128  -79.550   12    60    0\nHex     Mode  Sqwk  Flight   Alt    Spd  Hdg    Lat      Long   Sig  Msgs   Ti-\n-------------------------------------------------------------------------------\nA1DF3E  S           N22G      9875  299  274   40.128  -79.550   12    60    0\nHex     Mode  Sqwk  Flight   Alt    Spd  Hdg    Lat      Long   Sig  Msgs   Ti-\n-------------------------------------------------------------------------------\nA1DF3E  S           N22G      9875  299  274   40.128  -79.550   12    60    0\nHex     Mode  Sqwk  Flight   Alt    Spd  Hdg    Lat      Long   Sig  Msgs   Ti\\\n-------------------------------------------------------------------------------\nA1DF3E  S           N22G      9875  299  274   40.128  -79.550   12    60    1\nHex     Mode  Sqwk  Flight   Alt    Spd  Hdg    Lat      Long   Sig  Msgs   Ti\\\n-------------------------------------------------------------------------------\nA1DF3E  S           N22G      9875  299  275   40.128  -79.550   11    62    0\nHex     Mode  Sqwk  Flight   Alt    Spd  Hdg    Lat      Long   Sig  Msgs   Ti\\\n-------------------------------------------------------------------------------\nA1DF3E  S           N22G      9875  299  275   40.128  -79.550   11    62    0\nHex     Mode  Sqwk  Flight   Alt    Spd  Hdg    Lat      Long   Sig  Msgs   Ti|\n-------------------------------------------------------------------------------\nA1DF3E  S           N22G      9875  299  275   40.128  -79.550   13    64    1\nHex     Mode  Sqwk  Flight   Alt    Spd  Hdg    Lat      Long   Sig  Msgs   Ti|\n-------------------------------------------------------------------------------\nA1DF3E  S           N22G      9875  299  275   40.128  -79.553   12    66    0\nHex     Mode  Sqwk  Flight   Alt    Spd  Hdg    Lat      Long   Sig  Msgs   Ti|\n-------------------------------------------------------------------------------\nA1DF3E  S           N22G      9875  299  274   40.128  -79.553   12    67    0\nHex     Mode  Sqwk  Flight   Alt    Spd  Hdg    Lat      Long   Sig  Msgs   Ti|\n-------------------------------------------------------------------------------\nA1DF3E  S           N22G      9875  299  274   40.128  -79.553   12    67    0\nHex     Mode  Sqwk  Flight   Alt    Spd  Hdg    Lat      Long   Sig  Msgs   Ti/\n-------------------------------------------------------------------------------\nA1DF3E  S           N22G      9875  299  274   40.128  -79.553   14    69    0\nHex     Mode  Sqwk  Flight   Alt    Spd  Hdg    Lat      Long   Sig  Msgs   Ti/\n-------------------------------------------------------------------------------\nA1DF3E  S           N22G      9875  299  274   40.128  -79.553   14    69    0\nHex     Mode  Sqwk  Flight   Alt    Spd  Hdg    Lat      Long   Sig  Msgs   Ti/\n-------------------------------------------------------------------------------\nA1DF3E  S           N22G      9875  299  274   40.128  -79.553   14    69    0\nHex     Mode  Sqwk  Flight   Alt    Spd  Hdg    Lat      Long   Sig  Msgs   Ti/\n-------------------------------------------------------------------------------\nA1DF3E  S           N22G      9875  299  274   40.128  -79.555   15    71    0\nHex     Mode  Sqwk  Flight   Alt    Spd  Hdg    Lat      Long   Sig  Msgs   Ti-\n-------------------------------------------------------------------------------\nA1DF3E  S           N22G      9875  298  275   40.128  -79.555   15    72    1\nHex     Mode  Sqwk  Flight   Alt    Spd  Hdg    Lat      Long   Sig  Msgs   Ti-\n-------------------------------------------------------------------------------\nA1DF3E  S           N22G      9875  298  275   40.128  -79.555   15    72    1\nHex     Mode  Sqwk  Flight   Alt    Spd  Hdg    Lat      Long   Sig  Msgs   Ti-\n-------------------------------------------------------------------------------\nA1DF3E  S           N22G      9875  298  275   40.128  -79.555   15    73    0\nHex     Mode  Sqwk  Flight   Alt    Spd  Hdg    Lat      Long   Sig  Msgs   Ti-\n-------------------------------------------------------------------------------\nA1DF3E  S           N22G      9875  298  275   40.128  -79.555   15    73    0\nHex     Mode  Sqwk  Flight   Alt    Spd  Hdg    Lat      Long   Sig  Msgs   Ti\\\n-------------------------------------------------------------------------------\nA1DF3E  S           N22G      9875  298  275   40.128  -79.555   19    76    0\nHex     Mode  Sqwk  Flight   Alt    Spd  Hdg    Lat      Long   Sig  Msgs   Ti\\\n-------------------------------------------------------------------------------\nA1DF3E  S           N22G      9875  298  275   40.128  -79.555   18    77    0\nHex     Mode  Sqwk  Flight   Alt    Spd  Hdg    Lat      Long   Sig  Msgs   Ti\\\n-------------------------------------------------------------------------------\nA1DF3E  S           N22G      9875  298  275   40.129  -79.559   17    79    0\nHex     Mode  Sqwk  Flight   Alt    Spd  Hdg    Lat      Long   Sig  Msgs   Ti\\\n-------------------------------------------------------------------------------\nA1DF3E  S           N22G      9875  298  275   40.129  -79.559   17    79    0\nHex     Mode  Sqwk  Flight   Alt    Spd  Hdg    Lat      Long   Sig  Msgs   Ti|\n-------------------------------------------------------------------------------\nA1DF3E  S           N22G      9875  298  275   40.129  -79.560   17    81    0\nHex     Mode  Sqwk  Flight   Alt    Spd  Hdg    Lat      Long   Sig  Msgs   Ti|\n-------------------------------------------------------------------------------\nA1DF3E  S           N22G      9875  298  275   40.129  -79.560   15    82    0\nHex     Mode  Sqwk  Flight   Alt    Spd  Hdg    Lat      Long   Sig  Msgs   Ti|\n-------------------------------------------------------------------------------\nA1DF3E  S           N22G      9875  298  275   40.129  -79.561   15    83    0\nHex     Mode  Sqwk  Flight   Alt    Spd  Hdg    Lat      Long   Sig  Msgs   Ti|\n-------------------------------------------------------------------------------\nA1DF3E  S           N22G      9875  298  275   40.129  -79.562   15    85    0\nHex     Mode  Sqwk  Flight   Alt    Spd  Hdg    Lat      Long   Sig  Msgs   Ti/\n-------------------------------------------------------------------------------\nA1DF3E  S           N22G      9875  298  275   40.129  -79.562   14    86    0\nHex     Mode  Sqwk  Flight   Alt    Spd  Hdg    Lat      Long   Sig  Msgs   Ti/\n---------"
  # "dump1090.exe --interactive --net --net-beast --net-http-port 8081"
  # "Greensburg:\nMy location coordinates are:\nLatitude: 40.286792 / N 40° 17' 12.452''\nLongitude: -79.541260 / W 79° 32' 28.537''"
  # "https://icons.iconarchive.com/icons/papirus-team/papirus-status/64/airplane-mode-icon.png"
  # "https://image.flaticon.com/icons/png/512/633/633800.png"
  # "t.ly/zRy1"
  # "file:///C:/Users/Kaitie/Desktop/cesium/testbillboard.html"
  # "for blue pin"
  n1 = disable-structure shown="Disabled" {
    frame Disabled {
      n2 = call <vilib>:"example_cmd.vi"() -> ()  [unwired: 12 in]
    }
    frame Enabled {
    }
  }
  n3 = disable-structure shown="Enabled" {
    disable-tunnel: [w32 _] -> w13
    frame Enabled {
      n4 = call "TCP.vi"() -> ("data out"=w35:string)  [unwired: 11 in]
      n5 = Spreadsheet String To Array(delimiter (Tab)=",", format string="%s", spreadsheet string=w35, array type (2D Dbl)=w35) -> (array=w32:string[][])
    }
    frame Disabled {
    }
  }
  "Raw data" <- w13
  n6 = for {
    tunnel: w13 -> [w58] mode=indexing
    shift-right: [w55] -> w7
    shift-left: T1[] [] -> [w56]
    n7 = Index Array(array=w58, index #1=4 ("index"), index #2=1 ("index"), index #3=12 ("index"), index #4=13 ("index"), index #5=11 ("index"), index #6=14 ("index"), index #7=15 ("index"), index #8=21 ("index")) -> (element #1=w40:string, element #2=w41:string, element #3=w49:string, element #4=w48:string, element #5=w46:string, element #6=w43:string, element #7=w42:string, element #8=w38:string)
    n8 = Equal?(x=w38, y="") -> (x = y?=w36:bool)
    n9 = for {
      tunnel: w56 -> [w138] mode=indexing
      tunnel: w40 -> [w139]
      tunnel: [w137] -> w54
      tunnel: [w136] -> w53
      tunnel: [w135] -> _
      i -> [w136]
      stop <- w137 stop-if-true
      n10 = Unbundle By Name(w138) -> ("ICAO"=w135:string)
      n11 = Equal?(x=w135, y=w139) -> (x = y?=w137:bool)
    }
    n12 = case shown="True" w36 {
      tunnel: w56 -> [w69 w134]
      tunnel: [w68 w134] -> w55
      tunnel: w54 -> [w67 _]
      tunnel: w53 -> [w66 _]
      tunnel: w49 -> [w65 _]
      tunnel: w48 -> [w64 _]
      tunnel: w46 -> [w63 _]
      tunnel: w43 -> [w62 _]
      tunnel: w42 -> [w61 _]
      tunnel: w41 -> [w60 _]
      tunnel: w40 -> [w59 _]
      frame False {
        n13 = case shown="True" w67 {
          tunnel: w69 -> [w78 w109]
          tunnel: [w77 w110] -> w68
          tunnel: w66 -> [_ w108]
          tunnel: w60 -> [_ w107]
          tunnel: w59 -> [w76 w104]
          tunnel: w65 -> [w75 w103]
          tunnel: w64 -> [w71 w102]
          tunnel: w63 -> [w73 w101]
          tunnel: w62 -> [w74 w100]
          tunnel: w61 -> [w72 w99]
          tunnel: w60 -> [w70 _]
          frame False {
            n14 = case shown="\"3\", \"4\", \"5\", \"7\"" w70 {
              tunnel: w78 -> [w79 w98]
              tunnel: [w79 w97] -> w77
              tunnel: w76 -> [_ w94]
              tunnel: w75 -> [_ w93]
              tunnel: w74 -> [_ w89]
              tunnel: w73 -> [_ w80]
              tunnel: w72 -> [_ w85]
              tunnel: w71 -> [_ w82]
              frame "False", Default {
              }
              frame "3", "4", "5", "7" {
                n15 = Decimal String To Number(string=w93, default (0L)=0.0 ("default (0 I32)")) -> (number=w92:dbl)  [unwired: 1 in, 1 out]
                n16 = Fract/Exp String To Number(string=w89, default (0 dbl)=0.0 ("default (0 I32)")) -> (number=w86:dbl)  [unwired: 2 in, 1 out]
                n17 = Decimal String To Number(string=w80, default (0L)=0.0 ("default (0 I32)")) -> ()  [unwired: 1 in, 2 out]
                n18 = Fract/Exp String To Number(string=w85, default (0 dbl)=0.0 ("default (0 I32)")) -> (number=w84:dbl)  [unwired: 2 in, 1 out]
                n19 = Decimal String To Number(string=w82, default (0L)=0.0 ("default (0 I32)")) -> (number=w81:dbl)  [unwired: 1 in, 1 out]
                n20 = Bundle By Name(cluster=T1 {"ICAO"="", "Latitude"=0.0, "Longitude"=0.0, "Heading"=0.0, "Speed"=0.0, "Alt"=""} ("new element/subarray"), "ICAO"=w94, "Latitude"=w86, "Longitude"=w84, "Heading"=w81, "Alt"=w80, "Speed"=w92) -> (w95:T1)
                n21 = Insert Into Array(array=w98, new element=w95) -> (w97:T1[])  [unwired: 1 in]
              }
            }
          }
          frame True {
            n22 = Index Array(array=w109, index=w108) -> (element=w106:T1)
            n23 = case shown="\"3\"" w107 {
              tunnel: w106 -> [w118 w119 w124 w133]
              tunnel: [w117 w119 w123 w132] -> w105
              tunnel: w104 -> [w116 _ w122 w131]
              tunnel: w103 -> [w115 _ _ _]
              tunnel: w102 -> [w114 _ _ _]
              tunnel: w101 -> [_ _ w120 w125]
              tunnel: w100 -> [_ _ _ w130]
              tunnel: w99 -> [_ _ _ w129]
              frame "4" {
                w113 = 0.0 ("default (0 I32)")
                n24 = Decimal String To Number(string=w115, default (0L)=w113) -> (number=w112:dbl)  [unwired: 1 in, 1 out]
                n25 = Decimal String To Number(string=w114, default (0L)=w113) -> (number=w111:dbl)  [unwired: 1 in, 1 out]
                n26 = Bundle By Name(cluster=w118, "ICAO"=w116, "Speed"=w112, "Heading"=w111) -> (w117:T1)
              }
              frame Default {
              }
              frame "5", "7" {
                n27 = Decimal String To Number(string=w120, default (0L)=0.0 ("default (0 I32)")) -> ()  [unwired: 1 in, 2 out]
                n28 = Bundle By Name(cluster=w124, "ICAO"=w122, "Alt"=w120) -> (w123:T1)
              }
              frame "3" {
                w128 = 0.0 ("default (0 I32)")
                n29 = Decimal String To Number(string=w125, default (0L)=w128) -> ()  [unwired: 1 in, 2 out]
                n30 = Fract/Exp String To Number(string=w130, default (0 dbl)=w128) -> (number=w126:dbl)  [unwired: 2 in, 1 out]
                n31 = Fract/Exp String To Number(string=w129, default (0 dbl)=w128) -> (number=w127:dbl)  [unwired: 2 in, 1 out]
                n32 = Bundle By Name(cluster=w133, "ICAO"=w131, "Alt"=w125, "Latitude"=w126, "Longitude"=w127) -> (w132:T1)
              }
            }
            n33 = Replace Array Subset(array=w109, new element=w105, index=w108) -> (w110:T1[])
          }
        }
      }
      frame True {
      }
    }
  }
  "Airplanes" <- w7
  n34 = for {
    tunnel: w7 -> [w152] mode=indexing
    shift-right: [w141] -> w24
    shift-left: "" -> [w140]
    w151 = i16 6 ("width (-)")
    n35 = Unbundle By Name(w152) -> ("Latitude"=w148:dbl, "Longitude"=w147:dbl)
    n36 = Number To Fractional String(number=w147, width (-)=w151, precision (6)=w151) -> (F-format string=w144:string)  [unwired: 1 in]
    n37 = Number To Fractional String(number=w148, width (-)=i16 6, precision (6)=i16 6 ("width (-)")) -> (F-format string=w146:string)  [unwired: 1 in]
    n38 = Concatenate Strings("&markers=&markers=icon:https://icons.iconarchive.com/icons/unclebob/spanish-travel/24/plane-icon.png|" ("string"), w146, "," ("string"), w144) -> (w142:string)
    n39 = Concatenate Strings(w140, w142) -> (w141:string)
  }
  n40 = Concatenate Strings("https://maps.googleapis.com/maps/api/staticmap?center=" ("string"), "current lat", w27, "current lon", "&zoom=7&size=200x200&scale=2&maptype=roadmap" ("string"), "&markers=icon:https://icons.iconarchive.com/icons/icons8/windows-8/24/Transport-Prop-Plane-icon.png|" ("string"), "current lat", w27, "current lon", w24, "&key=AIzaSyBLVIRyOFRoOpmuxChHO5QT5_7M34SwGWA" ("string")) -> (w28:string)
  n41 = for {
    tunnel: w7 -> [w160] mode=indexing
    shift-right: [w162] -> w17
    shift-left: "" ("string") -> [w161]
    (unwired) TRUE
    n42 = Unbundle By Name(w160) -> ("ICAO"=w159:string, "Latitude"=w156:dbl, "Longitude"=w158:dbl, "Alt"=w157:string)
    n43 = Equal To 0?(x=w156) -> (x = 0?=w155:bool)
    n44 = Empty String/Path?(string/path=w157) -> (empty?=w154:bool)
    n45 = Or(x=w155, y=w154) -> (x .or. y?=w153:bool)
    n46 = case shown="False" w153 {
      tunnel: [w170 w182] -> w162
      tunnel: w161 -> [w169 w182]
      tunnel: w159 -> [w166 _]
      tunnel: w156 -> [w165 _]
      tunnel: w158 -> [w164 _]
      tunnel: w157 -> [w163 _]
      frame False {
        w173 = "," ("string")
        w181 = i16 6 ("width (-)")
        n47 = Number To Fractional String(number=w164, width (-)=w181, precision (6)=w181) -> (F-format string=w177:string)  [unwired: 1 in]
        n48 = Number To Fractional String(number=w165, width (-)=i16 6, precision (6)=i16 6 ("width (-)")) -> (F-format string=w175:string)  [unwired: 1 in]
        n49 = Concatenate Strings("{\"longitude\":" ("string"), w177, w173, "\"latitude\":" ("string"), w175, w173, "\"height\":" ("string"), w163, w173, "\"ICAO\":\"" ("string"), w166, "\"}" ("string")) -> (w167:string)
        n50 = Concatenate Strings(w169, "," ("string"), w167) -> (w170:string)
      }
      frame True {
        # "if lat/long are zero"
      }
    }
  }
  n51 = invoke class="IWebBrowser2" method="Refresh"(reference="Current Map") -> (reference out=w20:refnum<k7>)  [unwired: 2 in, 2 out]
  n52 = invoke class="IWebBrowser2" method="Navigate"(reference=w20, "URL"=w28) -> ()  [unwired: 6 in, 8 out]
  n53 = Index Array(array=w7) -> (element=w6:T1)  [unwired: 1 in]
  n54 = String Subset(string=w17, offset (0)=1) -> (substring=w16:string)  [unwired: 1 in]
  "string" <- w16
  n55 = Unbundle By Name(w6) -> ("Alt"=w5:string, "Heading"=w3:dbl, "Speed"=w2:dbl)
  n56 = disable-structure shown="Enabled" {
    disable-tunnel: w16 -> [w184 _]
    disable-tunnel: T2 {"ViewerLat"="40.286792", "ViewerLong"="-79.541260", "ViewerAlt"="1000", "ViewerHDG"="180", "Viewerpitch"="0"} ("ViewerData") -> [w183 _]
    frame Enabled {
      n57 = call "CreateCesTML.vi"("Traffic String"=w184, "ViewerData"=w183) -> ()  [unwired: 9 in, 1 out]
    }
    frame Disabled {
    }
  }
  n58 = Decimal String To Number(string=w5, default (0L)=0.0 ("default (0 I32)")) -> (number=w4:dbl)  [unwired: 1 in, 1 out]
  n59 = call "PlaneSpeed.vi"("GPS_Speed over Ground"=w2) -> ()  [unwired: 10 in, 1 out]
  n60 = call "PlaneAlt.vi"("Altitude [m]"=w4) -> ()  [unwired: 10 in, 1 out]
  n61 = Open VI Reference(vi path=path "C:/LauraLabVIEW/ADSB Tracker/SubVI/PlaneCompass.vi") -> (vi reference=w11:refnum<vi>)  [unwired: 5 in, 1 out]
  n62 = invoke class="VI" method="FP.Open"(reference=w11) -> (reference out=w8:refnum<vi>, error out=w10:errorcluster)  [unwired: 4 in, 3 out]
  n63 = call "PlaneCompass.vi"("error in (no error)"=w10, "GPS_Ground Course"=w3) -> ("error out"=w9:errorcluster)  [unwired: 9 in]
  n64 = Close Reference(reference=w8, error in (no error)=w9) -> ()  [unwired: 1 out]
